vi "RS_SMBV100A.vi"(4 "error in":T15, 7 "Command":T16) -> (0 "error out":T15, 3 "Response":T13)   [LabVIEW 2018]
uses:
  MOKO_LabViewLibrary/MokoLowLevel/MokoLowLovelControl/MLLC_Command.ctl
  MOKO_LabViewLibrary/MokoLowLevel/MokoLowLovelControl/MLLC_Error.ctl
  MOKO_LabViewLibrary/MokoLowLevel/MokoLowLovelControl/MLLC_Mode.ctl
  MOKO_LabViewLibrary/MokoLowLevel/MokoLowLovelControl/MLLC_Response.ctl
  MOKO_LabViewLibrary/MokoLowLevel/MokoLowLovelControl/MLLC_ConnectCluster.ctl
  MOKO_LabViewLibrary/MokoLowLevel/MokoLowLovelControl/MLLC_InterfaceType.ctl
  MOKO_LabViewLibrary/MokoLowLevel/MokoLowLovelControl/MLLC_OpenedSession.ctl
  MOKO_LabViewLibrary/MokoLowLevel/MokoLowLovelControl/MLLC_InterfaceSettings.ctl
  MOKO_LabViewLibrary/MokoLowLevel/MokoLowLovelControl/MLLC_InterfaceKind.ctl
  data/RS_SMBV100A_DynamWaypoints.ctl
  data/RS_SMBV100A_DynamWaypoint.ctl
  MOKO_LabViewLibrary/MokoLowLevel/MokoLowLovelControl/MLLC_DriverName.ctl
  MOKO_LabViewLibrary/MokoLowLevel/MokoLowLovelControl/MLLC_ErrorCode.ctl
  MOKO_LabViewLibrary/MokoLowLevel/MokoLowLovelControl/MLLC_ResponseInit.ctl
  MOKO_LabViewLibrary/MokoLowLevel/MokoLowLovelControl/MLLC_Request.ctl
panel:
  in  "Request":T1="*IDN?"
  in  "ResponseInit":T2="SMBV100A"
  in  "Error Code":T3=5450
  in  "Driver Name":T4="RS_SMBV100A"
  in  "Settings":T12={"Connect"={"InterfaceType"=enum."VISA", "OpenedSession"="COM1", "InterfaceSettings"={"Interface"=enum."RS232", "EOS 4 read"=enum."LF (\\n)", "EOS 4 write"=enum."LF (\\n)", "TMO, ms"=10000, "Sett"=variant(cluster{"Baud Rate":u32, "Data Bits":u16, "Parity":u16, "Stop Bits":u16, "Flow Control":u16, "Eho":bool} {"Baud Rate"=75, "Data Bits"=0, "Parity"=0, "Stop Bits"=0, "Flow Control"=0, "Eho"=FALSE})}}, "GPS SCENARIO"="****************************** MOVEMENT FILE ******************************\nRESOLUTION: 50\nREFERENCE: 11.583333,48.150,500\nSTART: 0, 0, 0, 10\nSTAY: 10000\nLINE: 200, 0, 0\nLINE: 100, 0, 19.6\nLINE: 600, 0, 0\nLINE: 100, 0, -19.6\nARC: 1000, 500, 180\nLINE: -200, 0, 0\nLINE: -100, 0, 19.6\nLINE: -600, 0, 0\nLINE: -100, 0, -19.6\nARC: 0, 500, 180", "GLONASS SCENARIO"="****************************** MOVEMENT FILE ******************************\nRESOLUTION: 50\nREFERENCE: 11.583333,48.150,500\nSTART: 0, 0, 0, 10\nSTAY: 10000\nLINE: 200, 0, 0\nLINE: 100, 0, 19.6\nLINE: 600, 0, 0\nLINE: 100, 0, -19.6\nARC: 1000, 500, 180\nLINE: -200, 0, 0\nLINE: -100, 0, 19.6\nLINE: -600, 0, 0\nLINE: -100, 0, -19.6\nARC: 0, 500, 180", "GPS WAYPOINTS"=[], "GLONASS WAYPOINTS"=[], "GALILOE SCENARIO"="****************************** MOVEMENT FILE ******************************\nRESOLUTION: 50\nREFERENCE: 11.583333,48.150,500\nSTART: 0, 0, 0, 10\nSTAY: 10000\nLINE: 200, 0, 0\nLINE: 100, 0, 19.6\nLINE: 600, 0, 0\nLINE: 100, 0, -19.6\nARC: 1000, 500, 180\nLINE: -200, 0, 0\nLINE: -100, 0, 19.6\nLINE: -600, 0, 0\nLINE: -100, 0, -19.6\nARC: 0, 500, 180", "GALILEO WAYPOINTS"=[], "GPS WAYPOINTS STRING"="", "BASEBAND"="GPS", "BEIDOU SCENARIO"="****************************** MOVEMENT FILE ******************************\nRESOLUTION: 50\nREFERENCE: 11.583333,48.150,500\nSTART: 0, 0, 0, 10\nSTAY: 10000\nLINE: 200, 0, 0\nLINE: 100, 0, 19.6\nLINE: 600, 0, 0\nLINE: 100, 0, -19.6\nARC: 1000, 500, 180\nLINE: -200, 0, 0\nLINE: -100, 0, 19.6\nLINE: -600, 0, 0\nLINE: -100, 0, -19.6\nARC: 0, 500, 180", "QZSS SCENARIO"="****************************** MOVEMENT FILE ******************************\nRESOLUTION: 50\nREFERENCE: 11.583333,48.150,500\nSTART: 0, 0, 0, 10\nSTAY: 10000\nLINE: 200, 0, 0\nLINE: 100, 0, 19.6\nLINE: 600, 0, 0\nLINE: 100, 0, -19.6\nARC: 1000, 500, 180\nLINE: -200, 0, 0\nLINE: -100, 0, 19.6\nLINE: -600, 0, 0\nLINE: -100, 0, -19.6\nARC: 0, 500, 180", "BEIDOU WAYPOINTS"=[], "SSDK WAYPOINTS"=[]} {"SSDK WAYPOINTS"."Time" format="%<%.3X>T"; "SSDK WAYPOINTS"."Speed" format="%#.10g"; "SSDK WAYPOINTS"."Heigth" format="%#.10g"; "SSDK WAYPOINTS"."Longitude" format="%#.10g"; "SSDK WAYPOINTS"."Latitude" format="%#.10g"; "BEIDOU WAYPOINTS"."Time" format="%<%.3X>T"; "BEIDOU WAYPOINTS"."Speed" format="%#.10g"; "BEIDOU WAYPOINTS"."Heigth" format="%#.10g"; "BEIDOU WAYPOINTS"."Longitude" format="%#.10g"; "BEIDOU WAYPOINTS"."Latitude" format="%#.10g"; "GALILEO WAYPOINTS"."Time" format="%<%.3X>T"; "GALILEO WAYPOINTS"."Speed" format="%#.10g"; "GALILEO WAYPOINTS"."Heigth" format="%#.10g"; "GALILEO WAYPOINTS"."Longitude" format="%#.10g"; "GALILEO WAYPOINTS"."Latitude" format="%#.10g"; "GLONASS WAYPOINTS"."Time" format="%<%.3X>T"; "GLONASS WAYPOINTS"."Speed" format="%#.10g"; "GLONASS WAYPOINTS"."Heigth" format="%#.10g"; "GLONASS WAYPOINTS"."Longitude" format="%#.10g"; "GLONASS WAYPOINTS"."Latitude" format="%#.10g"; "GPS WAYPOINTS"."Time" format="%<%.3X>T"; "GPS WAYPOINTS"."Speed" format="%#.10g"; "GPS WAYPOINTS"."Heigth" format="%#.10g"; "GPS WAYPOINTS"."Longitude" format="%#.10g"; "GPS WAYPOINTS"."Latitude" format="%#.10g"}
  in  "Mode":T14=enum."Check"
  # "RS_SMBV100A"
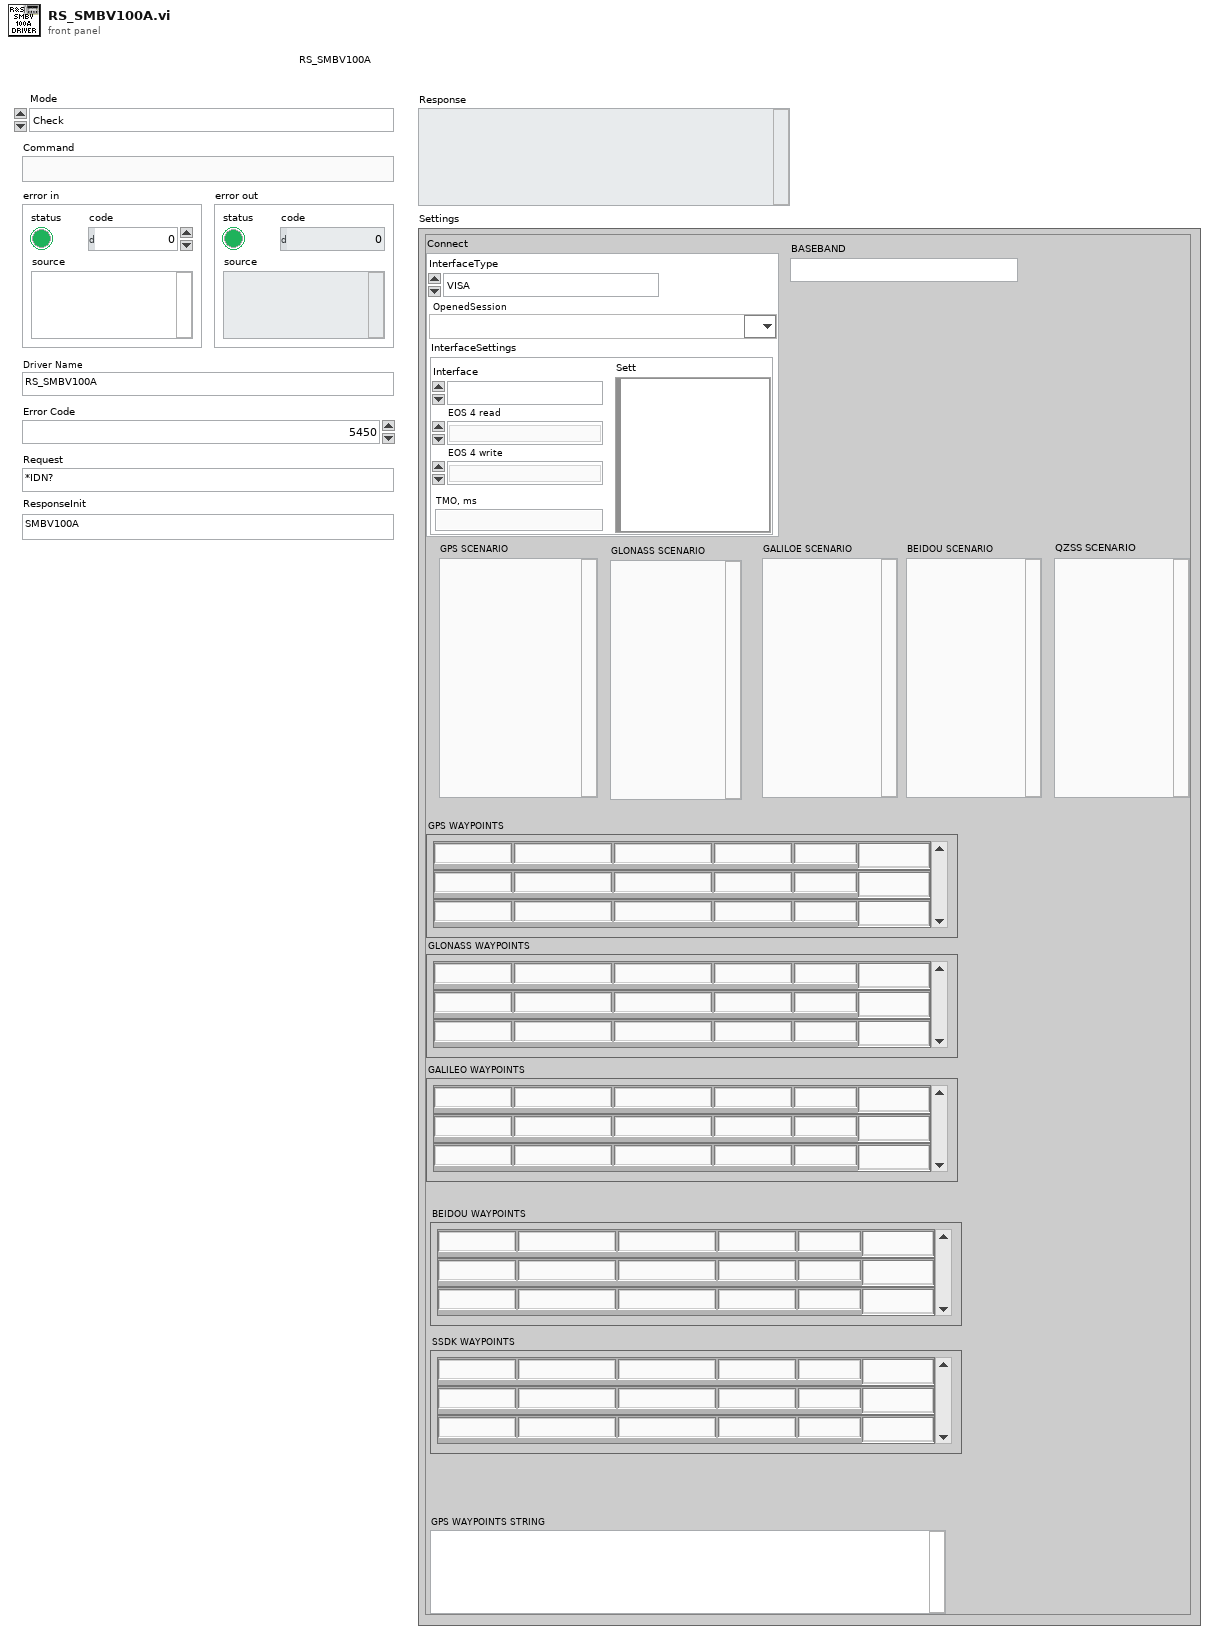
[diagram p1: front panel]
types:
  T1 = typedef "MLLC_Request.ctl" = string
  T2 = typedef "MLLC_ResponseInit.ctl" = string
  T3 = typedef "MLLC_ErrorCode.ctl" = u32
  T4 = typedef "MLLC_DriverName.ctl" = string
  T5 = typedef "MLLC_ConnectCluster.ctl" = cluster{"InterfaceType":T6, "OpenedSession":T7, "InterfaceSettings":T8}
  T6 = typedef "MLLC_InterfaceType.ctl" = enum16{"VISA", "Prologix USB-GPIB"}
  T7 = typedef "MLLC_OpenedSession.ctl" = refnum<visa-resource-name>
  T8 = typedef "MLLC_InterfaceSettings.ctl" = cluster{"Interface":T9, "EOS 4 read":enum16{"Default (=EOS 4 write)", "CR (\\r)", "LF (\\n)", "None"}, "EOS 4 write":enum16{"CR+LF (\\r\\n)", "CR (\\r)", "LF (\\n)", "None"}, "TMO, ms":i32, "Sett":variant}
  T9 = typedef "MLLC_InterfaceKind.ctl" = enum16{"RS232", "GPIB", "USB", "Ethernet", "another"}
  T10 = typedef "RS_SMBV100A_DynamWaypoints.ctl" = T11[]
  T11 = typedef "RS_SMBV100A_DynamWaypoint.ctl" = cluster{"Time":timestamp, "Latitude":ext, "Longitude":ext, "Heigth":dbl, "Speed":dbl, "Scenario":string}
  T12 = cluster{"Connect":T5, "GPS SCENARIO":string, "GLONASS SCENARIO":string, "GPS WAYPOINTS":T10, "GLONASS WAYPOINTS":T10, "GALILOE SCENARIO":string, "GALILEO WAYPOINTS":T10, "GPS WAYPOINTS STRING":string, "BASEBAND":string, "BEIDOU SCENARIO":string, "QZSS SCENARIO":string, "BEIDOU WAYPOINTS":T10, "SSDK WAYPOINTS":T10}
  T13 = typedef "MLLC_Response.ctl" = string
  T14 = typedef "MLLC_Mode.ctl" = enum16{"get", "set", "close", "Init", "Check"}
  T15 = typedef "MLLC_Error.ctl" = errorcluster
  T16 = typedef "MLLC_Command.ctl" = string
  T17 = enum16{"open", "replace", "create", "open or create", "replace or create", "replace or create with confirmation"}
  T18 = typedef "RS_SMBV100A_Parsing Satelite.ctl" = cluster{"Time":dbl[], "Sat":dbl[], "State":dbl[], "NUMBERINSKY":dbl[], "STANDART":string[]}
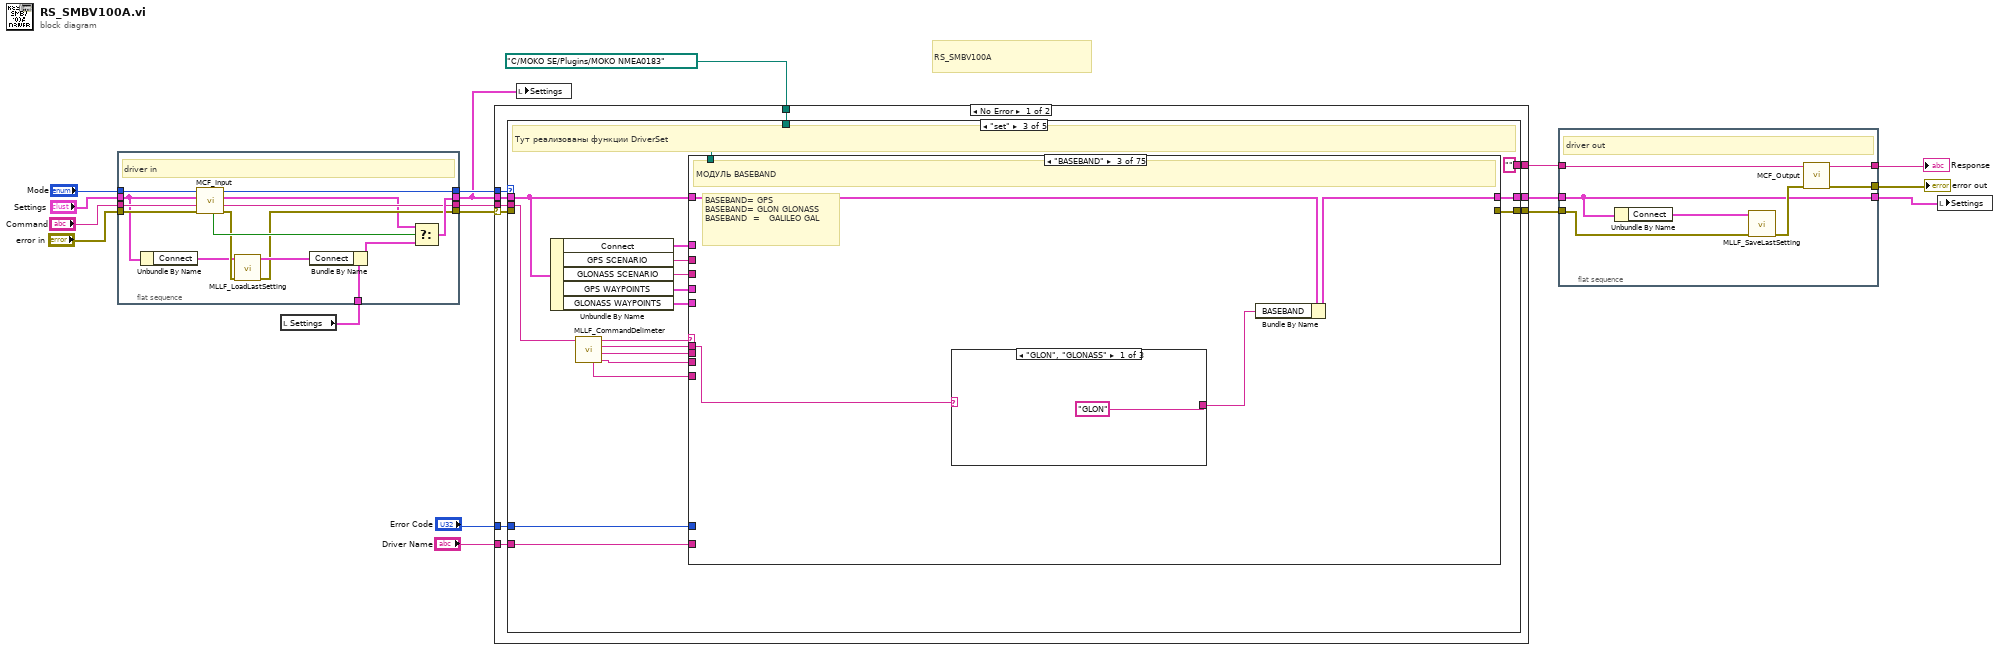
[diagram p0: block diagram]
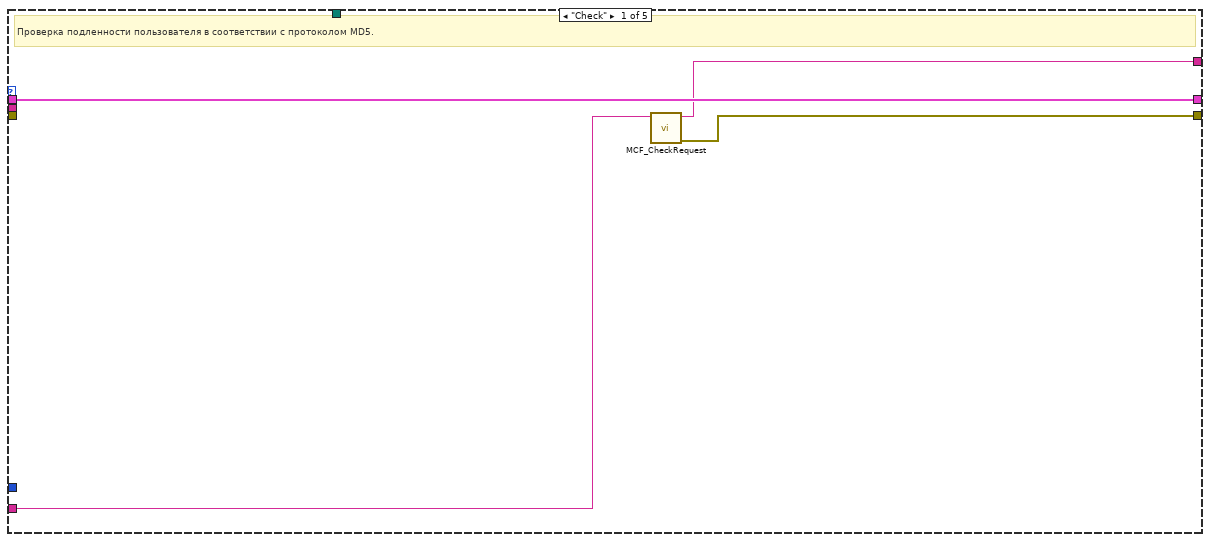
[diagram p2: hidden frame]
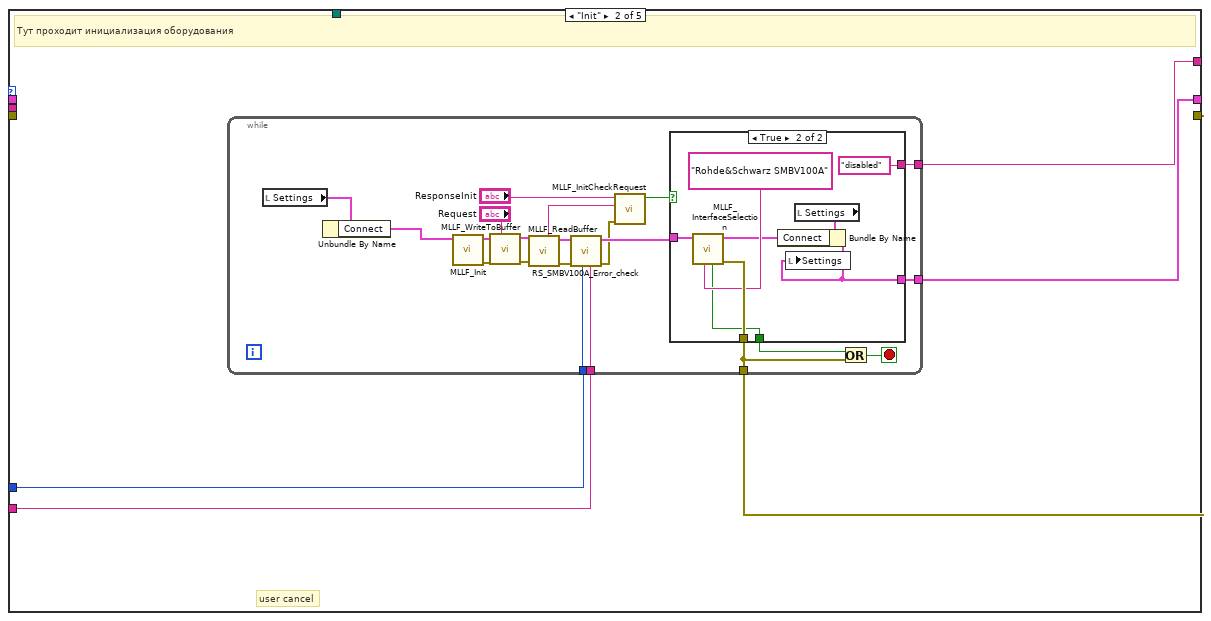
[diagram p3: hidden frame]
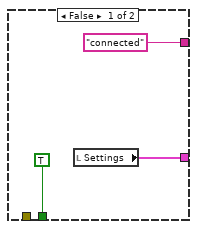
[diagram p4: hidden frame]
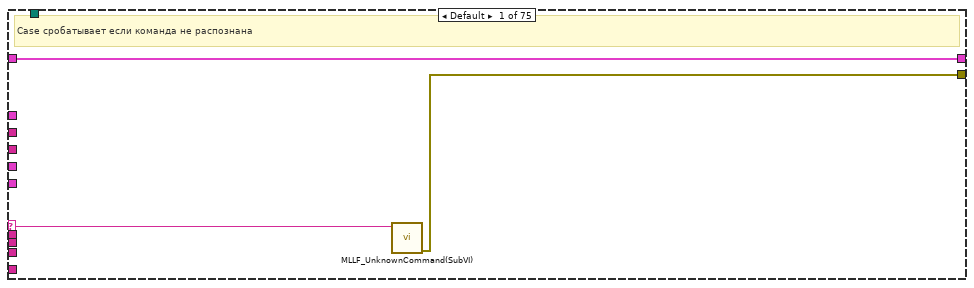
[diagram p5: hidden frame]
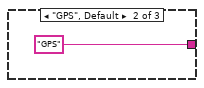
[diagram p7: hidden frame]
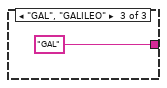
[diagram p8: hidden frame]
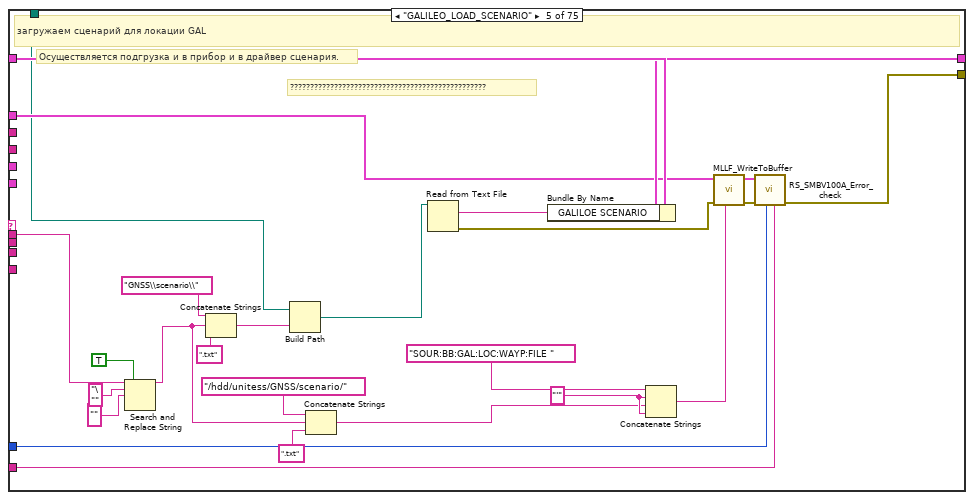
[diagram p10: hidden frame]
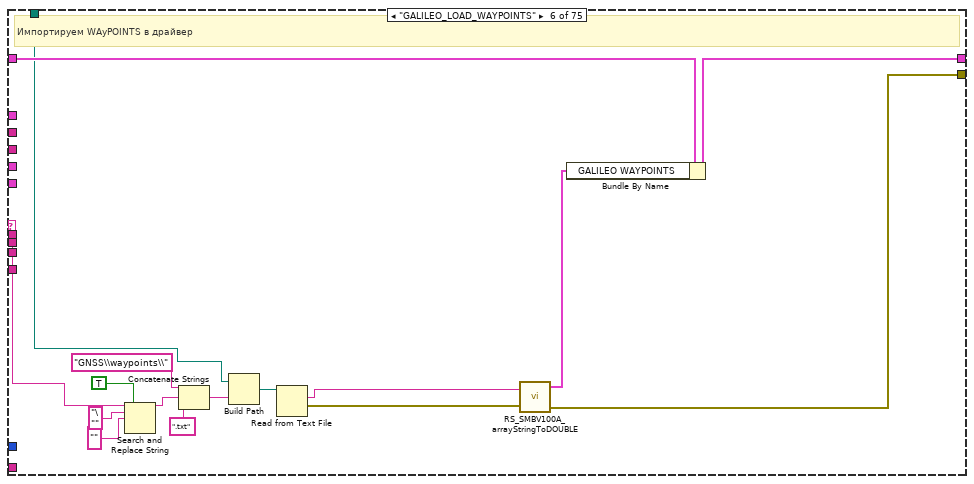
[diagram p11: hidden frame]
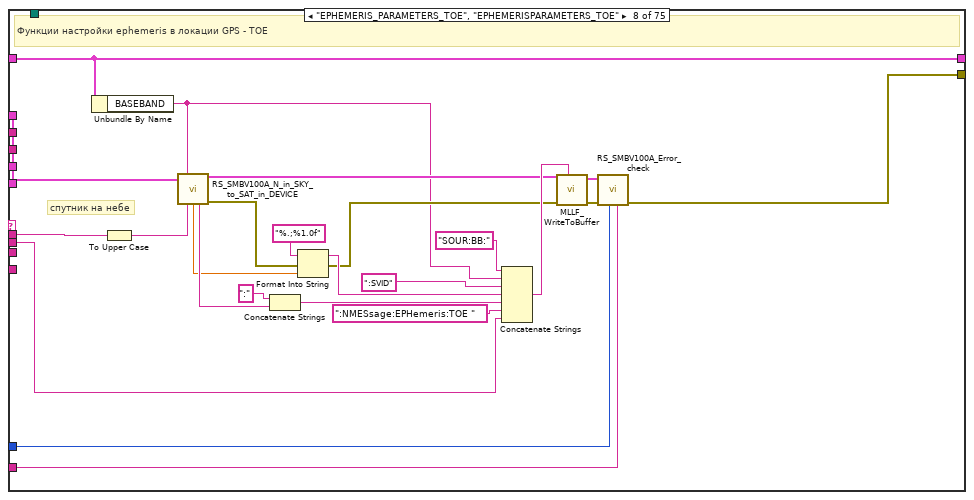
[diagram p13: hidden frame]
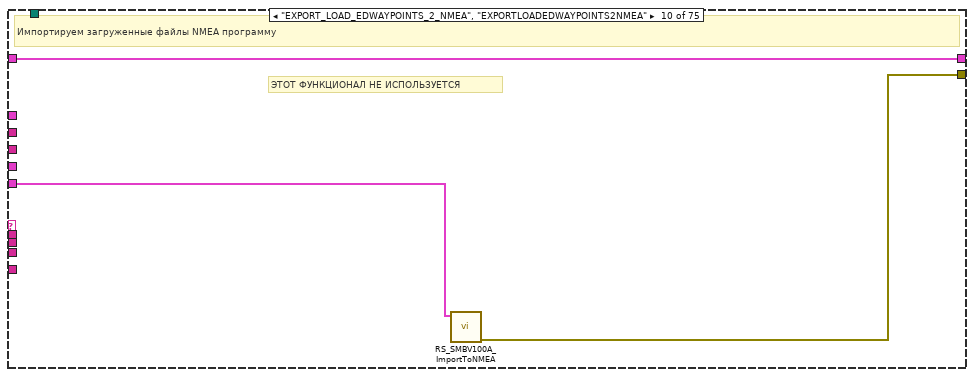
[diagram p15: hidden frame]
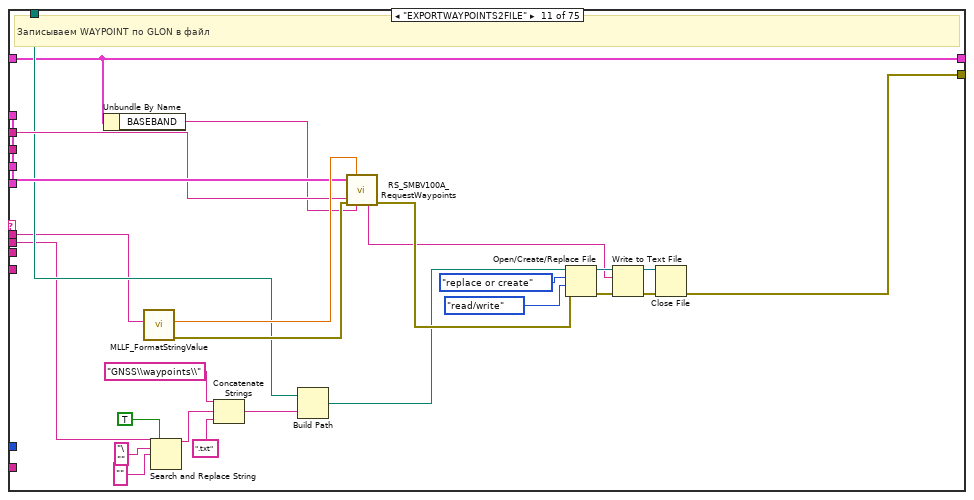
[diagram p16: hidden frame]
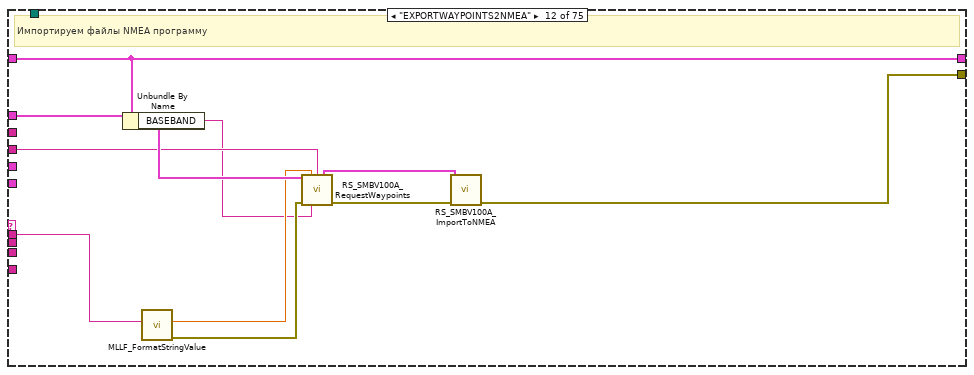
[diagram p17: hidden frame]
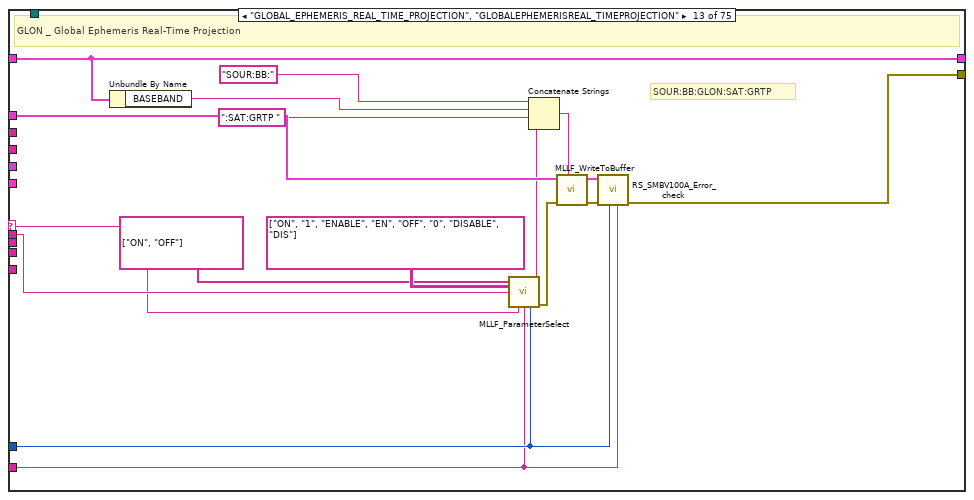
[diagram p18: hidden frame]
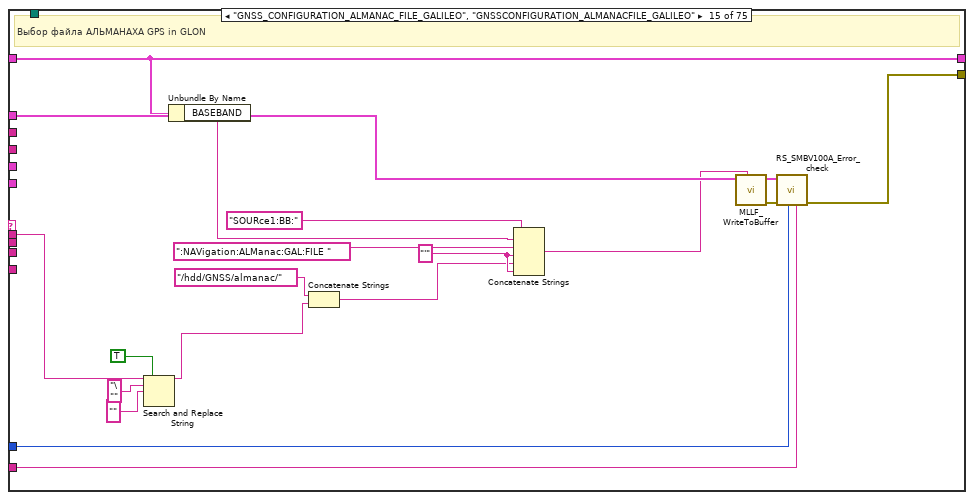
[diagram p20: hidden frame]
diagram:
  # "RS_SMBV100A"
  n1 = flat-sequence {
    tunnel: [w22] -> w3
    tunnel: [w32] -> w5
    tunnel: [w24] -> w2
    tunnel: "Command" -> [w25]
    tunnel: "Mode" -> [w27]
    tunnel: "Settings" -> [w20]
    tunnel: [w29] -> w4
    tunnel: w1 -> [w28]
    tunnel: "error in" -> [w21]
    frame #0 {
      # "driver in"
      n2 = Unbundle By Name(w20) -> ("Connect"=w19:T5)
      n3 = call "MCF_Input.vi"("Error In"=w21, "Command in"=w25, "Mode in"=w27) -> ("Error Out"=w23:errorcluster, "Command out"=w24:string, "Mode out"=w32:T14, "Boolean"=w26:bool)  [unwired: 5 in]
      n4 = call "MLLF_LoadLastSetting.vi"("Error In"=w23, "DriverConnectCluster in"=w19) -> ("Error Out"=w22:errorcluster, "DriverConnectCluster out"=w30:T5)  [unwired: 8 in]
      n5 = Bundle By Name(cluster=w28, "Connect"=w30) -> (w31:T12)
      n6 = Select(t=w20, s=w26, f=w31) -> (s? t:f=w29:T12)
    }
  }
  n7 = local read "Settings"() -> (w1:T12)
  n8 = case shown="No Error" w3 {
    selector: w3 -> [w39 w2026]
    tunnel: [w41 w2026] -> w13
    tunnel: w5 -> [w33 _]
    tunnel: [w42 _] -> w15
    tunnel: w2 -> [w40 _]
    tunnel: w4 -> [w36 w2025]
    tunnel: "Error Code" -> [w38 _]
    tunnel: "Driver Name" -> [w37 _]
    tunnel: [w35 w2025] -> w14
    tunnel: path "C:/MOKO SE/Plugins/MOKO NMEA0183" ("base path") -> [w34 _]
    frame No Error {
      n9 = case shown="\"set\"" w33 {
        tunnel: [w44 w47 "" ("Output String") w1143 "" ("Output String")] -> w42
        tunnel: [w43 w48 w100 w1142 w2023] -> w41
        tunnel: w40 -> [_ _ w101 w1155 _]
        tunnel: w39 -> [_ _ _ _ _]
        tunnel: w38 -> [_ w51 w99 w1152 _]
        tunnel: w37 -> [w45 w50 w96 w1151 _]
        tunnel: w36 -> [w46 _ w98 w1154 w2022]
        tunnel: [w46 w49 w97 w1153 w2022] -> w35
        tunnel: w34 -> [_ _ w95 _ _]
        frame "Check" {
          # "Проверка подленности пользователя в соответствии с протоколом MD5."
          n10 = call "MCF_CheckRequest.vi"("Driver Name"=w45) -> ("Error Out"=w43:errorcluster, "Output String"=w44:string)  [unwired: 9 in]
        }
        frame "Init" {
          # "user cancel"
          # "Тут проходит инициализация оборудования"
          n11 = while {
            tunnel: [w64] -> w48
            tunnel: w51 -> [w61]
            tunnel: w50 -> [w60]
            tunnel: [w57] -> w49
            tunnel: [w56] -> w47
            stop <- w63 stop-if-true
            n12 = local read "Settings"() -> (w67:T12)
            n13 = Unbundle By Name(w67) -> ("Connect"=w68:T5)
            n14 = call "MLLF_Init.vi"("DriverConnect in"=w68) -> ("Error Out"=w70:errorcluster, "DriverConnect out"=w69:T5)  [unwired: 7 in]
            n15 = call "MLLF_WriteToBuffer.vi"("String"="Request", "error in"=w70, "DriverConnect in"=w69) -> ("error out"=w72:T15, "DriverConnect out"=w71:T5)  [unwired: 5 in]
            n16 = call "MLLF_ReadBuffer.vi"("Error In"=w72, "DriverConnect in"=w71) -> ("Error Out"=w58:errorcluster, "DriverConnect out"=w59:T5, "String"=w54:string)  [unwired: 6 in]
            n17 = call "RS_SMBV100A_Error_check.vi"("Driver Name"=w60, "Error Code"=w61, "Error In"=w58, "DriverConnect in"=w59) -> ("Error Out"=w53:errorcluster, "DriverConnect out"=w62:T5)  [unwired: 6 in]
            n18 = call "MLLF_InitCheckRequest.vi"("error in (no error)"=w53, "Answer"=w54, "Response Init"="ResponseInit") -> ("Design"=w52:bool)  [unwired: 5 in, 3 out]
            n19 = case shown="True" w52 {
              tunnel: w62 -> [_ w82]
              tunnel: [TRUE w76] -> w65
              tunnel: [_ w83] -> w64
              tunnel: [w74 w78] -> w57
              tunnel: ["connected" "disabled"] -> w56
              frame False {
                n20 = local read "Settings"() -> (w74:T12)
              }
              frame True {
                n21 = call "MLLF_InterfaceSelection.vi"("Driver Name"="Rohde&Schwarz SMBV100A" ("String"), "DriverConnect in"=w82) -> ("error out"=w83:T15, "DriverConnect out"=w80:T5, "stop init?"=w76:bool)  [unwired: 5 in, 2 out]
                n22 = local read "Settings"() -> (w79:T12)
                n23 = Bundle By Name(cluster=w79, "Connect"=w80) -> (w78:T12)
                n24 = local write "Settings"(w78) -> ()
              }
            }
            n25 = Or(x=w65, y=w64) -> (x .or. y?=w63:bool)
          }
        }
        frame "set" {
          # "Тут реализованы функции DriverSet"
          n26 = Unbundle By Name(w98) -> ("Connect"=w93:T5, "GPS SCENARIO"=w92:string, "GLONASS SCENARIO"=w91:string, "GPS WAYPOINTS"=w90:T10, "GLONASS WAYPOINTS"=w89:T10)
          n27 = call "MLLF_CommandDelimeter.vi"("command with param"=w101) -> ("param 3"=w85:string, "param 2"=w86:string, "param 1"=w87:string, "command"=w88:string, "Spit delimetre"=w84:string)  [unwired: 6 in]
          n28 = case shown="\"BASEBAND\"" w88 {
            selector: w88 -> [w103 _ _ _ _ _ _ _ _ _ _ _ w221 _ _ _ _ _ _ _ w355 w372 w387 _ _ _ w447 _ w486 w503 w522 _ _ w575 _ _ _ w618 _ w655 _ w687 w703 _ _ w738 _ _ w807 _ w825 w842 w859 w876 _ _ w912 _ _ _ _ w975 _ _ _ _ _ _ _ _ _ w1080 _ _ _]
            tunnel: [w102 _ _ _ w129 w147 _ w176 _ w183 w199 w218 w229 _ w252 w271 w290 w309 w328 w347 w369 w386 w403 w419 w437 _ w455 w480 w494 w511 w536 w551 w564 w583 _ w603 w612 w626 w650 w665 w681 w696 w712 w726 _ w752 w773 w804 w815 _ w833 w850 w868 w884 w900 _ w920 w935 w947 _ w969 w991 _ w1006 w1025 _ w1040 w1047 w1056 w1064 w1072 w1082 w1100 w1108 w1118] -> w100
            tunnel: w99 -> [_ _ _ _ w128 _ _ w180 _ _ _ _ w234 _ w257 w276 w295 w314 w333 w352 w353 w370 w388 w418 _ _ w460 w485 w499 w516 w520 w556 w569 w573 _ w599 w617 w631 w654 w670 w686 w701 w717 w731 _ w736 w775 w806 w820 _ w838 w855 w872 w889 w905 _ w910 w934 w949 _ w974 w978 _ w1005 _ _ w1045 w1049 w1058 w1066 w1074 w1087 w1105 w1113 w1119]
            tunnel: w98 -> [w104 w105 w109 w113 w138 w151 w156 w163 w181 w184 w188 w212 w228 w238 w241 w261 w280 w297 w316 w335 w359 w376 w393 w428 w441 w446 w454 w469 w488 w505 w524 w539 w560 w577 w590 w594 w607 w620 w639 w657 w673 w690 w704 w722 w735 w740 w755 w778 w809 w824 w827 w844 w862 w878 w894 w909 w914 w930 w942 w953 w954 w979 w992 w1015 w1028 w1032 w1046 w1055 w1063 w1071 w1079 w1092 w1106 w1114 w1117]
            tunnel: [w104 w105 w108 w113 w137 w150 w156 w163 w181 w184 w188 w212 w228 w238 w241 w261 w280 w297 w316 w335 w359 w376 w393 w427 w440 w446 w454 w469 w488 w505 w524 w539 w560 w577 w590 w594 w607 w620 w639 w657 w673 w690 w704 w722 w735 w740 w755 w778 w809 w824 w827 w844 w862 w878 w894 w909 w914 w930 w942 w953 w954 w979 w992 w1014 w1027 w1032 w1046 w1055 w1063 w1071 w1079 w1092 w1106 w1114 w1116] -> w97
            tunnel: w93 -> [_ _ _ _ w131 _ _ w175 _ _ w208 w220 w232 _ w255 w274 w293 w312 w331 w350 w363 w380 w397 w421 _ _ w458 w483 w497 w514 w530 w554 w567 w584 _ w606 w615 w629 w649 w668 w684 w699 w715 w729 _ w748 w772 w803 w818 _ w836 w853 w871 w887 w903 _ w921 w936 w950 _ w972 w987 _ w1008 _ _ w1043 w1050 w1059 w1067 w1075 w1085 w1103 w1111 _]
            tunnel: w96 -> [_ _ _ _ w127 _ _ w179 _ _ _ _ w233 _ w256 w275 w294 w313 w332 w351 w354 w371 w389 w417 _ _ w459 w484 w498 w515 w521 w555 w568 w574 _ w600 w616 w630 w653 w669 w685 w700 w716 w730 _ w737 w774 w805 w819 _ w837 w854 w860 w888 w904 _ w911 w933 w948 _ w973 w977 _ w1004 _ _ w1044 w1048 w1057 w1065 w1073 w1086 w1104 w1112 w1120]
            tunnel: w87 -> [_ _ w106 _ w116 w141 _ w158 _ _ w186 w217 w222 _ w243 w263 w282 w300 w319 w338 w356 w373 w390 w406 w431 _ w448 w466 w487 w504 w523 w541 w557 w576 _ w591 _ w619 w636 w656 w672 _ _ w719 _ w739 w759 w783 w808 _ w826 w843 w861 w877 w893 _ w913 w927 _ _ w960 w976 _ w994 w1020 _ w1036 _ _ _ _ w1081 w1096 _ w1115]
            tunnel: w92 -> [_ _ _ _ _ _ _ _ _ _ w194 _ _ _ _ _ _ _ _ _ _ _ _ _ _ _ _ _ _ _ _ _ _ _ _ _ _ _ _ _ _ _ _ _ _ _ _ _ _ _ _ _ _ _ _ _ _ _ _ _ _ _ _ _ _ _ _ _ _ _ _ _ _ _ _]
            tunnel: w91 -> [_ _ _ _ _ _ _ _ _ _ _ w214 _ _ _ _ _ _ _ _ _ _ _ _ _ _ _ _ _ _ _ _ _ _ _ _ _ _ _ _ _ _ _ _ _ _ _ _ _ _ _ _ _ _ _ _ _ _ _ _ _ _ _ _ _ _ _ _ _ _ _ _ _ _ _]
            tunnel: w90 -> [_ _ _ _ _ _ _ _ _ _ _ _ _ _ _ _ _ _ _ _ _ _ _ _ _ _ _ _ _ _ _ _ _ _ _ _ _ _ _ _ _ _ _ _ _ _ _ _ _ _ _ _ _ _ _ _ _ _ _ _ _ _ _ _ _ _ _ _ _ _ _ _ _ _ _]
            tunnel: w89 -> [_ _ _ _ _ _ _ _ _ w182 _ _ _ _ _ _ _ _ _ _ _ _ _ _ _ _ _ _ _ _ _ _ _ _ _ _ _ _ _ _ _ _ _ _ _ _ _ _ _ _ _ _ _ _ _ _ _ _ _ _ _ _ _ _ _ _ _ _ _ _ _ _ _ _ _]
            tunnel: w95 -> [_ _ _ _ w114 w140 _ _ _ _ w189 _ _ _ _ _ _ _ _ _ _ _ _ w404 w430 _ _ _ _ _ _ _ _ _ _ _ _ _ _ _ _ _ _ _ _ _ _ _ _ _ _ _ _ _ _ _ _ _ _ _ _ _ _ w993 w1017 _ _ _ _ _ _ _ _ _ _]
            tunnel: w86 -> [_ _ _ _ _ _ _ w157 _ _ w185 _ _ _ _ _ _ _ _ _ _ _ _ _ _ _ _ w465 _ _ _ _ _ _ _ _ _ _ w635 _ _ _ _ _ _ _ _ _ _ _ _ _ _ _ _ _ _ _ _ _ _ _ _ _ _ _ _ _ _ _ _ _ _ _ _]
            tunnel: w85 -> [_ _ _ _ _ _ _ _ _ _ _ _ _ _ _ _ _ _ _ _ _ _ _ _ _ _ _ w464 _ _ _ _ _ _ _ _ _ _ _ _ _ _ _ _ _ _ _ _ _ _ _ _ _ _ _ _ _ _ _ _ _ _ _ _ _ _ _ _ _ _ _ _ _ _ _]
            tunnel: w84 -> [_ _ _ _ _ _ _ _ _ _ _ _ _ _ _ _ _ _ _ _ _ _ _ _ _ _ _ _ _ _ _ _ _ _ _ _ _ _ _ _ _ _ _ _ _ _ _ _ _ _ _ _ _ _ _ _ _ _ _ _ _ _ _ _ _ _ _ _ _ _ _ _ _ w1107 _]
            frame Default {
              # "Case сробатывает если команда не распознана"
              n29 = call "MLLF_UnknownCommand(SubVI).vi"("Unknown command"=w103) -> ("error out"=w102:errorcluster)  [unwired: 10 in]
            }
            frame "----- BASEBAND -----" {
              # "МОДУЛЬ BASEBAND"
            }
            frame "BASEBAND" {
              # "BASEBAND= GPS\nBASEBAND= GLON GLONASS\nBASEBAND  =   GALILEO GAL"
              # "МОДУЛЬ BASEBAND"
              n30 = case shown="\"GLON\", \"GLONASS\"" w106 {
                tunnel: ["GLON" ("regular expression") "GPS" "GAL" ("regular expression")] -> w107
                frame "GLON", "GLONASS" {
                }
                frame "GPS", Default {
                }
                frame "GAL", "GALILEO" {
                }
              }
              n31 = Bundle By Name(cluster=w109, "BASEBAND"=w107) -> (w108:T12)
            }
            frame "----GALILEO BASEBAND----" {
            }
            frame "GALILEO_LOAD_SCENARIO" {
              w135 = "'" ("string")
              # "?????????????????????????????????????????????????"
              # "Осуществляется подгрузка и в прибор и в драйвер сценария."
              # "загружаем сценарий для локации GAL"
              n32 = Search and Replace String(replace all?=TRUE, input string=w116, search string="\"", replace string="") -> (result string=w115:string)  [unwired: 4 in, 3 out]
              n33 = Concatenate Strings("GNSS\\scenario\\", w115, ".txt") -> (w125:string)
              n34 = Build Path(base path=w114, name or relative path=w125) -> (appended path=w120:path)
              n35 = Concatenate Strings("/hdd/unitess/GNSS/scenario/", w115, ".txt") -> (w121:string)
              n36 = Read from Text File(file (use dialog)=w120) -> (text=w139:string, error out=w130:errorcluster)  [unwired: 3 in, 2 out]
              n37 = Bundle By Name(cluster=w138, "GALILOE SCENARIO"=w139) -> (w137:T12)
              n38 = Concatenate Strings("SOUR:BB:GAL:LOC:WAYP:FILE " ("string"), w135, w121, w135) -> (w132:string)
              n39 = call "MLLF_WriteToBuffer.vi"("String"=w132, "error in"=w130, "DriverConnect in"=w131) -> ("error out"=w133:T15, "DriverConnect out"=w134:T5)  [unwired: 5 in]
              n40 = call "RS_SMBV100A_Error_check.vi"("Driver Name"=w127, "Error Code"=w128, "Error In"=w133, "DriverConnect in"=w134) -> ("Error Out"=w129:errorcluster)  [unwired: 6 in, 1 out]
            }
            frame "GALILEO_LOAD_WAYPOINTS" {
              # "Импортируем WAyPOINTS в драйвер"
              n41 = Search and Replace String(replace all?=TRUE, input string=w141, search string="\"", replace string="") -> (result string=w142:string)  [unwired: 4 in, 3 out]
              n42 = Concatenate Strings("GNSS\\waypoints\\", w142, ".txt") -> (w154:string)
              n43 = Build Path(base path=w140, name or relative path=w154) -> (appended path=w152:path)
              n44 = Read from Text File(file (use dialog)=w152) -> (text=w149:string, error out=w148:errorcluster)  [unwired: 3 in, 2 out]
              n45 = call "RS_SMBV100A_arrayStringToDOUBLE.vi"("string"=w149, "error in"=w148) -> ("Dynam waypoints"=w146:T10, "error out"=w147:errorcluster)  [unwired: 1 in]
              n46 = Bundle By Name(cluster=w151, "GALILEO WAYPOINTS"=w146) -> (w150:T12)
            }
            frame "---- GLONASS BASEBAND -----" {
              # "Функции настройки в локации GLONASS"
            }
            frame "EPHEMERIS_PARAMETERS_TOE", "EPHEMERISPARAMETERS_TOE" {
              # "спутник на небе"
              # "Функции настройки ephemeris в локации GPS - TOE"
              n47 = Unbundle By Name(w163) -> ("BASEBAND"=w160:string)
              n48 = To Upper Case(1:w158) -> (0:w159:string)
              n49 = call "RS_SMBV100A_N_in_SKY_to_SAT_in_DEVICE.vi"("DriverConnect in"=w175, "BASEBAND"=w160, "String Value"=w159) -> ("GNSS"=w167:string, "DriverConnect out"=w171:T5, "SATINSKY_for_DEVICE"=w164:dbl, "Error Out"=w170:errorcluster)  [unwired: 8 in, 1 out]
              n50 = Concatenate Strings(":" ("regular expression"), w167) -> (w166:string)
              n51 = Format Into String(format string="%.;%1.0f" ("format"), error in=w170, w164) -> (resulting string=w173:string, error out=w169:errorcluster)  [unwired: 1 in]
              n52 = Concatenate Strings("SOUR:BB:" ("regular expression"), w160, ":SVID" ("regular expression"), w173, w166, ":NMESsage:EPHemeris:TOE " ("regular expression"), w157) -> (w172:string)
              n53 = call "MLLF_WriteToBuffer.vi"("String"=w172, "error in"=w169, "DriverConnect in"=w171) -> ("error out"=w177:T15, "DriverConnect out"=w178:T5)  [unwired: 5 in]
              n54 = call "RS_SMBV100A_Error_check.vi"("Driver Name"=w179, "Error Code"=w180, "Error In"=w177, "DriverConnect in"=w178) -> ("Error Out"=w176:errorcluster)  [unwired: 6 in, 1 out]
            }
            frame "---------------------------- EXPORT ----------------------------------" {
            }
            frame "EXPORT_LOAD_EDWAYPOINTS_2_NMEA", "EXPORTLOADEDWAYPOINTS2NMEA" {
              # "ЭТОТ ФУНКЦИОНАЛ НЕ ИСПОЛЬЗУЕТСЯ"
              # "Импортируем загруженные файлы NMEA программу"
              n55 = call "RS_SMBV100A_ImportToNMEA.vi"("Dynam waypoints"=w182) -> ("error out"=w183:errorcluster)  [unwired: 10 in]
            }
            frame "EXPORTWAYPOINTS2FILE" {
              # "Записываем WAYPOINT по GLON в файл"
              n56 = Unbundle By Name(w188) -> ("BASEBAND"=w187:string)
              n57 = call "MLLF_FormatStringValue.vi"("String Value"=w186) -> ("error out"=w209:T15, "number"=w210:dbl)  [unwired: 8 in, 1 out]
              n58 = Search and Replace String(replace all?=TRUE, input string=w185, search string="\"", replace string="") -> (result string=w190:string)  [unwired: 4 in, 3 out]
              n59 = Concatenate Strings("GNSS\\waypoints\\", w190, ".txt") -> (w197:string)
              n60 = Build Path(base path=w189, name or relative path=w197) -> (appended path=w196:path)
              n61 = call "RS_SMBV100A_RequestWaypoints.vi"("DriverConnect in"=w208, "scenario time, c"=w210, "Error In"=w209, "BASEBAND"=w187, "Scenario in"=w194) -> ("Waypoints, txt"=w200:string, "Error Out"=w201:errorcluster)  [unwired: 7 in, 2 out]
              n62 = Open/Create/Replace File(file path (use dialog)=w196, error in=w201, operation (0:open)=T17."replace or create", access (0:read/write)=enum16{"read/write", "read-only", "write-only"}."read/write") -> (refnum out=w205:refnum<file>, error out=w202:errorcluster)  [unwired: 2 in, 1 out]
              n63 = Write to Text File(file (use dialog)=w205, text=w200, error in=w202) -> (refnum out=w203:refnum<file>, error out=w204:errorcluster)  [unwired: 1 in, 1 out]
              n64 = Close File(refnum=w203, error in=w204) -> (error out=w199:errorcluster)  [unwired: 1 out]
            }
            frame "EXPORTWAYPOINTS2NMEA" {
              # "Импортируем файлы NMEA программу"
              n65 = Unbundle By Name(w212) -> ("BASEBAND"=w211:string)
              n66 = call "MLLF_FormatStringValue.vi"("String Value"=w217) -> ("error out"=w215:T15, "number"=w216:dbl)  [unwired: 8 in, 1 out]
              n67 = call "RS_SMBV100A_RequestWaypoints.vi"("DriverConnect in"=w220, "scenario time, c"=w216, "Error In"=w215, "BASEBAND"=w211, "Scenario in"=w214) -> ("Dynam waypoints"=w213:T10, "Error Out"=w219:errorcluster)  [unwired: 7 in, 2 out]
              n68 = call "RS_SMBV100A_ImportToNMEA.vi"("error in"=w219, "Dynam waypoints"=w213) -> ("error out"=w218:errorcluster)  [unwired: 9 in]
            }
            frame "GLOBAL_EPHEMERIS_REAL_TIME_PROJECTION", "GLOBALEPHEMERISREAL_TIMEPROJECTION" {
              # "SOUR:BB:GLON:SAT:GRTP"
              # "GLON _ Global Ephemeris Real-Time Projection"
              n69 = Unbundle By Name(w228) -> ("BASEBAND"=w226:string)
              n70 = call "MLLF_ParameterSelect.vi"("Command to equipment"=string[] ["ON", "OFF"], "Names"=string[][] [["ON", "1", "ENABLE", "EN"], ["OFF", "0", "DISABLE", "DIS"]], "Input"=w222, "Command"=w221, "Driver Name"=w233, "Error Code"=w234) -> ("Choice"=w224:string, "Error Out"=w235:errorcluster)  [unwired: 8 in]
              n71 = Concatenate Strings("SOUR:BB:", w226, ":SAT:GRTP ", w224) -> (w223:string)
              n72 = call "MLLF_WriteToBuffer.vi"("String"=w223, "error in"=w235, "DriverConnect in"=w232) -> ("error out"=w230:T15, "DriverConnect out"=w231:T5)  [unwired: 5 in]
              n73 = call "RS_SMBV100A_Error_check.vi"("Driver Name"=w233, "Error Code"=w234, "Error In"=w230, "DriverConnect in"=w231) -> ("Error Out"=w229:errorcluster)  [unwired: 6 in, 1 out]
            }
            frame "---------------------- GNSS_CONFIGURATION ---------------------------------" {
            }
            frame "GNSS_CONFIGURATION_ALMANAC_FILE_GALILEO", "GNSSCONFIGURATION_ALMANACFILE_GALILEO" {
              w249 = "'" ("string")
              # "Выбор файла АЛЬМАНАХА GPS in GLON"
              n74 = Search and Replace String(replace all?=TRUE, input string=w243, search string="\"", replace string="") -> (result string=w242:string)  [unwired: 4 in, 3 out]
              n75 = Unbundle By Name(w241) -> ("BASEBAND"=w240:string)
              n76 = Concatenate Strings("/hdd/GNSS/almanac/" ("string"), w242) -> (w247:string)
              n77 = Concatenate Strings("SOURce1:BB:" ("string"), w240, ":NAVigation:ALManac:GAL:FILE " ("string"), w249, w247, w249) -> (w250:string)
              n78 = call "MLLF_WriteToBuffer.vi"("String"=w250, "DriverConnect in"=w255) -> ("error out"=w253:T15, "DriverConnect out"=w254:T5)  [unwired: 6 in]
              n79 = call "RS_SMBV100A_Error_check.vi"("Driver Name"=w256, "Error Code"=w257, "Error In"=w253, "DriverConnect in"=w254) -> ("Error Out"=w252:errorcluster)  [unwired: 6 in, 1 out]
            }
            frame "GNSS_CONFIGURATION_ALMANAC_FILE_GLONASS", "GNSSCONFIGURATION_ALMANACFILE_GLONASS" {
              w269 = "'" ("string")
              # "Выбор файла АЛЬМАНАХА Glonas in GLON"
              n80 = Search and Replace String(replace all?=TRUE, input string=w263, search string="\"", replace string="") -> (result string=w262:string)  [unwired: 4 in, 3 out]
              n81 = Unbundle By Name(w261) -> ("BASEBAND"=w260:string)
              n82 = Concatenate Strings("/hdd/GNSS/almanac/" ("string"), w262) -> (w267:string)
              n83 = Concatenate Strings("SOURce1:BB:" ("string"), w260, ":NAVigation:ALManac:GLON:FILE " ("string"), w269, w267, w269) -> (w270:string)
              n84 = call "MLLF_WriteToBuffer.vi"("String"=w270, "DriverConnect in"=w274) -> ("error out"=w272:T15, "DriverConnect out"=w273:T5)  [unwired: 6 in]
              n85 = call "RS_SMBV100A_Error_check.vi"("Driver Name"=w275, "Error Code"=w276, "Error In"=w272, "DriverConnect in"=w273) -> ("Error Out"=w271:errorcluster)  [unwired: 6 in, 1 out]
            }
            frame "GNSS_CONFIGURATION_ALMANAC_FILE_GPS", "GNSSCONFIGURATION_ALMANACFILE_GPS" {
              w288 = "'" ("string")
              # "Выбор файла АЛЬМАНАХА GPS in GLON"
              n86 = Search and Replace String(replace all?=TRUE, input string=w282, search string="\"", replace string="") -> (result string=w281:string)  [unwired: 4 in, 3 out]
              n87 = Concatenate Strings("/hdd/GNSS/almanac/" ("string"), w281) -> (w286:string)
              n88 = Unbundle By Name(w280) -> ("BASEBAND"=w278:string)
              n89 = Concatenate Strings("SOURce1:BB:" ("string"), w278, ":NAVigation:ALManac:GPS:FILE " ("string"), w288, w286, w288) -> (w289:string)
              n90 = call "MLLF_WriteToBuffer.vi"("String"=w289, "DriverConnect in"=w293) -> ("error out"=w291:T15, "DriverConnect out"=w292:T5)  [unwired: 6 in]
              n91 = call "RS_SMBV100A_Error_check.vi"("Driver Name"=w294, "Error Code"=w295, "Error In"=w291, "DriverConnect in"=w292) -> ("Error Out"=w290:errorcluster)  [unwired: 6 in, 1 out]
            }
            frame "GNSS_CONFIGURATION_RINEX_FILE_GAL", "GNSSCONFIGURATION_RINEXFILE_GAL" {
              w306 = "'" ("string")
              # "Выбор файла GPS RINEX GLON"
              n92 = Search and Replace String(replace all?=TRUE, input string=w300, search string="\"", replace string="") -> (result string=w299:string)  [unwired: 4 in, 3 out]
              n93 = Concatenate Strings("/hdd/GNSS/rinex/" ("string"), w299) -> (w304:string)
              n94 = Unbundle By Name(w297) -> ("BASEBAND"=w298:string)
              n95 = Concatenate Strings("SOURce1:BB:" ("string"), w298, ":RIN:ALM:GAL:FILE " ("string"), w306, w304, w306) -> (w307:string)
              n96 = call "MLLF_WriteToBuffer.vi"("String"=w307, "DriverConnect in"=w312) -> ("error out"=w310:T15, "DriverConnect out"=w311:T5)  [unwired: 6 in]
              n97 = call "RS_SMBV100A_Error_check.vi"("Driver Name"=w313, "Error Code"=w314, "Error In"=w310, "DriverConnect in"=w311) -> ("Error Out"=w309:errorcluster)  [unwired: 6 in, 1 out]
            }
            frame "GNSS_CONFIGURATION_RINEXFILE_GLONASS", "GNSSCONFIGURATION_RINEXFILE_GLONASS" {
              w325 = "'" ("string")
              # "Выбор файла GPS RINEX GLON"
              n98 = Search and Replace String(replace all?=TRUE, input string=w319, search string="\"", replace string="") -> (result string=w318:string)  [unwired: 4 in, 3 out]
              n99 = Concatenate Strings("/hdd/GNSS/rinex/" ("string"), w318) -> (w323:string)
              n100 = Unbundle By Name(w316) -> ("BASEBAND"=w317:string)
              n101 = Concatenate Strings("SOURce1:BB:" ("string"), w317, ":RIN:ALM:GLON:FILE " ("string"), w325, w323, w325) -> (w326:string)
              n102 = call "MLLF_WriteToBuffer.vi"("String"=w326, "DriverConnect in"=w331) -> ("error out"=w329:T15, "DriverConnect out"=w330:T5)  [unwired: 6 in]
              n103 = call "RS_SMBV100A_Error_check.vi"("Driver Name"=w332, "Error Code"=w333, "Error In"=w329, "DriverConnect in"=w330) -> ("Error Out"=w328:errorcluster)  [unwired: 6 in, 1 out]
            }
            frame "GNSS_CONFIGURATION_RINEX_FILE_GPS", "GNSSCONFIGURATION_RINEXFILE_GPS" {
              w344 = "'" ("string")
              # "Выбор файла GPS RINEX GLON"
              n104 = Search and Replace String(replace all?=TRUE, input string=w338, search string="\"", replace string="") -> (result string=w337:string)  [unwired: 4 in, 3 out]
              n105 = Concatenate Strings("/hdd/GNSS/rinex/" ("string"), w337) -> (w342:string)
              n106 = Unbundle By Name(w335) -> ("BASEBAND"=w336:string)
              n107 = Concatenate Strings("SOURce1:BB:" ("string"), w336, ":RIN:ALM:GPS:FILE " ("string"), w344, w342, w344) -> (w345:string)
              n108 = call "MLLF_WriteToBuffer.vi"("String"=w345, "DriverConnect in"=w350) -> ("error out"=w348:T15, "DriverConnect out"=w349:T5)  [unwired: 6 in]
              n109 = call "RS_SMBV100A_Error_check.vi"("Driver Name"=w351, "Error Code"=w352, "Error In"=w348, "DriverConnect in"=w349) -> ("Error Out"=w347:errorcluster)  [unwired: 6 in, 1 out]
            }
            frame "GNSS_CONFIGURATION_RINEX_FILE_GAL_STATE", "GNSSCONFIGURATION_RINEXFILE_GAL_STATE" {
              # "SOUR:BB:GLON:NAV:RIN:GAL:STAT OFF"
              # "Активировать\\Деактивировать GPS файла RINEX GLON"
              n110 = Unbundle By Name(w359) -> ("BASEBAND"=w361:string)
              n111 = call "MLLF_ParameterSelect.vi"("Command to equipment"=string[] ["ON\n", "OFF"], "Names"=string[][] [["ON", "1", "ENABLE", "EN"], ["OFF", "0", "DISABLE", "DIS"]], "Input"=w356, "Command"=w355, "Driver Name"=w354, "Error Code"=w353) -> ("Choice"=w358:string, "Error Out"=w366:errorcluster)  [unwired: 8 in]
              n112 = Concatenate Strings("SOUR:BB:", w361, ":NAV:RIN:GAL:STAT ", w358) -> (w357:string)
              n113 = call "MLLF_WriteToBuffer.vi"("String"=w357, "error in"=w366, "DriverConnect in"=w363) -> ("error out"=w364:T15, "DriverConnect out"=w365:T5)  [unwired: 5 in]
              n114 = call "RS_SMBV100A_Error_check.vi"("Driver Name"=w354, "Error Code"=w353, "Error In"=w364, "DriverConnect in"=w365) -> ("Error Out"=w369:errorcluster)  [unwired: 6 in, 1 out]
            }
            frame "GNSS_CONFIGURATION_RINEX_FILE_GLONASS_STATE", "GNSSCONFIGURATION_RINEXFILE_GLONASS_STATE" {
              # "SOUR:BB:GLON:NAV:RIN:GAL:STAT OFF"
              # "Активировать\\Деактивировать GPS файла RINEX GLON"
              n115 = Unbundle By Name(w376) -> ("BASEBAND"=w378:string)
              n116 = call "MLLF_ParameterSelect.vi"("Command to equipment"=string[] ["ON\n", "OFF"], "Names"=string[][] [["ON", "1", "ENABLE", "EN"], ["OFF", "0", "DISABLE", "DIS"]], "Input"=w373, "Command"=w372, "Driver Name"=w371, "Error Code"=w370) -> ("Choice"=w375:string, "Error Out"=w383:errorcluster)  [unwired: 8 in]
              n117 = Concatenate Strings("SOUR:BB:", w378, ":NAV:RIN:GLON:STAT ", w375) -> (w374:string)
              n118 = call "MLLF_WriteToBuffer.vi"("String"=w374, "error in"=w383, "DriverConnect in"=w380) -> ("error out"=w381:T15, "DriverConnect out"=w382:T5)  [unwired: 5 in]
              n119 = call "RS_SMBV100A_Error_check.vi"("Driver Name"=w371, "Error Code"=w370, "Error In"=w381, "DriverConnect in"=w382) -> ("Error Out"=w386:errorcluster)  [unwired: 6 in, 1 out]
            }
            frame "GNSS_CONFIGURATION_RINEX_FILE_GPS_STATE", "GNSSCONFIGURATION_RINEXFILE_GPS_STATE" {
              # "SOUR:BB:GLON:NAV:RIN:GAL:STAT OFF"
              # "Активировать\\Деактивировать GPS файла RINEX GLON"
              n120 = Unbundle By Name(w393) -> ("BASEBAND"=w395:string)
              n121 = call "MLLF_ParameterSelect.vi"("Command to equipment"=string[] ["ON\n", "OFF"], "Names"=string[][] [["ON", "1", "ENABLE", "EN"], ["OFF", "0", "DISABLE", "DIS"]], "Input"=w390, "Command"=w387, "Driver Name"=w389, "Error Code"=w388) -> ("Choice"=w392:string, "Error Out"=w400:errorcluster)  [unwired: 8 in]
              n122 = Concatenate Strings("SOUR:BB:", w395, ":NAV:RIN:GPS:STAT ", w392) -> (w391:string)
              n123 = call "MLLF_WriteToBuffer.vi"("String"=w391, "error in"=w400, "DriverConnect in"=w397) -> ("error out"=w398:T15, "DriverConnect out"=w399:T5)  [unwired: 5 in]
              n124 = call "RS_SMBV100A_Error_check.vi"("Driver Name"=w389, "Error Code"=w388, "Error In"=w398, "DriverConnect in"=w399) -> ("Error Out"=w403:errorcluster)  [unwired: 6 in, 1 out]
            }
            frame "GLONASS_LOAD_SCENARIO" {
              w425 = "'" ("string")
              # "Осуществляется подгрузка и в прибор и в драйвер сценария."
              # "загружаем сценарий для локации GLON"
              n125 = Search and Replace String(replace all?=TRUE, input string=w406, search string="\"", replace string="") -> (result string=w405:string)  [unwired: 4 in, 3 out]
              n126 = Concatenate Strings("GNSS\\scenario\\", w405, ".txt") -> (w415:string)
              n127 = Build Path(base path=w404, name or relative path=w415) -> (appended path=w410:path)
              n128 = Concatenate Strings("/hdd/GNSS/scenario/", w405, ".txt") -> (w411:string)
              n129 = Read from Text File(file (use dialog)=w410) -> (text=w429:string, error out=w420:errorcluster)  [unwired: 3 in, 2 out]
              n130 = Bundle By Name(cluster=w428, "GLONASS SCENARIO"=w429) -> (w427:T12)
              n131 = Concatenate Strings("SOUR:BB:GLON:LOC:WAYP:FILE " ("string"), w425, w411, w425) -> (w422:string)
              n132 = call "MLLF_WriteToBuffer.vi"("String"=w422, "error in"=w420, "DriverConnect in"=w421) -> ("error out"=w423:T15, "DriverConnect out"=w424:T5)  [unwired: 5 in]
              n133 = call "RS_SMBV100A_Error_check.vi"("Driver Name"=w417, "Error Code"=w418, "Error In"=w423, "DriverConnect in"=w424) -> ("Error Out"=w419:errorcluster)  [unwired: 6 in, 1 out]
            }
            frame "GLONASS_LOAD_WAYPOINTS" {
              # "Импортируем WAyPOINTS в драйвер"
              n134 = Search and Replace String(replace all?=TRUE, input string=w431, search string="\"", replace string="") -> (result string=w432:string)  [unwired: 4 in, 3 out]
              n135 = Concatenate Strings("GNSS\\waypoints\\", w432, ".txt") -> (w444:string)
              n136 = Build Path(base path=w430, name or relative path=w444) -> (appended path=w442:path)
              n137 = Read from Text File(file (use dialog)=w442) -> (text=w439:string, error out=w438:errorcluster)  [unwired: 3 in, 2 out]
              n138 = call "RS_SMBV100A_arrayStringToDOUBLE.vi"("string"=w439, "error in"=w438) -> ("Dynam waypoints"=w436:T10, "error out"=w437:errorcluster)  [unwired: 1 in]
              n139 = Bundle By Name(cluster=w441, "GLONASS WAYPOINTS"=w436) -> (w440:T12)
            }
            frame "------------------------------------ LOCALIZATION_DATA -----------------------------------" {
            }
            frame "LOCALIZATION_DATA_GEOGRAPHYCLOCATION", "LOCALIZATIONDATA_GEOGRAPHYCLOCATION" {
              # "выбираем позицию GLON приемника"
              n140 = Unbundle By Name(w454) -> ("BASEBAND"=w453:string)
              n141 = call "MLLF_ParameterSelect.vi"("Command to equipment"=string[] ["\"Waypoints\"", "\"User Defined\"", "\"New York\"", "\"BEIJING\"", "\"SEOUL\"", "\"SINGAPORE\"", "\"TAIPEI\"", "\"TOKYO\"", "\"SYDNEY\"", "\"LONDON\"", "\"MOSCOW\"", "\"MUNICH\"", "\"PARIS\""], "Names"=string[][] [["WAIPOINTS", "", ""], ["USER_DEFINE", "USER", "USER DEFINE"], ["NEW YORK", "NEW_YORK", ""], ["BEIJING", "", ""], ["SEOUL", "", ""], ["SINGAPORE", "", ""], ["TAIPEI", "", ""], ["TOKYO", "", ""], ["SYDNEY", "", ""], ["LONDON", "", ""], ["MOSCOW", "", ""], ["MUNICH", "", ""], ["PARIS", "", ""]], "Input"=w448, "Command"=w447, "Driver Name"=w459, "Error Code"=w460) -> ("Choice"=w450:string, "Error Out"=w461:errorcluster)  [unwired: 8 in]
              n142 = Concatenate Strings("SOUR:BB:", w453, ":LOC:SEL ", w450) -> (w449:string)
              n143 = call "MLLF_WriteToBuffer.vi"("String"=w449, "error in"=w461, "DriverConnect in"=w458) -> ("error out"=w456:T15, "DriverConnect out"=w457:T5)  [unwired: 5 in]
              n144 = call "RS_SMBV100A_Error_check.vi"("Driver Name"=w459, "Error Code"=w460, "Error In"=w456, "DriverConnect in"=w457) -> ("Error Out"=w455:errorcluster)  [unwired: 6 in, 1 out]
            }
            frame "LOCALIZATION_DATA_POSITION", "LOCALIZATIONDATA_POSITION" {
              w476 = ", " ("string")
              w478 = " %.;%1.7f" ("format")
              # "вот так правильно!"
              # "Позиция GLON приемника при USER DEFINE <Latitude> ,<Longitude>,<Altitude>"
              n145 = call "MLLF_FormatStringValue.vi"("String Value"=w466, "Format"=w478) -> ("error out"=w475:T15, "String Value Formated"=w470:T16)  [unwired: 7 in, 1 out]
              n146 = Unbundle By Name(w469) -> ("BASEBAND"=w467:string)
              n147 = call "MLLF_FormatStringValue.vi"("error in"=w475, "String Value"=w465, "Format"=w478) -> ("error out"=w474:T15, "String Value Formated"=w471:T16)  [unwired: 6 in, 1 out]
              n148 = call "MLLF_FormatStringValue.vi"("error in"=w474, "String Value"=w464, "Format"=w478) -> ("error out"=w473:T15, "String Value Formated"=w477:T16)  [unwired: 6 in, 1 out]
              n149 = Concatenate Strings("SOUR:BB:", w467, ":LOC:COOR:DEC " ("string"), w471, w476, w470, w476, w477) -> (w472:string)
              n150 = call "MLLF_WriteToBuffer.vi"("String"=w472, "error in"=w473, "DriverConnect in"=w483) -> ("error out"=w481:T15, "DriverConnect out"=w482:T5)  [unwired: 5 in]
              n151 = call "RS_SMBV100A_Error_check.vi"("Driver Name"=w484, "Error Code"=w485, "Error In"=w481, "DriverConnect in"=w482) -> ("Error Out"=w480:errorcluster)  [unwired: 6 in, 1 out]
            }
            frame "LOCALIZATION_DATA_READ_OUTMODE", "LOCALIZATIONDATA_READOUTMODE" {
              # "Использование сценария GLON"
              n152 = Unbundle By Name(w488) -> ("BASEBAND"=w489:string)
              n153 = call "MLLF_ParameterSelect.vi"("Command to equipment"=string[] ["CYCL", "OWAY", "RTR"], "Names"=string[][] [["CYCLE", "CYCLIC", ""], ["ONE WAY", "ONE", "OWAY"], ["ROUND TRIP", "ROUND", "RTR"]], "Input"=w487, "Command"=w486, "Driver Name"=w498, "Error Code"=w499) -> ("Choice"=w491:string, "Error Out"=w500:errorcluster)  [unwired: 8 in]
              n154 = Concatenate Strings("SOUR:BB:", w489, ":LOC:WAYP:ROM ", w491) -> (w490:string)
              n155 = call "MLLF_WriteToBuffer.vi"("String"=w490, "error in"=w500, "DriverConnect in"=w497) -> ("error out"=w495:T15, "DriverConnect out"=w496:T5)  [unwired: 5 in]
              n156 = call "RS_SMBV100A_Error_check.vi"("Driver Name"=w498, "Error Code"=w499, "Error In"=w495, "DriverConnect in"=w496) -> ("Error Out"=w494:errorcluster)  [unwired: 6 in, 1 out]
            }
            frame "LOCALIZATION_DATA_REFERENCE_FRAME", "LOCALIZATIONDATA_REFERENCEFRAME" {
              # "Использование сценария GLON"
              n157 = Unbundle By Name(w505) -> ("BASEBAND"=w508:string)
              n158 = call "MLLF_ParameterSelect.vi"("Command to equipment"=string[] ["WGS84", "PZ90"], "Names"=string[][] [["WGS84", "WGS_84", "WGS-84"], ["PZ90", "PZ_90", "PZ-90"]], "Input"=w504, "Command"=w503, "Driver Name"=w515, "Error Code"=w516) -> ("Choice"=w507:string, "Error Out"=w517:errorcluster)  [unwired: 8 in]
              n159 = Concatenate Strings("SOUR:BB:", w508, ":LOC:COOR:RFR ", w507) -> (w506:string)
              n160 = call "MLLF_WriteToBuffer.vi"("String"=w506, "error in"=w517, "DriverConnect in"=w514) -> ("error out"=w512:T15, "DriverConnect out"=w513:T5)  [unwired: 5 in]
              n161 = call "RS_SMBV100A_Error_check.vi"("Driver Name"=w515, "Error Code"=w516, "Error In"=w512, "DriverConnect in"=w513) -> ("Error Out"=w511:errorcluster)  [unwired: 6 in, 1 out]
            }
            frame "LOCALIZATION_DATA_SMOOTH_MOVEMENT", "LOCALIZATIONDATA_SMOOTHMOVEMENT" {
              # "Активировать функцию Smooth Movement"
              n162 = Unbundle By Name(w524) -> ("BASEBAND"=w527:string)
              n163 = call "MLLF_ParameterSelect.vi"("Command to equipment"=string[] ["ON\n", "OFF"], "Names"=string[][] [["ON", "1", "ENABLE", "EN"], ["OFF", "0", "DISABLE", "DIS"]], "Input"=w523, "Command"=w522, "Driver Name"=w521, "Error Code"=w520) -> ("Choice"=w526:string, "Error Out"=w533:errorcluster)  [unwired: 8 in]
              n164 = Concatenate Strings("SOUR:BB:", w527, ":LOC:SMOV ", w526) -> (w525:string)
              n165 = call "MLLF_WriteToBuffer.vi"("String"=w525, "error in"=w533, "DriverConnect in"=w530) -> ("error out"=w531:T15, "DriverConnect out"=w532:T5)  [unwired: 5 in]
              n166 = call "RS_SMBV100A_Error_check.vi"("Driver Name"=w521, "Error Code"=w520, "Error In"=w531, "DriverConnect in"=w532) -> ("Error Out"=w536:errorcluster)  [unwired: 6 in, 1 out]
            }
            frame "LOCALIZATION_DATA_WAIPOINTS", "LOCALIZATIONDATA_WAIPOINTS" {
              w548 = "'" ("string")
              # "Выбор файла сценария GPS приемника"
              n167 = Search and Replace String(replace all?=TRUE, input string=w541, search string="\"", replace string="") -> (result string=w540:string)  [unwired: 4 in, 3 out]
              n168 = Unbundle By Name(w539) -> ("BASEBAND"=w538:string)
              n169 = Concatenate Strings("/hdd/GNSS/scenario/" ("string"), w540, ".txt" ("string")) -> (w545:string)
              n170 = Concatenate Strings("SOUR:BB:", w538, ":LOC:WAYP:FILE " ("string"), w548, w545, w548) -> (w549:string)
              n171 = call "MLLF_WriteToBuffer.vi"("String"=w549, "DriverConnect in"=w554) -> ("error out"=w552:T15, "DriverConnect out"=w553:T5)  [unwired: 6 in]
              n172 = call "RS_SMBV100A_Error_check.vi"("Driver Name"=w555, "Error Code"=w556, "Error In"=w552, "DriverConnect in"=w553) -> ("Error Out"=w551:errorcluster)  [unwired: 6 in, 1 out]
            }
            frame "RFBAND" {
              # "Настройка частоты GLONASS грожданская/военная"
              n173 = Unbundle By Name(w560) -> ("BASEBAND"=w561:string)
              n174 = call "MLLF_ParameterSelect.vi"("Command to equipment"=string[] ["L1", "L2"], "Names"=string[][] [["L1", "L1/E2"], ["L2", ""]], "Input"=w557, "Driver Name"=w568, "Error Code"=w569) -> ("Choice"=w558:string, "Error Out"=w570:errorcluster)  [unwired: 9 in]
              n175 = Concatenate Strings("BB:", w561, ":RFB ", w558) -> (w559:string)
              n176 = call "MLLF_WriteToBuffer.vi"("String"=w559, "error in"=w570, "DriverConnect in"=w567) -> ("error out"=w565:T15, "DriverConnect out"=w566:T5)  [unwired: 5 in]
              n177 = call "RS_SMBV100A_Error_check.vi"("Driver Name"=w568, "Error Code"=w569, "Error In"=w565, "DriverConnect in"=w566) -> ("Error Out"=w564:errorcluster)  [unwired: 6 in, 1 out]
            }
            frame "TimeProjectionOfNavigationData" {
              # "<subsystem>:SVID<ch>:<GNSS>:NMESsage:\nRTPRojection."
              n178 = Unbundle By Name(w577) -> ("BASEBAND"=w580:string)
              n179 = call "MLLF_ParameterSelect.vi"("Command to equipment"=string[] ["ON\n", "OFF"], "Names"=string[][] [["ON", "1", "ENABLE", "EN"], ["OFF", "0", "DISABLE", "DIS"]], "Input"=w576, "Command"=w575, "Driver Name"=w574, "Error Code"=w573) -> ("Choice"=w578:string, "Error Out"=w587:errorcluster)  [unwired: 8 in]
              n180 = Concatenate Strings("SOURce1:BB:", w580, ":SATellite:GRTProjection ", w578) -> (w579:string)
              n181 = call "MLLF_WriteToBuffer.vi"("String"=w579, "error in"=w587, "DriverConnect in"=w584) -> ("error out"=w585:T15, "DriverConnect out"=w586:T5)  [unwired: 5 in]
              n182 = call "RS_SMBV100A_Error_check.vi"("Driver Name"=w574, "Error Code"=w573, "Error In"=w585, "DriverConnect in"=w586) -> ("Error Out"=w583:errorcluster)  [unwired: 6 in, 1 out]
            }
            frame "------------------------ SATELLITE_CONFIGURATIONS ---------------------------" {
            }
            frame "SATELLITE_CONFIGURATIONS_ELEVATION_MASK", "SATELLITECONFIGURATIONS_ELEVATIONMASK" {
              # "Угол отсечки по GLON"
              n183 = Unbundle By Name(w594) -> ("BASEBAND"=w595:string)
              n184 = call "MLLF_ParameterSelect.vi"("Command to equipment"=string[] ["0", "2.5", "5", "7.5", "10"], "Names"=string[][] [["0", ""], ["2.5", "2,5"], ["5", ""], ["7.5", "7,5"], ["10", ""]], "Input"=w591, "Driver Name"=w600, "Error Code"=w599) -> ("Choice"=w593:string, "Error Out"=w598:errorcluster)  [unwired: 9 in]
              n185 = Concatenate Strings("SOUR:BB:", w595, ":SEM ", w593) -> (w592:string)
              n186 = call "MLLF_WriteToBuffer.vi"("String"=w592, "error in"=w598, "DriverConnect in"=w606) -> ("error out"=w604:T15, "DriverConnect out"=w605:T5)  [unwired: 5 in]
              n187 = call "RS_SMBV100A_Error_check.vi"("Driver Name"=w600, "Error Code"=w599, "Error In"=w604, "DriverConnect in"=w605) -> ("Error Out"=w603:errorcluster)  [unwired: 6 in, 1 out]
            }
            frame "SATELLITECONFIGURATIONS_GETOPTIMALCONSTELATION" {
              # "Установить оптимальную конфигурацию спутников"
              n188 = Unbundle By Name(w607) -> ("BASEBAND"=w609:string)
              n189 = Concatenate Strings("SOUR:BB:", w609, ":GOC ") -> (w608:string)
              n190 = call "MLLF_WriteToBuffer.vi"("String"=w608, "DriverConnect in"=w615) -> ("error out"=w613:T15, "DriverConnect out"=w614:T5)  [unwired: 6 in]
              n191 = call "RS_SMBV100A_Error_check.vi"("Driver Name"=w616, "Error Code"=w617, "Error In"=w613, "DriverConnect in"=w614) -> ("Error Out"=w612:errorcluster)  [unwired: 6 in, 1 out]
            }
            frame "SATELLITECONFIGURATIONS_MAXIMUMNUMBEROFSATELLITES" {
              # "Колличество спутников В модуле GLON"
              n192 = Unbundle By Name(w620) -> ("BASEBAND"=w623:string)
              n193 = call "MLLF_ParameterSelect.vi"("Command to equipment"=string[] ["1", "4", "5", "6", "7", "8", "9", "10", "11", "12", "13", "14", "15", "16", "17", "18", "19", "20", "21", "22", "23", "24"], "Names"=string[][] [["1"], ["4"], ["5"], ["6"], ["7"], ["8"], ["9"], ["10"], ["11"], ["12"], ["13"], ["14"], ["15"], ["16"], ["17"], ["18"], ["19"], ["20"], ["21"], ["22"], ["23"], ["24"]], "Input"=w619, "Command"=w618, "Driver Name"=w630, "Error Code"=w631) -> ("Choice"=w621:string, "Error Out"=w632:errorcluster)  [unwired: 8 in]
              n194 = Concatenate Strings("SOUR:BB:", w623, ":SAT:COUNT ", w621) -> (w622:string)
              n195 = call "MLLF_WriteToBuffer.vi"("String"=w622, "error in"=w632, "DriverConnect in"=w629) -> ("error out"=w627:T15, "DriverConnect out"=w628:T5)  [unwired: 5 in]
              n196 = call "RS_SMBV100A_Error_check.vi"("Driver Name"=w630, "Error Code"=w631, "Error In"=w627, "DriverConnect in"=w628) -> ("Error Out"=w626:errorcluster)  [unwired: 6 in, 1 out]
            }
            frame "SATELLITECONFIGURATIONS_PseudorangeBias" {
              # "Функции настройки ephemeris в локации GPS - TOE"
              n197 = Unbundle By Name(w639) -> ("BASEBAND"=w637:string)
              n198 = call "RS_SMBV100A_N_in_SKY_to_SAT_in_DEVICE.vi"("DriverConnect in"=w649, "BASEBAND"=w637, "String Value"=w636) -> ("DriverConnect out"=w645:T5, "SAT"=w640:dbl, "Error Out"=w644:errorcluster)  [unwired: 8 in, 2 out]
              n199 = Format Into String(format string="%.;%1.0f" ("format"), error in=w644, w640) -> (resulting string=w641:string, error out=w643:errorcluster)  [unwired: 1 in]
              n200 = Concatenate Strings("SOUR:BB:", w637, ":SATellite" ("regular expression"), w641, ":PRBias " ("regular expression"), w635) -> (w646:string)
              n201 = call "MLLF_WriteToBuffer.vi"("String"=w646, "error in"=w643, "DriverConnect in"=w645) -> ("error out"=w651:T15, "DriverConnect out"=w652:T5)  [unwired: 5 in]
              n202 = call "RS_SMBV100A_Error_check.vi"("Driver Name"=w653, "Error Code"=w654, "Error In"=w651, "DriverConnect in"=w652) -> ("Error Out"=w650:errorcluster)  [unwired: 6 in, 1 out]
            }
            frame "SATELLITECONFIGURATIONS_POWERMODE" {
              # "Модуль мощности GLON"
              n203 = Unbundle By Name(w657) -> ("BASEBAND"=w660:string)
              n204 = call "MLLF_ParameterSelect.vi"("Command to equipment"=string[] ["USER", "AUTO"], "Names"=string[][] [["USER"], ["AUTO"]], "Input"=w656, "Command"=w655, "Driver Name"=w669, "Error Code"=w670) -> ("Choice"=w659:string, "Error Out"=w671:errorcluster)  [unwired: 8 in]
              n205 = Concatenate Strings("SOUR:BB:", w660, ":POW:MODE ", w659) -> (w658:string)
              n206 = call "MLLF_WriteToBuffer.vi"("String"=w658, "error in"=w671, "DriverConnect in"=w668) -> ("error out"=w666:T15, "DriverConnect out"=w667:T5)  [unwired: 5 in]
              n207 = call "RS_SMBV100A_Error_check.vi"("Driver Name"=w669, "Error Code"=w670, "Error In"=w666, "DriverConnect in"=w667) -> ("Error Out"=w665:errorcluster)  [unwired: 6 in, 1 out]
            }
            frame "SATELLITECONFIGURATIONS_REFPOWER" {
              # "от -145 до 20 dBm"
              # "Опорная Мощность по GLON"
              n208 = call "MLLF_FormatStringValue.vi"("String Value"=w672, "Format"=" %.;%1.2f" ("format")) -> ("error out"=w677:T15, "String Value Formated"=w678:T16)  [unwired: 7 in, 1 out]
              n209 = Unbundle By Name(w673) -> ("BASEBAND"=w674:string)
              n210 = Concatenate Strings("SOUR:BB:", w674, ":POW:REF:POW " ("string"), w678) -> (w676:string)
              n211 = call "MLLF_WriteToBuffer.vi"("String"=w676, "error in"=w677, "DriverConnect in"=w684) -> ("error out"=w682:T15, "DriverConnect out"=w683:T5)  [unwired: 5 in]
              n212 = call "RS_SMBV100A_Error_check.vi"("Driver Name"=w685, "Error Code"=w686, "Error In"=w682, "DriverConnect in"=w683) -> ("Error Out"=w681:errorcluster)  [unwired: 6 in, 1 out]
            }
            frame "SATELLITECONFIGURATIONS_REFSATELLITE" {
              # "!!!!!!!!!!!!!!!! N.A. -  устанавливается по умолчанию при сбросе\nНО не выставляется из CASE!!! так как указано в документации\n!!!!!!!!!!!!!!!!!!!!!!!!!!!!!!!!!!!!!!!!!!!!!!!!!!!!!!!!!!!!!!!!!!!!!!!!!!!!!!!!!\nПроизводители вкурсе ИХ КАСЯК!!!"
              # "Опорный спутник по мощности GLON"
              n213 = Unbundle By Name(w690) -> ("BASEBAND"=w691:string)
              n214 = call "MLLF_ParameterSelect.vi"("Command to equipment"=string[] ["-1", "1", "2", "3", "4", "5", "6", "7", "8", "9", "10", "11", "12", "13", "14", "15", "16", "17", "18", "19", "20", "21", "22", "23", "24"], "Names"=string[][] [["N.A.", "NA"], ["1", ""], ["2", ""], ["3", ""], ["4", ""], ["5", ""], ["6", ""], ["7", ""], ["8", ""], ["9", ""], ["10", ""], ["11", ""], ["12", ""], ["13", ""], ["14", ""], ["15", ""], ["16", ""], ["17", ""], ["18", ""], ["19", ""], ["20", ""], ["21", ""], ["22", ""], ["23", ""], ["24", ""]], "Input"=w687, "Driver Name"=w700, "Error Code"=w701) -> ("Choice"=w688:string, "Error Out"=w702:errorcluster)  [unwired: 9 in]
              n215 = Concatenate Strings("SOUR:BB:", w691, ":POW:REF:SAT ", w688) -> (w689:string)
              n216 = call "MLLF_WriteToBuffer.vi"("String"=w689, "error in"=w702, "DriverConnect in"=w699) -> ("error out"=w697:T15, "DriverConnect out"=w698:T5)  [unwired: 5 in]
              n217 = call "RS_SMBV100A_Error_check.vi"("Driver Name"=w700, "Error Code"=w701, "Error In"=w697, "DriverConnect in"=w698) -> ("Error Out"=w696:errorcluster)  [unwired: 6 in, 1 out]
            }
            frame "SATELLITECONFIGURATIONS_REFSTANDART" {
              # "SOUR:BB:GLON:POW:REF:STAN GAL"
              # "Опорный стандарт по мощности GLON"
              n218 = Unbundle By Name(w704) -> ("BASEBAND"=w707:string)
              n219 = call "MLLF_ParameterSelect.vi"("Command to equipment"=string[] ["GPS", "GLON", "GAL"], "Names"=string[][] [["GPS"], ["GLONASS"], ["GALILEO"]], "Input"=w703, "Driver Name"=w716, "Error Code"=w717) -> ("Choice"=w705:string, "Error Out"=w718:errorcluster)  [unwired: 9 in]
              n220 = Concatenate Strings("SOUR:BB:", w707, ":POW:REF:STAN ", w705) -> (w706:string)
              n221 = call "MLLF_WriteToBuffer.vi"("String"=w706, "error in"=w718, "DriverConnect in"=w715) -> ("error out"=w713:T15, "DriverConnect out"=w714:T5)  [unwired: 5 in]
              n222 = call "RS_SMBV100A_Error_check.vi"("Driver Name"=w716, "Error Code"=w717, "Error In"=w713, "DriverConnect in"=w714) -> ("Error Out"=w712:errorcluster)  [unwired: 6 in, 1 out]
            }
            frame "SIMULATIONMODE", "SMODE" {
              # "SOUR:BB:GLON:SMOD  USER"
              # "Выбор симуляции GLONASS статический\\автоматический\\пользовательский"
              n223 = Unbundle By Name(w722) -> ("BASEBAND"=w723:string)
              n224 = call "MLLF_ParameterSelect.vi"("Command to equipment"=string[] ["STAT", "AUTO", "USER"], "Names"=string[][] [["STATIC"], ["AUTO"], ["USER"]], "Input"=w719, "Driver Name"=w730, "Error Code"=w731) -> ("Choice"=w720:string, "Error Out"=w732:errorcluster)  [unwired: 9 in]
              n225 = Concatenate Strings("SOUR:BB:", w723, ":SMOD ", w720) -> (w721:string)
              n226 = call "MLLF_WriteToBuffer.vi"("String"=w721, "error in"=w732, "DriverConnect in"=w729) -> ("error out"=w727:T15, "DriverConnect out"=w728:T5)  [unwired: 5 in]
              n227 = call "RS_SMBV100A_Error_check.vi"("Driver Name"=w730, "Error Code"=w731, "Error In"=w727, "DriverConnect in"=w728) -> ("Error Out"=w726:errorcluster)  [unwired: 6 in, 1 out]
            }
            frame "----------------------------  SIMULATION_START_TIME ----------------------------------------" {
            }
            frame "SIMULATION_START_TIME", "SIMULATIONSTARTTIME" {
              # "SOUR:BB:GLON:NAV:SIM:TBAS UTC"
              # "Формат времени GLON"
              n228 = Unbundle By Name(w740) -> ("BASEBAND"=w743:string)
              n229 = call "MLLF_ParameterSelect.vi"("Command to equipment"=string[] ["UTC", "GLO", "GPS"], "Names"=string[][] [["UTC", ""], ["GLO", "GLONASS"], ["GPS", ""]], "Input"=w739, "Command"=w738, "Driver Name"=w737, "Error Code"=w736) -> ("Choice"=w741:string, "Error Out"=w749:errorcluster)  [unwired: 8 in]
              n230 = Concatenate Strings("SOUR:BB:", w743, ":NAV:SIM:TBAS ", w741) -> (w742:string)
              n231 = call "MLLF_WriteToBuffer.vi"("String"=w742, "error in"=w749, "DriverConnect in"=w748) -> ("error out"=w746:T15, "DriverConnect out"=w747:T5)  [unwired: 5 in]
              n232 = call "RS_SMBV100A_Error_check.vi"("Driver Name"=w737, "Error Code"=w736, "Error In"=w746, "DriverConnect in"=w747) -> ("Error Out"=w752:errorcluster)  [unwired: 6 in, 1 out]
            }
            frame "SIMULATIONSTARTTIME_DATE" {
              # "SOUR:BB:GLON:NAV:SIM:DATE %,;%<%Y,%m,%d>T"
              # "Вносим дату времени GLON"
              n233 = Search and Replace String(replace all?=TRUE, input string=w759, search string=".", replace string=",") -> (result string=w761:string, error out=w760:errorcluster)  [unwired: 4 in, 2 out]
              n234 = Unbundle By Name(w755) -> ("BASEBAND"=w756:string)
              n235 = Scan From String(format string="%.;%<%d,%m,%Y>T", input string=w761, error in=w760) -> (error out=w765:errorcluster, output 1=w768:timestamp)  [unwired: 2 in, 2 out]
              n236 = Format Into String(format string="%,;%<%Y,%m,%d>T", error in=w765, w768) -> (resulting string=w754:string, error out=w766:errorcluster)  [unwired: 1 in]
              n237 = Concatenate Strings("SOUR:BB:", w756, ":NAV:SIM:DATE ", w754) -> (w753:string)
              n238 = call "MLLF_WriteToBuffer.vi"("String"=w753, "error in"=w766, "DriverConnect in"=w772) -> ("error out"=w770:T15, "DriverConnect out"=w771:T5)  [unwired: 5 in]
              n239 = call "RS_SMBV100A_Error_check.vi"("Driver Name"=w774, "Error Code"=w775, "Error In"=w770, "DriverConnect in"=w771) -> ("Error Out"=w773:errorcluster)  [unwired: 6 in, 1 out]
            }
            frame "SIMULATIONSTARTTIME_TIME" {
              w791 = " %.;%1.3f" ("format")
              # "SOUR:BB:GLON:NAV:SIM:TIME %.;%<%H,%M,%S%5u>T"
              # "string               sec     sec"
              # "GLONASS_SIMULATIONSTARTTIME_TIME= 05,00,00.000 3456 -34551"
              # "Вносим время времени GLON"
              n240 = Unbundle By Name(w778) -> ("BASEBAND"=w779:string)
              n241 = Match Pattern(string=w783, regular expression="[\\s\\t]+") -> (before substring=w787:string, after substring=w792:string)  [unwired: 1 in, 2 out]
              n242 = Match Pattern(string=w792, regular expression="[\\s\\t]+") -> (before substring=w789:string, after substring=w788:string)  [unwired: 1 in, 2 out]
              n243 = call "MLLF_FormatStringValue.vi"("String Value"=w789, "Format"=w791) -> ("error out"=w790:T15, "number"=w785:dbl)  [unwired: 7 in, 1 out]
              n244 = call "MLLF_FormatStringValue.vi"("error in"=w790, "String Value"=w788, "Format"=w791) -> ("error out"=w786:T15, "number"=w784:dbl)  [unwired: 6 in, 1 out]
              n245 = Scan From String(format string="%.;%<%H,%M,%S%5u>T", input string=w787, error in=w786) -> (error out=w797:errorcluster, output 1=w798:timestamp)  [unwired: 2 in, 2 out]
              n246 = Add(x=w798, y=w785) -> (x+y=w795:timestamp)
              n247 = Add(x=w795, y=w784) -> (x+y=w796:timestamp)
              n248 = Format Into String(format string="%.;%<%H,%M,%S%5u>T", error in=w797, w796) -> (resulting string=w777:string, error out=w782:errorcluster)  [unwired: 1 in]
              n249 = Concatenate Strings("SOUR:BB:", w779, ":NAV:SIM:TIME ", w777) -> (w776:string)
              n250 = call "MLLF_WriteToBuffer.vi"("String"=w776, "error in"=w782, "DriverConnect in"=w803) -> ("error out"=w801:T15, "DriverConnect out"=w802:T5)  [unwired: 5 in]
              n251 = call "RS_SMBV100A_Error_check.vi"("Driver Name"=w805, "Error Code"=w806, "Error In"=w801, "DriverConnect in"=w802) -> ("Error Out"=w804:errorcluster)  [unwired: 6 in, 1 out]
            }
            frame "STATE" {
              # "Включение/выключения модуляции"
              n252 = Unbundle By Name(w809) -> ("BASEBAND"=w812:string)
              n253 = call "MLLF_ParameterSelect.vi"("Command to equipment"=string[] ["ON", "OFF"], "Names"=string[][] [["ON", "1", "ENABLE", "EN"], ["OFF", "0", "DISABLE", "DIS"]], "Input"=w808, "Command"=w807, "Driver Name"=w819, "Error Code"=w820) -> ("Choice"=w811:string, "Error Out"=w821:errorcluster)  [unwired: 8 in]
              n254 = Concatenate Strings("SOUR:BB:", w812, ":STAT ", w811) -> (w810:string)
              n255 = call "MLLF_WriteToBuffer.vi"("String"=w810, "error in"=w821, "DriverConnect in"=w818) -> ("error out"=w816:T15, "DriverConnect out"=w817:T5)  [unwired: 5 in]
              n256 = call "RS_SMBV100A_Error_check.vi"("Driver Name"=w819, "Error Code"=w820, "Error In"=w816, "DriverConnect in"=w817) -> ("Error Out"=w815:errorcluster)  [unwired: 6 in, 1 out]
            }
            frame "-------------------- SYSTEM_CONFIGURATION -----------------------------------" {
            }
            frame "SYSTEM_CONFIGURATION_ANTI_SPOOFING", "SYSTEMCONFIGURATION_ANTI_SPOOFING" {
              # "GLON ANTI-SPOOFING"
              n257 = Unbundle By Name(w827) -> ("BASEBAND"=w830:string)
              n258 = call "MLLF_ParameterSelect.vi"("Command to equipment"=string[] ["ON", "OFF"], "Names"=string[][] [["ON", "1", "ENABLE", "EN"], ["OFF", "0", "DISABLE", "DIS"]], "Input"=w826, "Command"=w825, "Driver Name"=w837, "Error Code"=w838) -> ("Choice"=w829:string, "Error Out"=w839:errorcluster)  [unwired: 8 in]
              n259 = Concatenate Strings("SOUR:BB:", w830, ":SAT:ASP ", w829) -> (w828:string)
              n260 = call "MLLF_WriteToBuffer.vi"("String"=w828, "error in"=w839, "DriverConnect in"=w836) -> ("error out"=w834:T15, "DriverConnect out"=w835:T5)  [unwired: 5 in]
              n261 = call "RS_SMBV100A_Error_check.vi"("Driver Name"=w837, "Error Code"=w838, "Error In"=w834, "DriverConnect in"=w835) -> ("Error Out"=w833:errorcluster)  [unwired: 6 in, 1 out]
            }
            frame "SYSTEM_CONFIGURATION_GLONASS", "SYSTEMCONFIGURATION_GLONASS" {
              # "Подмешиваем спутники GLONASS"
              n262 = Unbundle By Name(w844) -> ("BASEBAND"=w847:string)
              n263 = call "MLLF_ParameterSelect.vi"("Command to equipment"=string[] ["ON", "OFF"], "Names"=string[][] [["ON", "1", "ENABLE", "EN"], ["OFF", "0", "DISABLE", "DIS"]], "Input"=w843, "Command"=w842, "Driver Name"=w854, "Error Code"=w855) -> ("Choice"=w846:string, "Error Out"=w856:errorcluster)  [unwired: 8 in]
              n264 = Concatenate Strings("SOUR:BB:", w847, ":HYBR:GLON:STAT  ", w846) -> (w845:string)
              n265 = call "MLLF_WriteToBuffer.vi"("String"=w845, "error in"=w856, "DriverConnect in"=w853) -> ("error out"=w851:T15, "DriverConnect out"=w852:T5)  [unwired: 5 in]
              n266 = call "RS_SMBV100A_Error_check.vi"("Driver Name"=w854, "Error Code"=w855, "Error In"=w851, "DriverConnect in"=w852) -> ("Error Out"=w850:errorcluster)  [unwired: 6 in, 1 out]
            }
            frame "SYSTEM_CONFIGURATION_GALILEO", "SYSTEMCONFIGURATION_GALILEO" {
              # "Подмешиваем спутники GPS"
              n267 = Unbundle By Name(w862) -> ("BASEBAND"=w865:string)
              n268 = call "MLLF_ParameterSelect.vi"("Command to equipment"=string[] ["ON", "OFF"], "Names"=string[][] [["ON", "1", "ENABLE", "EN"], ["OFF", "0", "DISABLE", "DIS"]], "Input"=w861, "Command"=w859, "Driver Name"=w860, "Error Code"=w872) -> ("Choice"=w863:string, "Error Out"=w873:errorcluster)  [unwired: 8 in]
              n269 = Concatenate Strings("SOUR:BB:", w865, ":HYBR:GAL:STAT  ", w863) -> (w864:string)
              n270 = call "MLLF_WriteToBuffer.vi"("String"=w864, "error in"=w873, "DriverConnect in"=w871) -> ("error out"=w869:T15, "DriverConnect out"=w870:T5)  [unwired: 5 in]
              n271 = call "RS_SMBV100A_Error_check.vi"("Driver Name"=w860, "Error Code"=w872, "Error In"=w869, "DriverConnect in"=w870) -> ("Error Out"=w868:errorcluster)  [unwired: 6 in, 1 out]
            }
            frame "SYSTEM_CONFIGURATION_GPS", "SYSTEMCONFIGURATION_GPS" {
              # "Подмешиваем спутники GPS"
              n272 = Unbundle By Name(w878) -> ("BASEBAND"=w881:string)
              n273 = call "MLLF_ParameterSelect.vi"("Command to equipment"=string[] ["ON", "OFF"], "Names"=string[][] [["ON", "1", "ENABLE", "EN"], ["OFF", "0", "DISABLE", "DIS"]], "Input"=w877, "Command"=w876, "Driver Name"=w888, "Error Code"=w889) -> ("Choice"=w880:string, "Error Out"=w890:errorcluster)  [unwired: 8 in]
              n274 = Concatenate Strings("SOUR:BB:", w881, ":HYBR:GPS:STAT  ", w880) -> (w879:string)
              n275 = call "MLLF_WriteToBuffer.vi"("String"=w879, "error in"=w890, "DriverConnect in"=w887) -> ("error out"=w885:T15, "DriverConnect out"=w886:T5)  [unwired: 5 in]
              n276 = call "RS_SMBV100A_Error_check.vi"("Driver Name"=w888, "Error Code"=w889, "Error In"=w885, "DriverConnect in"=w886) -> ("Error Out"=w884:errorcluster)  [unwired: 6 in, 1 out]
            }
            frame "SYSTEM_CONFIGURATION_USE_COMMON_RF_FREQUENCY", "SYSTEMCONFIGURATION_USECOMMONRFFREQUENCY" {
              # "Используем опорную частоту GLON"
              n277 = Unbundle By Name(w894) -> ("BASEBAND"=w897:string)
              n278 = call "MLLF_ParameterSelect.vi"("Command to equipment"=string[] ["ON", "OFF"], "Names"=string[][] [["ON", "1", "ENABLE", "EN"], ["OFF", "0", "DISABLE", "DIS"]], "Input"=w893, "Driver Name"=w904, "Error Code"=w905) -> ("Choice"=w895:string, "Error Out"=w906:errorcluster)  [unwired: 9 in]
              n279 = Concatenate Strings("SOUR:BB:", w897, ":UCRF ", w895) -> (w896:string)
              n280 = call "MLLF_WriteToBuffer.vi"("String"=w896, "error in"=w906, "DriverConnect in"=w903) -> ("error out"=w901:T15, "DriverConnect out"=w902:T5)  [unwired: 5 in]
              n281 = call "RS_SMBV100A_Error_check.vi"("Driver Name"=w904, "Error Code"=w905, "Error In"=w901, "DriverConnect in"=w902) -> ("Error Out"=w900:errorcluster)  [unwired: 6 in, 1 out]
            }
            frame "---------------------------- TIME_CONVERSION_CONFIGURATION  ----------------------------" {
            }
            frame "TIME_CONVERSION_CONFIGURATION_SIMULATE_LEAP_SECOND_TRANSITION", "TIMECONVERSIONCONFIGURATION_SIMULATELEAPSECONDTRANSITION" {
              # "SOUR:BB:GLON:NAVigation:TCONversion:LEAP:SLST ON"
              n282 = Unbundle By Name(w914) -> ("BASEBAND"=w917:string)
              n283 = call "MLLF_ParameterSelect.vi"("Command to equipment"=string[] ["ON\n", "OFF"], "Names"=string[][] [["ON", "1", "ENABLE", "EN"], ["OFF", "0", "DISABLE", "DIS"]], "Input"=w913, "Command"=w912, "Driver Name"=w911, "Error Code"=w910) -> ("Choice"=w915:string, "Error Out"=w924:errorcluster)  [unwired: 8 in]
              n284 = Concatenate Strings("SOUR:BB:", w917, ":NAVigation:TCONversion:LEAP:SLST ", w915) -> (w916:string)
              n285 = call "MLLF_WriteToBuffer.vi"("String"=w916, "error in"=w924, "DriverConnect in"=w921) -> ("error out"=w922:T15, "DriverConnect out"=w923:T5)  [unwired: 5 in]
              n286 = call "RS_SMBV100A_Error_check.vi"("Driver Name"=w911, "Error Code"=w910, "Error In"=w922, "DriverConnect in"=w923) -> ("Error Out"=w920:errorcluster)  [unwired: 6 in, 1 out]
            }
            frame "TIME_CONVERSION_CONFIGURATION_CURRENT_LEAP_SECONDS", "TIMECONVERSIONCONFIGURATION_CURRENTLEAPSECONDS" {
              n287 = call "MLLF_FormatStringValue.vi"("String Value"=w927, "Format"=" %.;%1.7f" ("format")) -> ("error out"=w937:T15, "String Value Formated"=w938:T16)  [unwired: 7 in, 1 out]
              n288 = Unbundle By Name(w930) -> ("BASEBAND"=w929:string)
              n289 = Concatenate Strings("SOUR:BB:", w929, ":NAVigation:TCONversion:LEAP:SEC " ("string"), w938) -> (w932:string)
              n290 = call "MLLF_WriteToBuffer.vi"("String"=w932, "error in"=w937, "DriverConnect in"=w936) -> ("error out"=w940:T15, "DriverConnect out"=w941:T5)  [unwired: 5 in]
              n291 = call "RS_SMBV100A_Error_check.vi"("Driver Name"=w933, "Error Code"=w934, "Error In"=w940, "DriverConnect in"=w941) -> ("Error Out"=w935:errorcluster)  [unwired: 6 in, 1 out]
            }
            frame "TIME_CONVERSION_CONFIGURATION_SYNCHRONIZE", "TIMECONVERSIONCONFIGURATION_SYNCHRONIZE" {
              n292 = Unbundle By Name(w942) -> ("BASEBAND"=w945:string)
              n293 = Concatenate Strings("SOUR:BB:", w945, ":NAVigation:TCONversion:LEAP:SYNC" ("string")) -> (w943:string)
              n294 = call "MLLF_WriteToBuffer.vi"("String"=w943, "DriverConnect in"=w950) -> ("error out"=w951:T15, "DriverConnect out"=w952:T5)  [unwired: 6 in]
              n295 = call "RS_SMBV100A_Error_check.vi"("Driver Name"=w948, "Error Code"=w949, "Error In"=w951, "DriverConnect in"=w952) -> ("Error Out"=w947:errorcluster)  [unwired: 6 in, 1 out]
            }
            frame "---------------------------------------  VEHICLE ------------------------------------------" {
            }
            frame "VEHICLE_DESCRIPTION_FILE", "VEHICLEDESCRIPTIONFILE" {
              w967 = "\"" ("string")
              # "Выбор СВОЙСТВА средства передвижения GLON приемника"
              n296 = Search and Replace String(replace all?=TRUE, input string=w960, search string="\"", replace string="") -> (result string=w959:string)  [unwired: 4 in, 3 out]
              n297 = Unbundle By Name(w954) -> ("BASEBAND"=w957:string)
              n298 = Concatenate Strings("/hdd/GNSS/vehicle/" ("string"), w959, ".xvd" ("string")) -> (w965:string)
              n299 = Concatenate Strings(":VEHicle:FILE " ("string"), w967, w965, w967) -> (w955:string)
              n300 = Concatenate Strings("SOURce1:BB:", w957, w955) -> (w956:string)
              n301 = call "MLLF_WriteToBuffer.vi"("String"=w956, "DriverConnect in"=w972) -> ("error out"=w970:T15, "DriverConnect out"=w971:T5)  [unwired: 6 in]
              n302 = call "RS_SMBV100A_Error_check.vi"("Driver Name"=w973, "Error Code"=w974, "Error In"=w970, "DriverConnect in"=w971) -> ("Error Out"=w969:errorcluster)  [unwired: 6 in, 1 out]
            }
            frame "VEHICLE_TYPE", "VEHICLETYPE" {
              # "Выбор средства передвижения GLON приемника"
              n303 = Unbundle By Name(w979) -> ("BASEBAND"=w982:string)
              n304 = call "MLLF_ParameterSelect.vi"("Command to equipment"=string[] ["PEDESTRIAN", "LAND VEHICLE", "SHIP", "AIRCRAFT", "SPACECRAFT", "HIL"], "Names"=string[][] [["PEDESTRIAN"], ["LAND VEHICLE"], ["SHIP"], ["AIRCRAFT"], ["SPACECRAFT"], ["HIL"]], "Input"=w976, "Command"=w975, "Driver Name"=w977, "Error Code"=w978) -> ("Choice"=w980:string, "Error Out"=w988:errorcluster)  [unwired: 8 in]
              n305 = Concatenate Strings("SOUR:BB:", w982, ":VEH:TYPE ", w980) -> (w981:string)
              n306 = call "MLLF_WriteToBuffer.vi"("String"=w981, "error in"=w988, "DriverConnect in"=w987) -> ("error out"=w985:T15, "DriverConnect out"=w986:T5)  [unwired: 5 in]
              n307 = call "RS_SMBV100A_Error_check.vi"("Driver Name"=w977, "Error Code"=w978, "Error In"=w985, "DriverConnect in"=w986) -> ("Error Out"=w991:errorcluster)  [unwired: 6 in, 1 out]
            }
            frame "----- LOAD SCENARIO -----" {
              # "Функции настройки в локации GPS"
            }
            frame "GPS_LOAD_SCENARIO" {
              w1012 = "'" ("string")
              # "Осуществляется подгрузка и в прибор и в драйвер сценария."
              # "загружаем сценарий для локации GPS"
              n308 = Search and Replace String(replace all?=TRUE, input string=w994, search string="\"", replace string="") -> (result string=w995:string)  [unwired: 4 in, 3 out]
              n309 = Concatenate Strings("GNSS\\scenario\\", w995) -> (w1003:string)
              n310 = Build Path(base path=w993, name or relative path=w1003) -> (appended path=w999:path)
              n311 = Concatenate Strings("/hdd/GNSS/scenario/", w995) -> (w1000:string)
              n312 = Read from Text File(file (use dialog)=w999) -> (text=w1016:string, error out=w1007:errorcluster)  [unwired: 3 in, 2 out]
              n313 = Bundle By Name(cluster=w1015, "GPS SCENARIO"=w1016) -> (w1014:T12)
              n314 = Concatenate Strings("SOUR:BB:GPS:LOC:WAYP:FILE " ("string"), w1012, w1000, w1012) -> (w1009:string)
              n315 = call "MLLF_WriteToBuffer.vi"("String"=w1009, "error in"=w1007, "DriverConnect in"=w1008) -> ("error out"=w1010:T15, "DriverConnect out"=w1011:T5)  [unwired: 5 in]
              n316 = call "RS_SMBV100A_Error_check.vi"("Driver Name"=w1004, "Error Code"=w1005, "Error In"=w1010, "DriverConnect in"=w1011) -> ("Error Out"=w1006:errorcluster)  [unwired: 6 in, 1 out]
            }
            frame "GPS_LOAD_WAYPOINTS" {
              # "Импортируем WAYPOINTS в драйвер"
              n317 = Search and Replace String(replace all?=TRUE, input string=w1020, search string="\"", replace string="") -> (result string=w1019:string)  [unwired: 4 in, 3 out]
              n318 = Concatenate Strings("GNSS\\waypoints\\", w1019) -> (w1031:string)
              n319 = Build Path(base path=w1017, name or relative path=w1031) -> (appended path=w1029:path)
              n320 = Read from Text File(file (use dialog)=w1029) -> (text=w1018:string, error out=w1026:errorcluster)  [unwired: 3 in, 2 out]
              n321 = call "RS_SMBV100A_arrayStringToDOUBLE.vi"("string"=w1018, "error in"=w1026) -> ("Dynam waypoints"=w1024:T10, "error out"=w1025:errorcluster)  [unwired: 1 in]
              n322 = Bundle By Name(cluster=w1028, "GPS WAYPOINTS"=w1024, "GPS WAYPOINTS STRING"=w1018) -> (w1027:T12)
            }
            frame "----- Standart Function -----" {
              # "Стандартные функции"
            }
            frame "LEVEL", "RF_LEVEL_AMPLITUDE" {
              # "Уровень выходного сигнала в dBm"
              n323 = call "MLLF_FormatStringValue.vi"("String Value"=w1036, "Format"=" %.;%1.2f" ("format")) -> ("error out"=w1035:T15, "String Value Formated"=w1037:T16)  [unwired: 7 in, 1 out]
              n324 = Concatenate Strings("SOUR:POW:LEV:IMM:AMPL " ("string"), w1037, " dBm" ("string")) -> (w1034:string)
              n325 = call "MLLF_WriteToBuffer.vi"("String"=w1034, "error in"=w1035, "DriverConnect in"=w1043) -> ("error out"=w1041:T15, "DriverConnect out"=w1042:T5)  [unwired: 5 in]
              n326 = call "RS_SMBV100A_Error_check.vi"("Driver Name"=w1044, "Error Code"=w1045, "Error In"=w1041, "DriverConnect in"=w1042) -> ("Error Out"=w1040:errorcluster)  [unwired: 6 in, 1 out]
            }
            frame "PRESET", "RESET" {
              # "Сбрасывает прибор в состояние с начальными установками. Синтаксис: PRESET"
              n327 = call "MLLF_WriteToBufferWithDelay.vi"("Delay Time ( 0,05 s)"=3.0, "Command"="*RST" ("String"), "DriverConnect in"=w1050) -> ("Error Out"=w1053:errorcluster, "DriverConnect out"=w1054:T5)  [unwired: 7 in]
              n328 = call "RS_SMBV100A_Error_check.vi"("Driver Name"=w1048, "Error Code"=w1049, "Error In"=w1053, "DriverConnect in"=w1054) -> ("Error Out"=w1047:errorcluster)  [unwired: 6 in, 1 out]
            }
            frame "SHUTDOWN" {
              # "Сбрасывает прибор в состояние с начальными установками. Синтаксис: PRESET"
              n329 = call "MLLF_WriteToBufferWithDelay.vi"("Command"="SYST:SHUT" ("String"), "DriverConnect in"=w1059) -> ("Error Out"=w1061:errorcluster, "DriverConnect out"=w1062:T5)  [unwired: 8 in]
              n330 = call "RS_SMBV100A_Error_check.vi"("Driver Name"=w1057, "Error Code"=w1058, "Error In"=w1061, "DriverConnect in"=w1062) -> ("Error Out"=w1056:errorcluster)  [unwired: 6 in, 1 out]
            }
            frame "REBOOT" {
              # "Сбрасывает прибор в состояние с начальными установками. Синтаксис: PRESET"
              n331 = call "MLLF_WriteToBufferWithDelay.vi"("Command"="SYST:REB" ("String"), "DriverConnect in"=w1067) -> ("Error Out"=w1069:errorcluster, "DriverConnect out"=w1070:T5)  [unwired: 8 in]
              n332 = call "RS_SMBV100A_Error_check.vi"("Driver Name"=w1065, "Error Code"=w1066, "Error In"=w1069, "DriverConnect in"=w1070) -> ("Error Out"=w1064:errorcluster)  [unwired: 6 in, 1 out]
            }
            frame "RESTART" {
              # "Сбрасывает прибор в состояние с начальными установками. Синтаксис: PRESET"
              n333 = call "MLLF_WriteToBufferWithDelay.vi"("Command"="SYST:REST" ("String"), "DriverConnect in"=w1075) -> ("Error Out"=w1077:errorcluster, "DriverConnect out"=w1078:T5)  [unwired: 8 in]
              n334 = call "RS_SMBV100A_Error_check.vi"("Driver Name"=w1073, "Error Code"=w1074, "Error In"=w1077, "DriverConnect in"=w1078) -> ("Error Out"=w1072:errorcluster)  [unwired: 6 in, 1 out]
            }
            frame "RF" {
              # "ка = щт щаа"
              # "Включение\\Выключение блока RF\\A Mod"
              n335 = call "MLLF_ParameterSelect.vi"("Command to equipment"=string[] ["OUTP:STAT ON", "OUTP:STAT OFF"], "Names"=string[][] [["ON"], ["OFF"]], "Input"=w1081, "Command"=w1080, "Driver Name"=w1086, "Error Code"=w1087) -> ("Choice"=w1088:string, "Error Out"=w1089:errorcluster)  [unwired: 8 in]
              n336 = call "MLLF_WriteToBuffer.vi"("String"=w1088, "error in"=w1089, "DriverConnect in"=w1085) -> ("error out"=w1083:T15, "DriverConnect out"=w1084:T5)  [unwired: 5 in]
              n337 = call "RS_SMBV100A_Error_check.vi"("Driver Name"=w1086, "Error Code"=w1087, "Error In"=w1083, "DriverConnect in"=w1084) -> ("Error Out"=w1082:errorcluster)  [unwired: 6 in, 1 out]
            }
            frame "RF_LEVEL_LIMIT" {
              # "Уровень LIMITA PEP выходного сигнала в dBm"
              n338 = call "MLLF_FormatStringValue.vi"("String Value"=w1096, "Format"=" %.;%1.2f" ("format")) -> ("error out"=w1095:T15, "String Value Formated"=w1097:T16)  [unwired: 7 in, 1 out]
              n339 = Concatenate Strings("SOUR:POW:LIM:AMPL " ("string"), w1097, " dBm" ("string")) -> (w1094:string)
              n340 = call "MLLF_WriteToBuffer.vi"("String"=w1094, "error in"=w1095, "DriverConnect in"=w1103) -> ("error out"=w1101:T15, "DriverConnect out"=w1102:T5)  [unwired: 5 in]
              n341 = call "RS_SMBV100A_Error_check.vi"("Driver Name"=w1104, "Error Code"=w1105, "Error In"=w1101, "DriverConnect in"=w1102) -> ("Error Out"=w1100:errorcluster)  [unwired: 6 in, 1 out]
            }
            frame "SCPI" {
              # "Уровень LIMITA PEP выходного сигнала в dBm"
              n342 = call "MLLF_WriteToBuffer.vi"("String"=w1107, "DriverConnect in"=w1111) -> ("error out"=w1109:T15, "DriverConnect out"=w1110:T5)  [unwired: 6 in]
              n343 = call "RS_SMBV100A_Error_check.vi"("Driver Name"=w1112, "Error Code"=w1113, "Error In"=w1109, "DriverConnect in"=w1110) -> ("Error Out"=w1108:errorcluster)  [unwired: 6 in, 1 out]
            }
            frame "TIMEOUT" {
              # "Время ожидания ответа от прибора."
              n344 = call "MLLF_FormatStringValue.vi"("String Value"=w1115) -> ("error out"=w1122:T15, "number"=w1121:dbl)  [unwired: 8 in, 1 out]
              n345 = In Range and Coerce(upper limit=60000, x=w1121, lower limit=50) -> (coerced(x)=w1125:dbl, In Range?=w1123:bool)
              n346 = case shown="False" w1123 {
                tunnel: [w1134 _] -> w1124
                tunnel: w1119 -> [w1133 _]
                tunnel: w1120 -> [w1132 _]
                frame False {
                  n347 = Format Into String(format string="Ошибка команды: %s.\nTimeOut должен быть в пределах 50 - 60000", w1132) -> (resulting string=w1136:string)  [unwired: 2 in, 1 out]
                  n348 = Add(x=w1133, y=0) -> (x+y=w1137:T3)
                  n349 = Bundle By Name(cluster=errorcluster {"status"=TRUE, "code"=0, "source"=""} ("error out"), "code"=w1137, "source"=w1136) -> (w1134:errorcluster)
                }
                frame True {
                }
              }
              n350 = case shown="No Error" w1122 {
                tunnel: [w1130 w1131] -> w1116
                tunnel: w1117 -> [w1129 w1131]
                tunnel: w1125 -> [w1128 _]
                frame No Error {
                  n351 = Bundle By Name(cluster=w1129, "Connect.InterfaceSettings.TMO, ms"=w1128) -> (w1130:T12)
                }
                frame Error {
                }
              }
              n352 = Merge Errors(w1122, w1124) -> (w1118:errorcluster)
            }
          }
        }
        frame "get" {
          # "Тут реализованы функции DriverGet"
          n353 = Unbundle By Name(w1154) -> ("Connect"=w1148:T5)
          n354 = call "MLLF_CommandDelimeter.vi"("command with param"=w1155) -> ("param 1"=w1140:string, "command"=w1141:string)  [unwired: 6 in, 3 out]
          n355 = case shown="\"GNSS_N_SKY_SORTED_MAXTOMIN\"" w1141 {
            selector: w1141 -> [w1157 _ _ _ _ _ _ _ _ _ _ _ _ _ _ _ _ _ _ _ _ _ _ _ _ _ _ _ _ _ _ _ _ _ _ _ _ _ _ _ _ _ _ _ _ _ _ _ _ _ _ _ _ _ _ _ _ _ _ _ _ _ _]
            tunnel: [w1156 _ _ w1175 w1189 w1203 _ _ _ w1224 w1240 w1256 w1271 w1287 w1303 w1319 w1335 w1351 w1367 w1383 w1399 w1415 w1431 w1447 w1463 w1479 w1495 w1511 w1527 w1543 _ w1575 w1593 w1617 w1629 w1642 w1682 w1718 w1742 w1754 w1785 _ w1797 w1808 w1819 w1830 w1841 w1852 w1863 w1874 w1885 w1896 w1907 w1918 w1929 w1940 w1951 w1962 w1973 w1984 w1990 w2007 w2018] -> w1147
            tunnel: w1152 -> [_ _ _ _ _ _ _ _ _ w1226 w1242 w1258 w1273 w1289 w1305 w1321 w1337 w1353 w1369 w1385 w1401 w1417 w1433 w1449 w1465 w1481 w1497 w1513 w1529 w1545 _ w1577 w1595 w1619 w1631 w1641 w1681 w1717 w1741 w1753 w1787 _ w1799 w1810 w1821 w1832 w1843 w1854 w1865 w1876 w1887 w1898 w1909 w1920 w1931 w1942 w1953 w1964 w1975 w1986 w1998 w2009 w2020]
            tunnel: [w1160 w1163 w1164 w1174 w1188 w1202 w1211 w1212 w1213 w1215 w1231 w1247 w1264 w1279 w1295 w1311 w1327 w1344 w1359 w1375 w1392 w1408 w1424 w1440 w1456 w1471 w1487 w1503 w1519 w1535 w1550 w1551 w1578 w1613 w1621 w1634 w1665 w1705 w1722 w1746 w1777 w1788 w1790 w1802 w1813 w1824 w1834 w1845 w1856 w1867 w1878 w1889 w1900 w1911 w1922 w1933 w1944 w1955 w1966 w1977 w1988 w2000 w2011] -> w1153
            tunnel: w1154 -> [w1160 w1163 w1164 w1174 w1188 w1202 w1211 w1212 w1213 w1215 w1231 w1247 w1264 w1279 w1295 w1311 w1327 w1344 w1359 w1375 w1392 w1408 w1424 w1440 w1456 w1471 w1487 w1503 w1519 w1535 w1550 w1551 w1578 w1613 w1621 w1634 w1665 w1705 w1722 w1746 w1777 w1788 w1790 w1802 w1813 w1824 w1834 w1845 w1856 w1867 w1878 w1889 w1900 w1911 w1922 w1933 w1944 w1955 w1966 w1977 w1988 w2000 w2011]
            tunnel: [w1158 w1161 _ _ _ _ _ _ _ w1223 w1239 w1255 w1265 w1282 w1297 w1313 w1329 w1346 w1362 w1379 w1393 w1410 w1426 w1442 w1458 w1473 w1489 w1506 w1521 w1537 _ w1574 _ _ _ _ _ w1713 w1737 _ w1784 _ w1796 w1807 w1818 w1826 w1837 w1848 w1858 w1870 w1881 w1892 w1903 w1914 w1924 w1936 w1947 w1958 w1969 w1980 _ w2003 w2014] -> w1149
            tunnel: w1148 -> [_ _ _ w1176 w1190 w1204 _ _ _ w1222 w1238 w1254 w1270 w1286 w1302 w1318 w1334 w1350 w1366 w1382 w1398 w1414 w1430 w1446 w1462 w1478 w1494 w1510 w1526 w1542 _ w1573 w1591 w1603 w1625 w1638 w1673 w1710 w1732 w1750 w1783 _ w1795 w1806 w1817 w1829 w1840 w1851 w1862 w1873 w1884 w1895 w1906 w1917 w1928 w1939 w1950 w1961 w1972 w1983 w1996 w2006 w2017]
            tunnel: w1151 -> [_ _ _ _ _ _ _ _ _ w1225 w1241 w1257 w1272 w1288 w1304 w1320 w1336 w1352 w1368 w1384 w1400 w1416 w1432 w1448 w1464 w1480 w1496 w1512 w1528 w1544 _ w1576 w1594 w1618 w1630 w1640 w1680 w1716 w1740 w1752 w1786 _ w1798 w1809 w1820 w1831 w1842 w1853 w1864 w1875 w1886 w1897 w1908 w1919 w1930 w1941 w1952 w1963 w1974 w1985 w1997 w2008 w2019]
            tunnel: [_ _ _ w1167 w1184 w1199 _ _ _ _ _ _ _ _ _ _ _ _ _ _ _ _ _ _ _ _ _ _ _ _ _ _ w1587 w1606 w1626 w1660 w1700 _ _ w1772 _ _ _ _ _ _ _ _ _ _ _ _ _ _ _ _ _ _ _ _ w1994 _ _] -> w1144
            tunnel: w1140 -> [_ _ _ _ _ _ _ _ _ w1219 w1235 w1251 w1267 w1283 w1299 w1315 w1331 w1347 w1363 w1378 w1395 w1411 w1427 w1443 w1459 w1475 w1491 w1507 w1523 w1539 _ w1572 _ _ _ w1637 w1669 w1709 w1734 w1749 w1782 _ _ _ _ _ _ _ _ _ _ _ _ _ _ _ _ _ _ _ _ _ _]
            frame "False", Default {
              # "DEFAULT"
              n356 = call "MLLF_UnknownCommand(SubVI).vi"("Unknown command"=w1157) -> ("error out"=w1156:errorcluster)  [unwired: 10 in]
              n357 = Build Array(0 ("TimeOut")) -> (w1158:i32[])
            }
            frame "TIMEOUT" {
              # "Время ожидания ответа от прибора."
              n358 = Unbundle By Name(w1163) -> ("Connect.InterfaceSettings.TMO, ms"=w1162:i32)
              n359 = Build Array(w1162) -> (w1161:i32[])
            }
            frame "------ID-------" {
            }
            frame "model" {
              n360 = call "RS_SMBV100A_FASTQUERY.vi"("input"="*IDN?", "DriverConnect in"=w1176) -> ("Error Out"=w1175:errorcluster, "output"=w1173:string)  [unwired: 7 in, 1 out]
              n361 = for {
                N: 4 -> [_]
                shift-right: [w1178] -> _
                shift-left: w1173 -> [w1181]
                tunnel: [w1180] -> w1172 mode=indexing
                stop <- w1179 stop-if-true
                n362 = Match Pattern(string=w1181, regular expression=",") -> (before substring=w1180:string, after substring=w1178:string)  [unwired: 1 in, 2 out]
                n363 = Empty String/Path?(string/path=w1178) -> (empty?=w1179:bool)
              }
              n364 = Index Array(array=w1172, index #1=0 ("index"), index #2=1 ("index")) -> (element #1=w1170:string, element #2=w1168:string)
              n365 = Concatenate Strings(w1170, " " ("string"), w1168) -> (w1167:string)
            }
            frame "FW", "ver", "version" {
              n366 = call "RS_SMBV100A_FASTQUERY.vi"("input"="*IDN?", "DriverConnect in"=w1190) -> ("Error Out"=w1189:errorcluster, "output"=w1185:string)  [unwired: 7 in, 1 out]
              n367 = for {
                N: 4 -> [_]
                shift-right: [w1192] -> _
                shift-left: w1185 -> [w1195]
                tunnel: [w1194] -> w1187 mode=indexing
                stop <- w1193 stop-if-true
                n368 = Match Pattern(string=w1195, regular expression=",") -> (before substring=w1194:string, after substring=w1192:string)  [unwired: 1 in, 2 out]
                n369 = Empty String/Path?(string/path=w1192) -> (empty?=w1193:bool)
              }
              n370 = Index Array(array=w1187, index=3) -> (element=w1184:string)
            }
            frame "serial", "serialNum", "SN" {
              n371 = call "RS_SMBV100A_FASTQUERY.vi"("input"="*IDN?", "DriverConnect in"=w1204) -> ("Error Out"=w1203:errorcluster, "output"=w1198:string)  [unwired: 7 in, 1 out]
              n372 = for {
                N: 4 -> [_]
                shift-right: [w1206] -> _
                shift-left: w1198 -> [w1209]
                tunnel: [w1208] -> w1201 mode=indexing
                stop <- w1207 stop-if-true
                n373 = Match Pattern(string=w1209, regular expression=",") -> (before substring=w1208:string, after substring=w1206:string)  [unwired: 1 in, 2 out]
                n374 = Empty String/Path?(string/path=w1206) -> (empty?=w1207:bool)
              }
              n375 = Index Array(array=w1201, index=2) -> (element=w1199:string)
            }
            frame "----- BASEBAND -----" {
            }
            frame "----- GPS BASEBAND -----" {
            }
            frame "----- GPS BASEBAND MASS WITH SARTIROVKA-----" {
            }
            frame "GNNS_N_NUMBER_ACTIVE_SAT" {
              # "колличество активных спутников на Созвездии."
              n376 = Unbundle By Name(w1215) -> ("BASEBAND"=w1216:string)
              n377 = call "RS_SMBV100A_N_ASKCONFIGURATION.vi"("DriverConnect in"=w1222, "BASEBAND"=w1216, "mass"=w1219) -> ("wrong sat"=w1217:bool, "DriverConnect out"=w1221:T5, "Parsing Satelite"=w1214:T18, "Error Out"=w1220:errorcluster)  [unwired: 9 in]
              n378 = case shown="False" w1217 {
                tunnel: [0.0 ("OUT GNSS NUMBERACTIVESAT") w1229] -> w1218
                tunnel: w1214 -> [_ w1228]
                frame True {
                  # "Если Тру вернуть Ноль\nтогда в скрипте проверку делать"
                }
                frame False {
                  n379 = call "RS_SMBV100A_PARS_SAT_TIME_AND_NUMBER.vi"("Parsing Satelite"=w1228) -> ("OUT GNSS NUMBERACTIVESAT"=w1229:dbl)  [unwired: 13 in, 5 out]
                }
              }
              n380 = Build Array(w1218) -> (w1223:dbl[])
              n381 = call "RS_SMBV100A_Error_check.vi"("Driver Name"=w1225, "Error Code"=w1226, "Error In"=w1220, "DriverConnect in"=w1221) -> ("Error Out"=w1224:errorcluster)  [unwired: 6 in, 1 out]
            }
            frame "GPS_N_NUMBER_ACTIVE_SAT" {
              # "колличество активных спутников GPS на Созвездии."
              n382 = Unbundle By Name(w1231) -> ("BASEBAND"=w1232:string)
              n383 = call "RS_SMBV100A_N_ASKCONFIGURATION.vi"("DriverConnect in"=w1238, "BASEBAND"=w1232, "mass"=w1235) -> ("wrong sat"=w1233:bool, "DriverConnect out"=w1237:T5, "Parsing Satelite"=w1230:T18, "Error Out"=w1236:errorcluster)  [unwired: 9 in]
              n384 = case shown="False" w1233 {
                tunnel: [0.0 ("OUT GNSS NUMBERACTIVESAT") w1245] -> w1234
                tunnel: w1230 -> [_ w1244]
                frame True {
                  # "Если Тру вернуть Ноль\nтогда в скрипте проверку делать"
                }
                frame False {
                  n385 = call "RS_SMBV100A_PARS_SAT_TIME_AND_NUMBER.vi"("Parsing Satelite"=w1244) -> ("OUT GPS NUMBERACTIVESAT"=w1245:dbl)  [unwired: 13 in, 5 out]
                }
              }
              n386 = Build Array(w1234) -> (w1239:dbl[])
              n387 = call "RS_SMBV100A_Error_check.vi"("Driver Name"=w1241, "Error Code"=w1242, "Error In"=w1236, "DriverConnect in"=w1237) -> ("Error Out"=w1240:errorcluster)  [unwired: 6 in, 1 out]
            }
            frame "GLONASS_N_NUMBER_ACTIVE_SAT" {
              # "колличество активных спутников GLONASS на Созвездии."
              n388 = Unbundle By Name(w1247) -> ("BASEBAND"=w1248:string)
              n389 = call "RS_SMBV100A_N_ASKCONFIGURATION.vi"("DriverConnect in"=w1254, "BASEBAND"=w1248, "mass"=w1251) -> ("wrong sat"=w1250:bool, "DriverConnect out"=w1253:T5, "Parsing Satelite"=w1246:T18, "Error Out"=w1252:errorcluster)  [unwired: 9 in]
              n390 = case shown="False" w1250 {
                tunnel: [0.0 ("OUT GNSS NUMBERACTIVESAT") w1261] -> w1249
                tunnel: w1246 -> [_ w1260]
                frame True {
                  # "Если Тру вернуть Ноль\nтогда в скрипте проверку делать"
                }
                frame False {
                  n391 = call "RS_SMBV100A_PARS_SAT_TIME_AND_NUMBER.vi"("Parsing Satelite"=w1260) -> ("OUT GLONASS NUMBERACTIVESAT"=w1261:dbl)  [unwired: 13 in, 5 out]
                }
              }
              n392 = Build Array(w1249) -> (w1255:dbl[])
              n393 = call "RS_SMBV100A_Error_check.vi"("Driver Name"=w1257, "Error Code"=w1258, "Error In"=w1252, "DriverConnect in"=w1253) -> ("Error Out"=w1256:errorcluster)  [unwired: 6 in, 1 out]
            }
            frame "GNSS_N_SAT_SORTED_MINTOMAX" {
              # "Массив порядка спутников(не номеров собственных) по времени от наименьшего времени"
              n394 = Unbundle By Name(w1264) -> ("BASEBAND"=w1263:string)
              n395 = call "RS_SMBV100A_N_ASKCONFIGURATION.vi"("DriverConnect in"=w1270, "BASEBAND"=w1263, "mass"=w1267) -> ("wrong sat"=w1266:bool, "DriverConnect out"=w1269:T5, "Parsing Satelite"=w1262:T18, "Error Out"=w1268:errorcluster)  [unwired: 9 in]
              n396 = case shown="False" w1266 {
                tunnel: [dbl[] [0.0] ("GNSS_SatSkySortedMinToMax") w1277] -> w1265
                tunnel: w1262 -> [_ w1275]
                frame True {
                  # "Если Тру вернуть Ноль\nтогда в скрипте проверку делать"
                }
                frame False {
                  n397 = call "RS_SMBV100A_PARS_SAT_TIME_AND_NUMBER.vi"("Parsing Satelite"=w1275) -> ("GNSS 2D SAT"=w1276:dbl[][])  [unwired: 13 in, 5 out]
                  n398 = call "RS_SMBV100A_CONVERT_DATASAT_2D_to_N1D.vi"("2D DATA SAT"=w1276) -> ("GNSS_SatSortedMinToMax"=w1277:dbl[])  [unwired: 2 in, 5 out]
                }
              }
              n399 = call "RS_SMBV100A_Error_check.vi"("Driver Name"=w1272, "Error Code"=w1273, "Error In"=w1268, "DriverConnect in"=w1269) -> ("Error Out"=w1271:errorcluster)  [unwired: 6 in, 1 out]
            }
            frame "GPS_N_SAT_SORTED_MINTOMAX" {
              # "Массив порядка GPS спутников(не номеров собственных) по времени от наименьшего времени"
              n400 = Unbundle By Name(w1279) -> ("BASEBAND"=w1280:string)
              n401 = call "RS_SMBV100A_N_ASKCONFIGURATION.vi"("DriverConnect in"=w1286, "BASEBAND"=w1280, "mass"=w1283) -> ("wrong sat"=w1281:bool, "DriverConnect out"=w1285:T5, "Parsing Satelite"=w1278:T18, "Error Out"=w1284:errorcluster)  [unwired: 9 in]
              n402 = case shown="False" w1281 {
                tunnel: [dbl[] [0.0] ("GNSS_SatSkySortedMinToMax") w1292] -> w1282
                tunnel: w1278 -> [_ w1291]
                frame True {
                  # "Если Тру вернуть Ноль\nтогда в скрипте проверку делать"
                }
                frame False {
                  n403 = call "RS_SMBV100A_PARS_SAT_TIME_AND_NUMBER.vi"("Parsing Satelite"=w1291) -> ("GPS 2D SAT"=w1293:dbl[][])  [unwired: 13 in, 5 out]
                  n404 = call "RS_SMBV100A_CONVERT_DATASAT_2D_to_N1D.vi"("2D DATA SAT"=w1293) -> ("GNSS_SatSortedMinToMax"=w1292:dbl[])  [unwired: 2 in, 5 out]
                }
              }
              n405 = call "RS_SMBV100A_Error_check.vi"("Driver Name"=w1288, "Error Code"=w1289, "Error In"=w1284, "DriverConnect in"=w1285) -> ("Error Out"=w1287:errorcluster)  [unwired: 6 in, 1 out]
            }
            frame "GLONASS_N_SAT_SORTED_MINTOMAX" {
              # "Массив порядка GLONASS спутников(не номеров собственных) по времени от наименьшего времени"
              n406 = Unbundle By Name(w1295) -> ("BASEBAND"=w1296:string)
              n407 = call "RS_SMBV100A_N_ASKCONFIGURATION.vi"("DriverConnect in"=w1302, "BASEBAND"=w1296, "mass"=w1299) -> ("wrong sat"=w1298:bool, "DriverConnect out"=w1301:T5, "Parsing Satelite"=w1294:T18, "Error Out"=w1300:errorcluster)  [unwired: 9 in]
              n408 = case shown="False" w1298 {
                tunnel: [dbl[] [0.0] ("GNSS_SatSkySortedMinToMax") w1309] -> w1297
                tunnel: w1294 -> [_ w1307]
                frame True {
                  # "Если Тру вернуть Ноль\nтогда в скрипте проверку делать"
                }
                frame False {
                  n409 = call "RS_SMBV100A_PARS_SAT_TIME_AND_NUMBER.vi"("Parsing Satelite"=w1307) -> ("GLONASS 2D SAT"=w1308:dbl[][])  [unwired: 13 in, 5 out]
                  n410 = call "RS_SMBV100A_CONVERT_DATASAT_2D_to_N1D.vi"("2D DATA SAT"=w1308) -> ("GNSS_SatSortedMinToMax"=w1309:dbl[])  [unwired: 2 in, 5 out]
                }
              }
              n411 = call "RS_SMBV100A_Error_check.vi"("Driver Name"=w1304, "Error Code"=w1305, "Error In"=w1300, "DriverConnect in"=w1301) -> ("Error Out"=w1303:errorcluster)  [unwired: 6 in, 1 out]
            }
            frame "GNSS_N_TIME_SORTED_MINTOMAX" {
              # "Массив времен в секундах GNSS спутников - от наименьшего времени"
              n412 = Unbundle By Name(w1311) -> ("BASEBAND"=w1312:string)
              n413 = call "RS_SMBV100A_N_ASKCONFIGURATION.vi"("DriverConnect in"=w1318, "BASEBAND"=w1312, "mass"=w1315) -> ("wrong sat"=w1314:bool, "DriverConnect out"=w1317:T5, "Parsing Satelite"=w1310:T18, "Error Out"=w1316:errorcluster)  [unwired: 9 in]
              n414 = case shown="False" w1314 {
                tunnel: [dbl[] [0.0] ("GNSS_SatSkySortedMinToMax") w1324] -> w1313
                tunnel: w1310 -> [_ w1323]
                frame True {
                  # "Если Тру вернуть Ноль\nтогда в скрипте проверку делать"
                }
                frame False {
                  n415 = call "RS_SMBV100A_PARS_SAT_TIME_AND_NUMBER.vi"("Parsing Satelite"=w1323) -> ("GNSS 2D SAT"=w1325:dbl[][])  [unwired: 13 in, 5 out]
                  n416 = call "RS_SMBV100A_CONVERT_DATASAT_2D_to_N1D.vi"("2D DATA SAT"=w1325) -> ("GNSS_TimeSortedMinToMax"=w1324:dbl[])  [unwired: 2 in, 5 out]
                }
              }
              n417 = call "RS_SMBV100A_Error_check.vi"("Driver Name"=w1320, "Error Code"=w1321, "Error In"=w1316, "DriverConnect in"=w1317) -> ("Error Out"=w1319:errorcluster)  [unwired: 6 in, 1 out]
            }
            frame "GPS_N_TIME_SORTED_MINTOMAX" {
              # "Массив времен в секундах GPS спутников - от наименьшего времени"
              n418 = Unbundle By Name(w1327) -> ("BASEBAND"=w1328:string)
              n419 = call "RS_SMBV100A_N_ASKCONFIGURATION.vi"("DriverConnect in"=w1334, "BASEBAND"=w1328, "mass"=w1331) -> ("wrong sat"=w1330:bool, "DriverConnect out"=w1333:T5, "Parsing Satelite"=w1326:T18, "Error Out"=w1332:errorcluster)  [unwired: 9 in]
              n420 = case shown="False" w1330 {
                tunnel: [dbl[] [0.0] ("GNSS_SatSkySortedMinToMax") w1340] -> w1329
                tunnel: w1326 -> [_ w1339]
                frame True {
                  # "Если Тру вернуть Ноль\nтогда в скрипте проверку делать"
                }
                frame False {
                  n421 = call "RS_SMBV100A_PARS_SAT_TIME_AND_NUMBER.vi"("Parsing Satelite"=w1339) -> ("GPS 2D SAT"=w1341:dbl[][])  [unwired: 13 in, 5 out]
                  n422 = call "RS_SMBV100A_CONVERT_DATASAT_2D_to_N1D.vi"("2D DATA SAT"=w1341) -> ("GNSS_TimeSortedMinToMax"=w1340:dbl[])  [unwired: 2 in, 5 out]
                }
              }
              n423 = call "RS_SMBV100A_Error_check.vi"("Driver Name"=w1336, "Error Code"=w1337, "Error In"=w1332, "DriverConnect in"=w1333) -> ("Error Out"=w1335:errorcluster)  [unwired: 6 in, 1 out]
            }
            frame "GLONASS_N_TIME_SORTED_MINTOMAX" {
              # "Массив времен в секундах GLONASS спутников - от наименьшего времени"
              n424 = Unbundle By Name(w1344) -> ("BASEBAND"=w1343:string)
              n425 = call "RS_SMBV100A_N_ASKCONFIGURATION.vi"("DriverConnect in"=w1350, "BASEBAND"=w1343, "mass"=w1347) -> ("wrong sat"=w1345:bool, "DriverConnect out"=w1349:T5, "Parsing Satelite"=w1342:T18, "Error Out"=w1348:errorcluster)  [unwired: 9 in]
              n426 = case shown="False" w1345 {
                tunnel: [dbl[] [0.0] ("GNSS_SatSkySortedMinToMax") w1356] -> w1346
                tunnel: w1342 -> [_ w1355]
                frame True {
                  # "Если Тру вернуть Ноль\nтогда в скрипте проверку делать"
                }
                frame False {
                  n427 = call "RS_SMBV100A_PARS_SAT_TIME_AND_NUMBER.vi"("Parsing Satelite"=w1355) -> ("GLONASS 2D SAT"=w1357:dbl[][])  [unwired: 13 in, 5 out]
                  n428 = call "RS_SMBV100A_CONVERT_DATASAT_2D_to_N1D.vi"("2D DATA SAT"=w1357) -> ("GNSS_TimeSortedMinToMax"=w1356:dbl[])  [unwired: 2 in, 5 out]
                }
              }
              n429 = call "RS_SMBV100A_Error_check.vi"("Driver Name"=w1352, "Error Code"=w1353, "Error In"=w1348, "DriverConnect in"=w1349) -> ("Error Out"=w1351:errorcluster)  [unwired: 6 in, 1 out]
            }
            frame "GNSS_N_SKY_SORTED_MINTOMAX" {
              # "Массив номеров GNSS спутников на небе - от наименьшего времени"
              n430 = Unbundle By Name(w1359) -> ("BASEBAND"=w1360:string)
              n431 = call "RS_SMBV100A_N_ASKCONFIGURATION.vi"("DriverConnect in"=w1366, "BASEBAND"=w1360, "mass"=w1363) -> ("wrong sat"=w1361:bool, "DriverConnect out"=w1365:T5, "Parsing Satelite"=w1358:T18, "Error Out"=w1364:errorcluster)  [unwired: 9 in]
              n432 = case shown="False" w1361 {
                tunnel: [dbl[] [0.0] ("GNSS_SatSkySortedMinToMax") w1373] -> w1362
                tunnel: w1358 -> [_ w1371]
                frame True {
                  # "Если Тру вернуть Ноль\nтогда в скрипте проверку делать"
                }
                frame False {
                  n433 = call "RS_SMBV100A_PARS_SAT_TIME_AND_NUMBER.vi"("Parsing Satelite"=w1371) -> ("GNSS 2D SAT"=w1372:dbl[][])  [unwired: 13 in, 5 out]
                  n434 = call "RS_SMBV100A_CONVERT_DATASAT_2D_to_N1D.vi"("2D DATA SAT"=w1372) -> ("GNSS_SatSkySortedMinToMax"=w1373:dbl[])  [unwired: 2 in, 5 out]
                }
              }
              n435 = call "RS_SMBV100A_Error_check.vi"("Driver Name"=w1368, "Error Code"=w1369, "Error In"=w1364, "DriverConnect in"=w1365) -> ("Error Out"=w1367:errorcluster)  [unwired: 6 in, 1 out]
            }
            frame "GPS_N_SKY_SORTED_MINTOMAX" {
              # "Массив номеров GPS спутников на небе - от наименьшего времени"
              n436 = Unbundle By Name(w1375) -> ("BASEBAND"=w1376:string)
              n437 = call "RS_SMBV100A_N_ASKCONFIGURATION.vi"("DriverConnect in"=w1382, "BASEBAND"=w1376, "mass"=w1378) -> ("wrong sat"=w1377:bool, "DriverConnect out"=w1381:T5, "Parsing Satelite"=w1374:T18, "Error Out"=w1380:errorcluster)  [unwired: 9 in]
              n438 = case shown="False" w1377 {
                tunnel: [dbl[] [0.0] ("GNSS_SatSkySortedMinToMax") w1389] -> w1379
                tunnel: w1374 -> [_ w1387]
                frame True {
                  # "Если Тру вернуть Ноль\nтогда в скрипте проверку делать"
                }
                frame False {
                  n439 = call "RS_SMBV100A_PARS_SAT_TIME_AND_NUMBER.vi"("Parsing Satelite"=w1387) -> ("GPS 2D SAT"=w1388:dbl[][])  [unwired: 13 in, 5 out]
                  n440 = call "RS_SMBV100A_CONVERT_DATASAT_2D_to_N1D.vi"("2D DATA SAT"=w1388) -> ("GNSS_SatSkySortedMinToMax"=w1389:dbl[])  [unwired: 2 in, 5 out]
                }
              }
              n441 = call "RS_SMBV100A_Error_check.vi"("Driver Name"=w1384, "Error Code"=w1385, "Error In"=w1380, "DriverConnect in"=w1381) -> ("Error Out"=w1383:errorcluster)  [unwired: 6 in, 1 out]
            }
            frame "GLONASS_N_SKY_SORTED_MINTOMAX" {
              # "Массив номеров GLONASS спутников на небе - от наименьшего времени"
              n442 = Unbundle By Name(w1392) -> ("BASEBAND"=w1391:string)
              n443 = call "RS_SMBV100A_N_ASKCONFIGURATION.vi"("DriverConnect in"=w1398, "BASEBAND"=w1391, "mass"=w1395) -> ("wrong sat"=w1394:bool, "DriverConnect out"=w1397:T5, "Parsing Satelite"=w1390:T18, "Error Out"=w1396:errorcluster)  [unwired: 9 in]
              n444 = case shown="False" w1394 {
                tunnel: [dbl[] [0.0] ("GNSS_SatSkySortedMinToMax") w1404] -> w1393
                tunnel: w1390 -> [_ w1403]
                frame True {
                  # "Если Тру вернуть Ноль\nтогда в скрипте проверку делать"
                }
                frame False {
                  n445 = call "RS_SMBV100A_PARS_SAT_TIME_AND_NUMBER.vi"("Parsing Satelite"=w1403) -> ("GLONASS 2D SAT"=w1405:dbl[][])  [unwired: 13 in, 5 out]
                  n446 = call "RS_SMBV100A_CONVERT_DATASAT_2D_to_N1D.vi"("2D DATA SAT"=w1405) -> ("GNSS_SatSkySortedMinToMax"=w1404:dbl[])  [unwired: 2 in, 5 out]
                }
              }
              n447 = call "RS_SMBV100A_Error_check.vi"("Driver Name"=w1400, "Error Code"=w1401, "Error In"=w1396, "DriverConnect in"=w1397) -> ("Error Out"=w1399:errorcluster)  [unwired: 6 in, 1 out]
            }
            frame "GNSS_N_SAT_SORTED_MAXTOMIN" {
              # "Массив порядка спутников(не номеров собственных) по времени от наибольшего времени"
              n448 = Unbundle By Name(w1408) -> ("BASEBAND"=w1407:string)
              n449 = call "RS_SMBV100A_N_ASKCONFIGURATION.vi"("DriverConnect in"=w1414, "BASEBAND"=w1407, "mass"=w1411) -> ("wrong sat"=w1409:bool, "DriverConnect out"=w1413:T5, "Parsing Satelite"=w1406:T18, "Error Out"=w1412:errorcluster)  [unwired: 9 in]
              n450 = case shown="False" w1409 {
                tunnel: [dbl[] [0.0] ("GNSS_SatSkySortedMinToMax") w1421] -> w1410
                tunnel: w1406 -> [_ w1419]
                frame True {
                  # "Если Тру вернуть Ноль\nтогда в скрипте проверку делать"
                }
                frame False {
                  n451 = call "RS_SMBV100A_PARS_SAT_TIME_AND_NUMBER.vi"("Parsing Satelite"=w1419) -> ("GNSS 2D SAT"=w1420:dbl[][])  [unwired: 13 in, 5 out]
                  n452 = call "RS_SMBV100A_CONVERT_DATASAT_2D_to_N1D.vi"("2D DATA SAT"=w1420) -> ("GNSS_SatSortedMaxToMin"=w1421:dbl[])  [unwired: 2 in, 5 out]
                }
              }
              n453 = call "RS_SMBV100A_Error_check.vi"("Driver Name"=w1416, "Error Code"=w1417, "Error In"=w1412, "DriverConnect in"=w1413) -> ("Error Out"=w1415:errorcluster)  [unwired: 6 in, 1 out]
            }
            frame "GPS_N_SAT_SORTED_MAXTOMIN" {
              # "Массив порядка GPS спутников(не номеров собственных) по времени от наибольшего времени"
              n454 = Unbundle By Name(w1424) -> ("BASEBAND"=w1423:string)
              n455 = call "RS_SMBV100A_N_ASKCONFIGURATION.vi"("DriverConnect in"=w1430, "BASEBAND"=w1423, "mass"=w1427) -> ("wrong sat"=w1425:bool, "DriverConnect out"=w1429:T5, "Parsing Satelite"=w1422:T18, "Error Out"=w1428:errorcluster)  [unwired: 9 in]
              n456 = case shown="False" w1425 {
                tunnel: [dbl[] [0.0] ("GNSS_SatSkySortedMinToMax") w1436] -> w1426
                tunnel: w1422 -> [_ w1435]
                frame True {
                  # "Если Тру вернуть Ноль\nтогда в скрипте проверку делать"
                }
                frame False {
                  n457 = call "RS_SMBV100A_PARS_SAT_TIME_AND_NUMBER.vi"("Parsing Satelite"=w1435) -> ("GPS 2D SAT"=w1437:dbl[][])  [unwired: 13 in, 5 out]
                  n458 = call "RS_SMBV100A_CONVERT_DATASAT_2D_to_N1D.vi"("2D DATA SAT"=w1437) -> ("GNSS_SatSortedMaxToMin"=w1436:dbl[])  [unwired: 2 in, 5 out]
                }
              }
              n459 = call "RS_SMBV100A_Error_check.vi"("Driver Name"=w1432, "Error Code"=w1433, "Error In"=w1428, "DriverConnect in"=w1429) -> ("Error Out"=w1431:errorcluster)  [unwired: 6 in, 1 out]
            }
            frame "GLONASS_N_SAT_SORTED_MAXTOMIN" {
              # "Массив порядка GLONASS спутников(не номеров собственных) по времени от наибольшего времени"
              n460 = Unbundle By Name(w1440) -> ("BASEBAND"=w1439:string)
              n461 = call "RS_SMBV100A_N_ASKCONFIGURATION.vi"("DriverConnect in"=w1446, "BASEBAND"=w1439, "mass"=w1443) -> ("wrong sat"=w1441:bool, "DriverConnect out"=w1445:T5, "Parsing Satelite"=w1438:T18, "Error Out"=w1444:errorcluster)  [unwired: 9 in]
              n462 = case shown="False" w1441 {
                tunnel: [dbl[] [0.0] ("GNSS_SatSkySortedMinToMax") w1453] -> w1442
                tunnel: w1438 -> [_ w1451]
                frame True {
                  # "Если Тру вернуть Ноль\nтогда в скрипте проверку делать"
                }
                frame False {
                  n463 = call "RS_SMBV100A_PARS_SAT_TIME_AND_NUMBER.vi"("Parsing Satelite"=w1451) -> ("GLONASS 2D SAT"=w1452:dbl[][])  [unwired: 13 in, 5 out]
                  n464 = call "RS_SMBV100A_CONVERT_DATASAT_2D_to_N1D.vi"("2D DATA SAT"=w1452) -> ("GNSS_SatSortedMaxToMin"=w1453:dbl[])  [unwired: 2 in, 5 out]
                }
              }
              n465 = call "RS_SMBV100A_Error_check.vi"("Driver Name"=w1448, "Error Code"=w1449, "Error In"=w1444, "DriverConnect in"=w1445) -> ("Error Out"=w1447:errorcluster)  [unwired: 6 in, 1 out]
            }
            frame "GPS_N_TIME_SORTED_MAXTOMIN" {
              # "Массив времен в секундах GPS спутников- по времени от наибольшего времени"
              n466 = Unbundle By Name(w1456) -> ("BASEBAND"=w1455:string)
              n467 = call "RS_SMBV100A_N_ASKCONFIGURATION.vi"("DriverConnect in"=w1462, "BASEBAND"=w1455, "mass"=w1459) -> ("wrong sat"=w1457:bool, "DriverConnect out"=w1461:T5, "Parsing Satelite"=w1454:T18, "Error Out"=w1460:errorcluster)  [unwired: 9 in]
              n468 = case shown="False" w1457 {
                tunnel: [dbl[] [0.0] ("GNSS_SatSkySortedMinToMax") w1468] -> w1458
                tunnel: w1454 -> [_ w1467]
                frame True {
                  # "Если Тру вернуть Ноль\nтогда в скрипте проверку делать"
                }
                frame False {
                  n469 = call "RS_SMBV100A_PARS_SAT_TIME_AND_NUMBER.vi"("Parsing Satelite"=w1467) -> ("GPS 2D SAT"=w1469:dbl[][])  [unwired: 13 in, 5 out]
                  n470 = call "RS_SMBV100A_CONVERT_DATASAT_2D_to_N1D.vi"("2D DATA SAT"=w1469) -> ("GNSS_TimeSortedMaxToMin"=w1468:dbl[])  [unwired: 2 in, 5 out]
                }
              }
              n471 = call "RS_SMBV100A_Error_check.vi"("Driver Name"=w1464, "Error Code"=w1465, "Error In"=w1460, "DriverConnect in"=w1461) -> ("Error Out"=w1463:errorcluster)  [unwired: 6 in, 1 out]
            }
            frame "GNSS_N_TIME_SORTED_MAXTOMIN" {
              # "Массив времен в секундах GNSS спутников- по времени от наибольшего времени"
              n472 = Unbundle By Name(w1471) -> ("BASEBAND"=w1472:string)
              n473 = call "RS_SMBV100A_N_ASKCONFIGURATION.vi"("DriverConnect in"=w1478, "BASEBAND"=w1472, "mass"=w1475) -> ("wrong sat"=w1474:bool, "DriverConnect out"=w1477:T5, "Parsing Satelite"=w1470:T18, "Error Out"=w1476:errorcluster)  [unwired: 9 in]
              n474 = case shown="False" w1474 {
                tunnel: [dbl[] [0.0] ("GNSS_SatSkySortedMinToMax") w1484] -> w1473
                tunnel: w1470 -> [_ w1483]
                frame True {
                  # "Если Тру вернуть Ноль\nтогда в скрипте проверку делать"
                }
                frame False {
                  n475 = call "RS_SMBV100A_PARS_SAT_TIME_AND_NUMBER.vi"("Parsing Satelite"=w1483) -> ("GNSS 2D SAT"=w1485:dbl[][])  [unwired: 13 in, 5 out]
                  n476 = call "RS_SMBV100A_CONVERT_DATASAT_2D_to_N1D.vi"("2D DATA SAT"=w1485) -> ("GNSS_TimeSortedMaxToMin"=w1484:dbl[])  [unwired: 2 in, 5 out]
                }
              }
              n477 = call "RS_SMBV100A_Error_check.vi"("Driver Name"=w1480, "Error Code"=w1481, "Error In"=w1476, "DriverConnect in"=w1477) -> ("Error Out"=w1479:errorcluster)  [unwired: 6 in, 1 out]
            }
            frame "GLONASS_N_TIME_SORTED_MAXTOMIN" {
              # "Массив времен в секундах GLONASS спутников- по времени от наибольшего времени"
              n478 = Unbundle By Name(w1487) -> ("BASEBAND"=w1488:string)
              n479 = call "RS_SMBV100A_N_ASKCONFIGURATION.vi"("DriverConnect in"=w1494, "BASEBAND"=w1488, "mass"=w1491) -> ("wrong sat"=w1490:bool, "DriverConnect out"=w1493:T5, "Parsing Satelite"=w1486:T18, "Error Out"=w1492:errorcluster)  [unwired: 9 in]
              n480 = case shown="False" w1490 {
                tunnel: [dbl[] [0.0] ("GNSS_SatSkySortedMinToMax") w1501] -> w1489
                tunnel: w1486 -> [_ w1499]
                frame True {
                  # "Если Тру вернуть Ноль\nтогда в скрипте проверку делать"
                }
                frame False {
                  n481 = call "RS_SMBV100A_PARS_SAT_TIME_AND_NUMBER.vi"("Parsing Satelite"=w1499) -> ("GLONASS 2D SAT"=w1500:dbl[][])  [unwired: 13 in, 5 out]
                  n482 = call "RS_SMBV100A_CONVERT_DATASAT_2D_to_N1D.vi"("2D DATA SAT"=w1500) -> ("GNSS_TimeSortedMaxToMin"=w1501:dbl[])  [unwired: 2 in, 5 out]
                }
              }
              n483 = call "RS_SMBV100A_Error_check.vi"("Driver Name"=w1496, "Error Code"=w1497, "Error In"=w1492, "DriverConnect in"=w1493) -> ("Error Out"=w1495:errorcluster)  [unwired: 6 in, 1 out]
            }
            frame "GNSS_N_SKY_SORTED_MAXTOMIN" {
              # "Массив номеров GNSS спутников на небе - по времени от наибольшего времени"
              n484 = Unbundle By Name(w1503) -> ("BASEBAND"=w1504:string)
              n485 = call "RS_SMBV100A_N_ASKCONFIGURATION.vi"("DriverConnect in"=w1510, "BASEBAND"=w1504, "mass"=w1507) -> ("wrong sat"=w1505:bool, "DriverConnect out"=w1509:T5, "Parsing Satelite"=w1502:T18, "Error Out"=w1508:errorcluster)  [unwired: 9 in]
              n486 = case shown="False" w1505 {
                tunnel: [dbl[] [0.0] ("GNSS_SatSkySortedMinToMax") w1516] -> w1506
                tunnel: w1502 -> [_ w1515]
                frame True {
                  # "Если Тру вернуть Ноль\nтогда в скрипте проверку делать"
                }
                frame False {
                  n487 = call "RS_SMBV100A_PARS_SAT_TIME_AND_NUMBER.vi"("Parsing Satelite"=w1515) -> ("GNSS 2D SAT"=w1517:dbl[][])  [unwired: 13 in, 5 out]
                  n488 = call "RS_SMBV100A_CONVERT_DATASAT_2D_to_N1D.vi"("2D DATA SAT"=w1517) -> ("GNSS_SatSkySortedMaxToMin"=w1516:dbl[])  [unwired: 2 in, 5 out]
                }
              }
              n489 = call "RS_SMBV100A_Error_check.vi"("Driver Name"=w1512, "Error Code"=w1513, "Error In"=w1508, "DriverConnect in"=w1509) -> ("Error Out"=w1511:errorcluster)  [unwired: 6 in, 1 out]
            }
            frame "GPS_N_SKY_SORTED_MAXTOMIN" {
              # "Массив номеров GPS спутников на небе - по времени от наибольшего времени"
              n490 = Unbundle By Name(w1519) -> ("BASEBAND"=w1520:string)
              n491 = call "RS_SMBV100A_N_ASKCONFIGURATION.vi"("DriverConnect in"=w1526, "BASEBAND"=w1520, "mass"=w1523) -> ("wrong sat"=w1522:bool, "DriverConnect out"=w1525:T5, "Parsing Satelite"=w1518:T18, "Error Out"=w1524:errorcluster)  [unwired: 9 in]
              n492 = case shown="False" w1522 {
                tunnel: [dbl[] [0.0] ("GNSS_SatSkySortedMinToMax") w1533] -> w1521
                tunnel: w1518 -> [_ w1531]
                frame True {
                  # "Если Тру вернуть Ноль\nтогда в скрипте проверку делать"
                }
                frame False {
                  n493 = call "RS_SMBV100A_PARS_SAT_TIME_AND_NUMBER.vi"("Parsing Satelite"=w1531) -> ("GPS 2D SAT"=w1532:dbl[][])  [unwired: 13 in, 5 out]
                  n494 = call "RS_SMBV100A_CONVERT_DATASAT_2D_to_N1D.vi"("2D DATA SAT"=w1532) -> ("GNSS_SatSkySortedMaxToMin"=w1533:dbl[])  [unwired: 2 in, 5 out]
                }
              }
              n495 = call "RS_SMBV100A_Error_check.vi"("Driver Name"=w1528, "Error Code"=w1529, "Error In"=w1524, "DriverConnect in"=w1525) -> ("Error Out"=w1527:errorcluster)  [unwired: 6 in, 1 out]
            }
            frame "GLONASS_N_SKY_SORTED_MAXTOMIN" {
              # "Массив номеров GLONASS спутников на небе - по времени от наибольшего времени"
              n496 = Unbundle By Name(w1535) -> ("BASEBAND"=w1536:string)
              n497 = call "RS_SMBV100A_N_ASKCONFIGURATION.vi"("DriverConnect in"=w1542, "BASEBAND"=w1536, "mass"=w1539) -> ("wrong sat"=w1538:bool, "DriverConnect out"=w1541:T5, "Parsing Satelite"=w1534:T18, "Error Out"=w1540:errorcluster)  [unwired: 9 in]
              n498 = case shown="False" w1538 {
                tunnel: [dbl[] [0.0] ("GNSS_SatSkySortedMinToMax") w1548] -> w1537
                tunnel: w1534 -> [_ w1547]
                frame True {
                  # "Если Тру вернуть Ноль\nтогда в скрипте проверку делать"
                }
                frame False {
                  n499 = call "RS_SMBV100A_PARS_SAT_TIME_AND_NUMBER.vi"("Parsing Satelite"=w1547) -> ("GLONASS 2D SAT"=w1549:dbl[][])  [unwired: 13 in, 5 out]
                  n500 = call "RS_SMBV100A_CONVERT_DATASAT_2D_to_N1D.vi"("2D DATA SAT"=w1549) -> ("GNSS_SatSkySortedMaxToMin"=w1548:dbl[])  [unwired: 2 in, 5 out]
                }
              }
              n501 = call "RS_SMBV100A_Error_check.vi"("Driver Name"=w1544, "Error Code"=w1545, "Error In"=w1540, "DriverConnect in"=w1541) -> ("Error Out"=w1543:errorcluster)  [unwired: 6 in, 1 out]
            }
            frame "----- GLONASS BASEBAND -----" {
            }
            frame "EPHEMERISPARAMETERS_TOE" {
              # "спутник на небе"
              # "Возвращает время TOE от номера на небе спутника"
              n502 = Unbundle By Name(w1551) -> ("BASEBAND"=w1554:string)
              n503 = call "RS_SMBV100A_N_in_SKY_to_SAT_in_DEVICE.vi"("DriverConnect in"=w1573, "BASEBAND"=w1554, "String Value"=w1572) -> ("GNSS"=w1565:string, "DriverConnect out"=w1562:T5, "SATINSKY_for_DEVICE"=w1555:dbl, "Error Out"=w1564:errorcluster)  [unwired: 8 in, 1 out]
              n504 = Concatenate Strings(":" ("regular expression"), w1565) -> (w1567:string)
              n505 = Format Into String(format string="%.;%1.0f" ("format"), error in=w1564, w1555) -> (resulting string=w1569:string, error out=w1561:errorcluster)  [unwired: 1 in]
              n506 = Unbundle By Name(w1551) -> ("BASEBAND"=w1553:string)
              n507 = Concatenate Strings("SOUR:BB:" ("regular expression"), w1553, ":SVID" ("regular expression"), w1569, w1567, ":NMESsage:EPHemeris:TOE?" ("regular expression")) -> (w1563:string)
              n508 = call "RS_SMBV100A_FASTQUERY.vi"("input"=w1563, "Error In"=w1561, "DriverConnect in"=w1562) -> ("Error Out"=w1557:errorcluster, "DriverConnect out"=w1560:T5, "output"=w1559:string)  [unwired: 6 in]
              n509 = call "MLLF_FormatStringValue.vi"("error in"=w1557, "String Value"=w1559) -> ("error out"=w1556:T15, "number"=w1558:dbl)  [unwired: 7 in, 1 out]
              n510 = Build Array(w1558) -> (w1574:dbl[])
              n511 = call "RS_SMBV100A_Error_check.vi"("Driver Name"=w1576, "Error Code"=w1577, "Error In"=w1556, "DriverConnect in"=w1560) -> ("Error Out"=w1575:errorcluster)  [unwired: 6 in, 1 out]
            }
            frame "SIMULATIONDATE" {
              n512 = Unbundle By Name(w1578) -> ("BASEBAND"=w1581:string)
              n513 = Concatenate Strings("SOUR:BB:", w1581, ":NAV:SIM:DATE? " ("regular expression")) -> (w1579:string)
              n514 = call "RS_SMBV100A_FASTQUERY.vi"("input"=w1579, "DriverConnect in"=w1591) -> ("Error Out"=w1586:errorcluster, "DriverConnect out"=w1592:T5, "output"=w1588:string)  [unwired: 7 in]
              n515 = Scan From String(format string="%.;%<%d,%m,%Y>T", input string=w1588, error in=w1586) -> (error out=w1589:errorcluster, output 1=w1590:timestamp)  [unwired: 2 in, 2 out]
              n516 = Format Into String(format string="%,;%<%Y,%m,%d>T", error in=w1589, w1590) -> (resulting string=w1587:string, error out=w1585:errorcluster)  [unwired: 1 in]
              n517 = call "RS_SMBV100A_Error_check.vi"("Driver Name"=w1594, "Error Code"=w1595, "Error In"=w1585, "DriverConnect in"=w1592) -> ("Error Out"=w1593:errorcluster)  [unwired: 6 in, 1 out]
            }
            frame "CURRENTTIME" {
              w1600 = "SOUR:BB:"
              # "возвращает время в UTC"
              n518 = Unbundle By Name(w1613) -> ("BASEBAND"=w1599:string)
              n519 = Concatenate Strings(w1600, w1599, ":NAV:SIM:TIME? " ("regular expression")) -> (w1598:string)
              n520 = call "RS_SMBV100A_FASTQUERY.vi"("input"=w1598, "DriverConnect in"=w1603) -> ("DriverConnect out"=w1602:T5, "output"=w1597:string)  [unwired: 7 in, 1 out]
              n521 = Concatenate Strings(w1600, w1599, ":SPOT:NHOT? " ("regular expression")) -> (w1614:string)
              n522 = call "RS_SMBV100A_FASTQUERY.vi"("input"=w1614, "DriverConnect in"=w1602) -> ("Error Out"=w1604:errorcluster, "DriverConnect out"=w1616:T5, "output"=w1596:string)  [unwired: 7 in]
              n523 = call "MLLF_FormatStringValue.vi"("String Value"=w1596) -> ("number"=w1608:dbl)  [unwired: 8 in, 2 out]
              n524 = Scan From String(format string="%.;%<%H,%M,%S>T", input string=w1597, error in=w1604) -> (error out=w1611:errorcluster, output 1=w1609:timestamp)  [unwired: 2 in, 2 out]
              n525 = Add(x=w1609, y=w1608) -> (x+y=w1607:timestamp)
              n526 = Format Into String(format string="%.;%<%H,%M,%S%3u>T", error in=w1611, w1607) -> (resulting string=w1606:string, error out=w1605:errorcluster)  [unwired: 1 in]
              n527 = call "RS_SMBV100A_Error_check.vi"("Driver Name"=w1618, "Error Code"=w1619, "Error In"=w1605, "DriverConnect in"=w1616) -> ("Error Out"=w1617:errorcluster)  [unwired: 6 in, 1 out]
            }
            frame "SIMULATIONTIME" {
              n528 = Unbundle By Name(w1621) -> ("BASEBAND"=w1623:string)
              n529 = Concatenate Strings("SOUR:BB:", w1623, ":NAV:SIM:TIME? " ("regular expression")) -> (w1620:string)
              n530 = call "RS_SMBV100A_FASTQUERY.vi"("input"=w1620, "DriverConnect in"=w1625) -> ("Error Out"=w1628:errorcluster, "DriverConnect out"=w1627:T5, "output"=w1626:string)  [unwired: 7 in]
              n531 = call "RS_SMBV100A_Error_check.vi"("Driver Name"=w1630, "Error Code"=w1631, "Error In"=w1628, "DriverConnect in"=w1627) -> ("Error Out"=w1629:errorcluster)  [unwired: 6 in, 1 out]
            }
            frame "SATELLITECONFIGURATIONS_DURATION_UTC" {
              w1649 = " ," ("format")
              w1653 = "%1.0f" ("format")
              w1658 = 60.0 ("y")
              # "Определяет время в UTC спутника N(приборе)"
              n532 = Unbundle By Name(w1634) -> ("BASEBAND"=w1632:string)
              n533 = Concatenate Strings("SOUR:BB:", w1632, ":SAT" ("regular expression"), w1637, ":DUR? " ("regular expression")) -> (w1647:string)
              n534 = call "RS_SMBV100A_FASTQUERY.vi"("input"=w1647, "DriverConnect in"=w1638) -> ("Error Out"=w1636:errorcluster, "DriverConnect out"=w1639:T5, "output"=w1644:string)  [unwired: 7 in]
              n535 = call "MLLF_FormatStringValue.vi"("error in"=w1636, "String Value"=w1644) -> ("error out"=w1635:T15, "number"=w1659:dbl)  [unwired: 7 in, 1 out]
              n536 = Quotient & Remainder(x=w1659, y=w1658) -> (x-y*floor(x/y)=w1656:dbl, floor(x/y)=w1657:dbl)
              n537 = Quotient & Remainder(x=w1657, y=w1658) -> (x-y*floor(x/y)=w1655:dbl, floor(x/y)=w1654:dbl)
              n538 = Format Into String(format string=w1653, w1656) -> (resulting string=w1650:string)  [unwired: 2 in, 1 out]
              n539 = Format Into String(format string=w1653, w1655) -> (resulting string=w1651:string)  [unwired: 2 in, 1 out]
              n540 = Format Into String(format string=w1653, w1654) -> (resulting string=w1652:string)  [unwired: 2 in, 1 out]
              n541 = Concatenate Strings(w1652, w1649, w1651, w1649, w1650) -> (w1648:string)
              n542 = Scan From String(format string="%.;%<%H,%M,%S>T", input string=w1648, error in=w1635) -> (error out=w1661:errorcluster, output 1=w1663:timestamp)  [unwired: 2 in, 2 out]
              n543 = Format Into String(format string="%.;%<%H,%M,%S%3u>T", error in=w1661, w1663) -> (resulting string=w1660:string, error out=w1643:errorcluster)  [unwired: 1 in]
              n544 = call "RS_SMBV100A_Error_check.vi"("Driver Name"=w1640, "Error Code"=w1641, "Error In"=w1643, "DriverConnect in"=w1639) -> ("Error Out"=w1642:errorcluster)  [unwired: 6 in, 1 out]
            }
            frame "SATELLITECONFIGURATIONS_REAL_SAT_DURATION_UTC" {
              w1689 = " ," ("format")
              w1693 = "%1.0f" ("format")
              w1698 = 60.0 ("y")
              # "Определяет время в UTC спутника на небе"
              n545 = Unbundle By Name(w1665) -> ("BASEBAND"=w1666:string)
              n546 = call "RS_SMBV100A_N_in_SKY_to_SAT_in_DEVICE.vi"("DriverConnect in"=w1673, "BASEBAND"=w1666, "String Value"=w1669) -> ("DriverConnect out"=w1672:T5, "SAT"=w1675:dbl, "Error Out"=w1674:errorcluster)  [unwired: 8 in, 2 out]
              n547 = Unbundle By Name(w1665) -> ("BASEBAND"=w1667:string)
              n548 = Format Into String(format string="%.;%1.0f" ("format"), error in=w1674, w1675) -> (resulting string=w1670:string, error out=w1671:errorcluster)  [unwired: 1 in]
              n549 = Concatenate Strings("SOUR:BB:", w1667, ":SAT" ("regular expression"), w1670, ":DUR? " ("regular expression")) -> (w1687:string)
              n550 = call "RS_SMBV100A_FASTQUERY.vi"("input"=w1687, "Error In"=w1671, "DriverConnect in"=w1672) -> ("Error Out"=w1678:errorcluster, "DriverConnect out"=w1679:T5, "output"=w1684:string)  [unwired: 6 in]
              n551 = call "MLLF_FormatStringValue.vi"("error in"=w1678, "String Value"=w1684) -> ("error out"=w1677:T15, "number"=w1699:dbl)  [unwired: 7 in, 1 out]
              n552 = Quotient & Remainder(x=w1699, y=w1698) -> (x-y*floor(x/y)=w1696:dbl, floor(x/y)=w1697:dbl)
              n553 = Quotient & Remainder(x=w1697, y=w1698) -> (x-y*floor(x/y)=w1695:dbl, floor(x/y)=w1694:dbl)
              n554 = Format Into String(format string=w1693, w1696) -> (resulting string=w1690:string)  [unwired: 2 in, 1 out]
              n555 = Format Into String(format string=w1693, w1695) -> (resulting string=w1691:string)  [unwired: 2 in, 1 out]
              n556 = Format Into String(format string=w1693, w1694) -> (resulting string=w1692:string)  [unwired: 2 in, 1 out]
              n557 = Concatenate Strings(w1692, w1689, w1691, w1689, w1690) -> (w1688:string)
              n558 = Scan From String(format string="%.;%<%H,%M,%S>T", input string=w1688, error in=w1677) -> (error out=w1701:errorcluster, output 1=w1703:timestamp)  [unwired: 2 in, 2 out]
              n559 = Format Into String(format string="%.;%<%H,%M,%S%3u>T", error in=w1701, w1703) -> (resulting string=w1700:string, error out=w1683:errorcluster)  [unwired: 1 in]
              n560 = call "RS_SMBV100A_Error_check.vi"("Driver Name"=w1680, "Error Code"=w1681, "Error In"=w1683, "DriverConnect in"=w1679) -> ("Error Out"=w1682:errorcluster)  [unwired: 6 in, 1 out]
            }
            frame "SATELLITECONFIGURATIONS_DURATION_SEC" {
              # "Определяет время в UTC спутника N(в приборе)"
              n561 = Unbundle By Name(w1705) -> ("BASEBAND"=w1707:string)
              n562 = Concatenate Strings("SOUR:BB:", w1707, ":SAT" ("regular expression"), w1709, ":DUR? " ("regular expression")) -> (w1721:string)
              n563 = call "RS_SMBV100A_FASTQUERY.vi"("input"=w1721, "DriverConnect in"=w1710) -> ("Error Out"=w1711:errorcluster, "DriverConnect out"=w1715:T5, "output"=w1719:string)  [unwired: 7 in]
              n564 = call "MLLF_FormatStringValue.vi"("error in"=w1711, "String Value"=w1719) -> ("error out"=w1712:T15, "number"=w1714:dbl)  [unwired: 7 in, 1 out]
              n565 = call "RS_SMBV100A_Error_check.vi"("Driver Name"=w1716, "Error Code"=w1717, "Error In"=w1712, "DriverConnect in"=w1715) -> ("Error Out"=w1718:errorcluster)  [unwired: 6 in, 1 out]
              n566 = Build Array(w1714) -> (w1713:dbl[])
            }
            frame "SATELLITECONFIGURATIONS_REAL_SAT_DURATION_SEC" {
              # "Определяет время в UTC спутника на небе"
              n567 = Unbundle By Name(w1722) -> ("BASEBAND"=w1723:string)
              n568 = call "RS_SMBV100A_N_in_SKY_to_SAT_in_DEVICE.vi"("DriverConnect in"=w1732, "BASEBAND"=w1723, "String Value"=w1734) -> ("DriverConnect out"=w1733:T5, "SAT"=w1730:dbl, "Error Out"=w1729:errorcluster)  [unwired: 8 in, 2 out]
              n569 = Format Into String(format string="%.;%1.0f" ("format"), error in=w1729, w1730) -> (resulting string=w1727:string, error out=w1728:errorcluster)  [unwired: 1 in]
              n570 = Unbundle By Name(w1722) -> ("BASEBAND"=w1725:string)
              n571 = Concatenate Strings("SOUR:BB:", w1725, ":SAT" ("regular expression"), w1727, ":DUR? " ("regular expression")) -> (w1745:string)
              n572 = call "RS_SMBV100A_FASTQUERY.vi"("input"=w1745, "Error In"=w1728, "DriverConnect in"=w1733) -> ("Error Out"=w1735:errorcluster, "DriverConnect out"=w1739:T5, "output"=w1743:string)  [unwired: 6 in]
              n573 = call "MLLF_FormatStringValue.vi"("error in"=w1735, "String Value"=w1743) -> ("error out"=w1736:T15, "number"=w1738:dbl)  [unwired: 7 in, 1 out]
              n574 = call "RS_SMBV100A_Error_check.vi"("Driver Name"=w1740, "Error Code"=w1741, "Error In"=w1736, "DriverConnect in"=w1739) -> ("Error Out"=w1742:errorcluster)  [unwired: 6 in, 1 out]
              n575 = Build Array(w1738) -> (w1737:dbl[])
            }
            frame "SATELLITECONFIGURATIONS_DURATION" {
              w1761 = " ," ("format")
              w1765 = "%1.0f" ("format")
              w1770 = 60.0 ("y")
              # "Определяет время в UTC спутника N(приборе)"
              n576 = Unbundle By Name(w1746) -> ("BASEBAND"=w1747:string)
              n577 = Concatenate Strings("SOUR:BB:", w1747, ":SAT" ("regular expression"), w1749, ":DUR? " ("regular expression")) -> (w1759:string)
              n578 = call "RS_SMBV100A_FASTQUERY.vi"("input"=w1759, "DriverConnect in"=w1750) -> ("DriverConnect out"=w1751:T5, "output"=w1756:string)  [unwired: 7 in, 1 out]
              n579 = call "MLLF_FormatStringValue.vi"("String Value"=w1756) -> ("number"=w1771:dbl)  [unwired: 8 in, 2 out]
              n580 = Quotient & Remainder(x=w1771, y=w1770) -> (x-y*floor(x/y)=w1768:dbl, floor(x/y)=w1769:dbl)
              n581 = Quotient & Remainder(x=w1769, y=w1770) -> (x-y*floor(x/y)=w1767:dbl, floor(x/y)=w1766:dbl)
              n582 = Format Into String(format string=w1765, w1768) -> (resulting string=w1762:string)  [unwired: 2 in, 1 out]
              n583 = Format Into String(format string=w1765, w1767) -> (resulting string=w1763:string)  [unwired: 2 in, 1 out]
              n584 = Format Into String(format string=w1765, w1766) -> (resulting string=w1764:string)  [unwired: 2 in, 1 out]
              n585 = Concatenate Strings(w1764, w1761, w1763, w1761, w1762) -> (w1760:string)
              n586 = Scan From String(format string="%.;%<%H,%M,%S>T", input string=w1760) -> (error out=w1773:errorcluster, output 1=w1775:timestamp)  [unwired: 3 in, 2 out]
              n587 = Format Into String(format string="%.;%<%H,%M,%S%3u>T", error in=w1773, w1775) -> (resulting string=w1772:string, error out=w1755:errorcluster)  [unwired: 1 in]
              n588 = call "RS_SMBV100A_Error_check.vi"("Driver Name"=w1752, "Error Code"=w1753, "Error In"=w1755, "DriverConnect in"=w1751) -> ("Error Out"=w1754:errorcluster)  [unwired: 6 in, 1 out]
            }
            frame "GNNS_NUMBER_SAT_IN_SATELLITECONFIGURATIONS" {
              # "Отдает порядковый номер спутника в устройстве по номеру на Небе"
              n589 = Unbundle By Name(w1777) -> ("BASEBAND"=w1778:string)
              n590 = call "RS_SMBV100A_N_in_SKY_to_SAT_in_DEVICE.vi"("DriverConnect in"=w1783, "BASEBAND"=w1778, "String Value"=w1782) -> ("DriverConnect out"=w1780:T5, "SAT"=w1781:dbl, "Error Out"=w1779:errorcluster)  [unwired: 8 in, 2 out]
              n591 = Build Array(w1781) -> (w1784:dbl[])
              n592 = call "RS_SMBV100A_Error_check.vi"("Driver Name"=w1786, "Error Code"=w1787, "Error In"=w1779, "DriverConnect in"=w1780) -> ("Error Out"=w1785:errorcluster)  [unwired: 6 in, 1 out]
            }
            frame "----- GLONASS BASEBAND MASS -----" {
            }
            frame "GNNS_NUMBER_ACTIVE_SAT" {
              # "колличество активных спутников на Созвездии."
              n593 = Unbundle By Name(w1790) -> ("BASEBAND"=w1791:string)
              n594 = call "RS_SMBV100A_ASKCONFIGURATION.vi"("DriverConnect in"=w1795, "BASEBAND"=w1791) -> ("DriverConnect out"=w1794:T5, "Parsing Satelite"=w1789:T18, "Error Out"=w1793:errorcluster)  [unwired: 11 in]
              n595 = call "RS_SMBV100A_PARS_SAT_TIME_AND_NUMBER.vi"("Parsing Satelite"=w1789) -> ("OUT GNSS NUMBERACTIVESAT"=w1792:dbl)  [unwired: 13 in, 5 out]
              n596 = Build Array(w1792) -> (w1796:dbl[])
              n597 = call "RS_SMBV100A_Error_check.vi"("Driver Name"=w1798, "Error Code"=w1799, "Error In"=w1793, "DriverConnect in"=w1794) -> ("Error Out"=w1797:errorcluster)  [unwired: 6 in, 1 out]
            }
            frame "GPS_NUMBER_ACTIVE_SAT" {
              # "колличество активных спутников GPS на Созвездии."
              n598 = Unbundle By Name(w1802) -> ("BASEBAND"=w1801:string)
              n599 = call "RS_SMBV100A_ASKCONFIGURATION.vi"("DriverConnect in"=w1806, "BASEBAND"=w1801) -> ("DriverConnect out"=w1805:T5, "Parsing Satelite"=w1800:T18, "Error Out"=w1804:errorcluster)  [unwired: 11 in]
              n600 = call "RS_SMBV100A_PARS_SAT_TIME_AND_NUMBER.vi"("Parsing Satelite"=w1800) -> ("OUT GPS NUMBERACTIVESAT"=w1803:dbl)  [unwired: 13 in, 5 out]
              n601 = Build Array(w1803) -> (w1807:dbl[])
              n602 = call "RS_SMBV100A_Error_check.vi"("Driver Name"=w1809, "Error Code"=w1810, "Error In"=w1804, "DriverConnect in"=w1805) -> ("Error Out"=w1808:errorcluster)  [unwired: 6 in, 1 out]
            }
            frame "GLONASS_NUMBER_ACTIVE_SAT" {
              # "колличество активных спутников GLONASS на Созвездии."
              n603 = Unbundle By Name(w1813) -> ("BASEBAND"=w1812:string)
              n604 = call "RS_SMBV100A_ASKCONFIGURATION.vi"("DriverConnect in"=w1817, "BASEBAND"=w1812) -> ("DriverConnect out"=w1816:T5, "Parsing Satelite"=w1811:T18, "Error Out"=w1815:errorcluster)  [unwired: 11 in]
              n605 = call "RS_SMBV100A_PARS_SAT_TIME_AND_NUMBER.vi"("Parsing Satelite"=w1811) -> ("OUT GLONASS NUMBERACTIVESAT"=w1814:dbl)  [unwired: 13 in, 5 out]
              n606 = Build Array(w1814) -> (w1818:dbl[])
              n607 = call "RS_SMBV100A_Error_check.vi"("Driver Name"=w1820, "Error Code"=w1821, "Error In"=w1815, "DriverConnect in"=w1816) -> ("Error Out"=w1819:errorcluster)  [unwired: 6 in, 1 out]
            }
            frame "GNSS_SAT_SORTED_MINTOMAX" {
              # "Массив порядка спутников(не номеров собственных) по времени от наименьшего времени"
              n608 = Unbundle By Name(w1824) -> ("BASEBAND"=w1823:string)
              n609 = call "RS_SMBV100A_ASKCONFIGURATION.vi"("DriverConnect in"=w1829, "BASEBAND"=w1823) -> ("DriverConnect out"=w1828:T5, "Parsing Satelite"=w1822:T18, "Error Out"=w1827:errorcluster)  [unwired: 11 in]
              n610 = call "RS_SMBV100A_PARS_SAT_TIME_AND_NUMBER.vi"("Parsing Satelite"=w1822) -> ("GNSS 2D SAT"=w1825:dbl[][])  [unwired: 13 in, 5 out]
              n611 = call "RS_SMBV100A_CONVERT_DATASAT_2D_to_N1D.vi"("2D DATA SAT"=w1825) -> ("GNSS_SatSortedMinToMax"=w1826:dbl[])  [unwired: 2 in, 5 out]
              n612 = call "RS_SMBV100A_Error_check.vi"("Driver Name"=w1831, "Error Code"=w1832, "Error In"=w1827, "DriverConnect in"=w1828) -> ("Error Out"=w1830:errorcluster)  [unwired: 6 in, 1 out]
            }
            frame "GPS_SAT_SORTED_MINTOMAX" {
              # "Массив порядка GPS спутников(не номеров собственных) по времени от наименьшего времени"
              n613 = Unbundle By Name(w1834) -> ("BASEBAND"=w1835:string)
              n614 = call "RS_SMBV100A_ASKCONFIGURATION.vi"("DriverConnect in"=w1840, "BASEBAND"=w1835) -> ("DriverConnect out"=w1839:T5, "Parsing Satelite"=w1833:T18, "Error Out"=w1838:errorcluster)  [unwired: 11 in]
              n615 = call "RS_SMBV100A_PARS_SAT_TIME_AND_NUMBER.vi"("Parsing Satelite"=w1833) -> ("GPS 2D SAT"=w1836:dbl[][])  [unwired: 13 in, 5 out]
              n616 = call "RS_SMBV100A_CONVERT_DATASAT_2D_to_N1D.vi"("2D DATA SAT"=w1836) -> ("GNSS_SatSortedMinToMax"=w1837:dbl[])  [unwired: 2 in, 5 out]
              n617 = call "RS_SMBV100A_Error_check.vi"("Driver Name"=w1842, "Error Code"=w1843, "Error In"=w1838, "DriverConnect in"=w1839) -> ("Error Out"=w1841:errorcluster)  [unwired: 6 in, 1 out]
            }
            frame "GLONASS_SAT_SORTED_MINTOMAX" {
              # "Массив порядка GLONASS спутников(не номеров собственных) по времени от наименьшего времени"
              n618 = Unbundle By Name(w1845) -> ("BASEBAND"=w1846:string)
              n619 = call "RS_SMBV100A_ASKCONFIGURATION.vi"("DriverConnect in"=w1851, "BASEBAND"=w1846) -> ("DriverConnect out"=w1850:T5, "Parsing Satelite"=w1844:T18, "Error Out"=w1849:errorcluster)  [unwired: 11 in]
              n620 = call "RS_SMBV100A_PARS_SAT_TIME_AND_NUMBER.vi"("Parsing Satelite"=w1844) -> ("GLONASS 2D SAT"=w1847:dbl[][])  [unwired: 13 in, 5 out]
              n621 = call "RS_SMBV100A_CONVERT_DATASAT_2D_to_N1D.vi"("2D DATA SAT"=w1847) -> ("GNSS_SatSortedMinToMax"=w1848:dbl[])  [unwired: 2 in, 5 out]
              n622 = call "RS_SMBV100A_Error_check.vi"("Driver Name"=w1853, "Error Code"=w1854, "Error In"=w1849, "DriverConnect in"=w1850) -> ("Error Out"=w1852:errorcluster)  [unwired: 6 in, 1 out]
            }
            frame "GNSS_TIME_SORTED_MINTOMAX" {
              # "Массив времен в секундах GNSS спутников - от наименьшего времени"
              n623 = Unbundle By Name(w1856) -> ("BASEBAND"=w1857:string)
              n624 = call "RS_SMBV100A_ASKCONFIGURATION.vi"("DriverConnect in"=w1862, "BASEBAND"=w1857) -> ("DriverConnect out"=w1861:T5, "Parsing Satelite"=w1855:T18, "Error Out"=w1860:errorcluster)  [unwired: 11 in]
              n625 = call "RS_SMBV100A_PARS_SAT_TIME_AND_NUMBER.vi"("Parsing Satelite"=w1855) -> ("GNSS 2D SAT"=w1859:dbl[][])  [unwired: 13 in, 5 out]
              n626 = call "RS_SMBV100A_CONVERT_DATASAT_2D_to_N1D.vi"("2D DATA SAT"=w1859) -> ("GNSS_TimeSortedMinToMax"=w1858:dbl[])  [unwired: 2 in, 5 out]
              n627 = call "RS_SMBV100A_Error_check.vi"("Driver Name"=w1864, "Error Code"=w1865, "Error In"=w1860, "DriverConnect in"=w1861) -> ("Error Out"=w1863:errorcluster)  [unwired: 6 in, 1 out]
            }
            frame "GPS_TIME_SORTED_MINTOMAX" {
              # "Массив времен в секундах GPS спутников - от наименьшего времени"
              n628 = Unbundle By Name(w1867) -> ("BASEBAND"=w1868:string)
              n629 = call "RS_SMBV100A_ASKCONFIGURATION.vi"("DriverConnect in"=w1873, "BASEBAND"=w1868) -> ("DriverConnect out"=w1872:T5, "Parsing Satelite"=w1866:T18, "Error Out"=w1871:errorcluster)  [unwired: 11 in]
              n630 = call "RS_SMBV100A_PARS_SAT_TIME_AND_NUMBER.vi"("Parsing Satelite"=w1866) -> ("GPS 2D SAT"=w1869:dbl[][])  [unwired: 13 in, 5 out]
              n631 = call "RS_SMBV100A_CONVERT_DATASAT_2D_to_N1D.vi"("2D DATA SAT"=w1869) -> ("GNSS_TimeSortedMinToMax"=w1870:dbl[])  [unwired: 2 in, 5 out]
              n632 = call "RS_SMBV100A_Error_check.vi"("Driver Name"=w1875, "Error Code"=w1876, "Error In"=w1871, "DriverConnect in"=w1872) -> ("Error Out"=w1874:errorcluster)  [unwired: 6 in, 1 out]
            }
            frame "GLONASS_TIME_SORTED_MINTOMAX" {
              # "Массив времен в секундах GLONASS спутников - от наименьшего времени"
              n633 = Unbundle By Name(w1878) -> ("BASEBAND"=w1879:string)
              n634 = call "RS_SMBV100A_ASKCONFIGURATION.vi"("DriverConnect in"=w1884, "BASEBAND"=w1879) -> ("DriverConnect out"=w1883:T5, "Parsing Satelite"=w1877:T18, "Error Out"=w1882:errorcluster)  [unwired: 11 in]
              n635 = call "RS_SMBV100A_PARS_SAT_TIME_AND_NUMBER.vi"("Parsing Satelite"=w1877) -> ("GLONASS 2D SAT"=w1880:dbl[][])  [unwired: 13 in, 5 out]
              n636 = call "RS_SMBV100A_CONVERT_DATASAT_2D_to_N1D.vi"("2D DATA SAT"=w1880) -> ("GNSS_TimeSortedMinToMax"=w1881:dbl[])  [unwired: 2 in, 5 out]
              n637 = call "RS_SMBV100A_Error_check.vi"("Driver Name"=w1886, "Error Code"=w1887, "Error In"=w1882, "DriverConnect in"=w1883) -> ("Error Out"=w1885:errorcluster)  [unwired: 6 in, 1 out]
            }
            frame "GNSS_SKY_SORTED_MINTOMAX" {
              # "Массив номеров GNSS спутников на небе - от наименьшего времени"
              n638 = Unbundle By Name(w1889) -> ("BASEBAND"=w1890:string)
              n639 = call "RS_SMBV100A_ASKCONFIGURATION.vi"("DriverConnect in"=w1895, "BASEBAND"=w1890) -> ("DriverConnect out"=w1894:T5, "Parsing Satelite"=w1888:T18, "Error Out"=w1893:errorcluster)  [unwired: 11 in]
              n640 = call "RS_SMBV100A_PARS_SAT_TIME_AND_NUMBER.vi"("Parsing Satelite"=w1888) -> ("GNSS 2D SAT"=w1891:dbl[][])  [unwired: 13 in, 5 out]
              n641 = call "RS_SMBV100A_CONVERT_DATASAT_2D_to_N1D.vi"("2D DATA SAT"=w1891) -> ("GNSS_SatSkySortedMinToMax"=w1892:dbl[])  [unwired: 2 in, 5 out]
              n642 = call "RS_SMBV100A_Error_check.vi"("Driver Name"=w1897, "Error Code"=w1898, "Error In"=w1893, "DriverConnect in"=w1894) -> ("Error Out"=w1896:errorcluster)  [unwired: 6 in, 1 out]
            }
            frame "GPS_SKY_SORTED_MINTOMAX" {
              # "Массив номеров GPS спутников на небе - от наименьшего времени"
              n643 = Unbundle By Name(w1900) -> ("BASEBAND"=w1901:string)
              n644 = call "RS_SMBV100A_ASKCONFIGURATION.vi"("DriverConnect in"=w1906, "BASEBAND"=w1901) -> ("DriverConnect out"=w1905:T5, "Parsing Satelite"=w1899:T18, "Error Out"=w1904:errorcluster)  [unwired: 11 in]
              n645 = call "RS_SMBV100A_PARS_SAT_TIME_AND_NUMBER.vi"("Parsing Satelite"=w1899) -> ("GPS 2D SAT"=w1902:dbl[][])  [unwired: 13 in, 5 out]
              n646 = call "RS_SMBV100A_CONVERT_DATASAT_2D_to_N1D.vi"("2D DATA SAT"=w1902) -> ("GNSS_SatSkySortedMinToMax"=w1903:dbl[])  [unwired: 2 in, 5 out]
              n647 = call "RS_SMBV100A_Error_check.vi"("Driver Name"=w1908, "Error Code"=w1909, "Error In"=w1904, "DriverConnect in"=w1905) -> ("Error Out"=w1907:errorcluster)  [unwired: 6 in, 1 out]
            }
            frame "GLONASS_SKY_SORTED_MINTOMAX" {
              # "Массив номеров GLONASS спутников на небе - от наименьшего времени"
              n648 = Unbundle By Name(w1911) -> ("BASEBAND"=w1912:string)
              n649 = call "RS_SMBV100A_ASKCONFIGURATION.vi"("DriverConnect in"=w1917, "BASEBAND"=w1912) -> ("DriverConnect out"=w1916:T5, "Parsing Satelite"=w1910:T18, "Error Out"=w1915:errorcluster)  [unwired: 11 in]
              n650 = call "RS_SMBV100A_PARS_SAT_TIME_AND_NUMBER.vi"("Parsing Satelite"=w1910) -> ("GLONASS 2D SAT"=w1913:dbl[][])  [unwired: 13 in, 5 out]
              n651 = call "RS_SMBV100A_CONVERT_DATASAT_2D_to_N1D.vi"("2D DATA SAT"=w1913) -> ("GNSS_SatSkySortedMinToMax"=w1914:dbl[])  [unwired: 2 in, 5 out]
              n652 = call "RS_SMBV100A_Error_check.vi"("Driver Name"=w1919, "Error Code"=w1920, "Error In"=w1915, "DriverConnect in"=w1916) -> ("Error Out"=w1918:errorcluster)  [unwired: 6 in, 1 out]
            }
            frame "GNSS_SAT_SORTED_MAXTOMIN" {
              # "Массив порядка спутников(не номеров собственных) по времени от наибольшего времени"
              n653 = Unbundle By Name(w1922) -> ("BASEBAND"=w1923:string)
              n654 = call "RS_SMBV100A_ASKCONFIGURATION.vi"("DriverConnect in"=w1928, "BASEBAND"=w1923) -> ("DriverConnect out"=w1927:T5, "Parsing Satelite"=w1921:T18, "Error Out"=w1926:errorcluster)  [unwired: 11 in]
              n655 = call "RS_SMBV100A_PARS_SAT_TIME_AND_NUMBER.vi"("Parsing Satelite"=w1921) -> ("GNSS 2D SAT"=w1925:dbl[][])  [unwired: 13 in, 5 out]
              n656 = call "RS_SMBV100A_CONVERT_DATASAT_2D_to_N1D.vi"("2D DATA SAT"=w1925) -> ("GNSS_SatSortedMaxToMin"=w1924:dbl[])  [unwired: 2 in, 5 out]
              n657 = call "RS_SMBV100A_Error_check.vi"("Driver Name"=w1930, "Error Code"=w1931, "Error In"=w1926, "DriverConnect in"=w1927) -> ("Error Out"=w1929:errorcluster)  [unwired: 6 in, 1 out]
            }
            frame "GPS_SAT_SORTED_MAXTOMIN" {
              # "Массив порядка GPS спутников(не номеров собственных) по времени от наибольшего времени"
              n658 = Unbundle By Name(w1933) -> ("BASEBAND"=w1934:string)
              n659 = call "RS_SMBV100A_ASKCONFIGURATION.vi"("DriverConnect in"=w1939, "BASEBAND"=w1934) -> ("DriverConnect out"=w1938:T5, "Parsing Satelite"=w1932:T18, "Error Out"=w1937:errorcluster)  [unwired: 11 in]
              n660 = call "RS_SMBV100A_PARS_SAT_TIME_AND_NUMBER.vi"("Parsing Satelite"=w1932) -> ("GPS 2D SAT"=w1935:dbl[][])  [unwired: 13 in, 5 out]
              n661 = call "RS_SMBV100A_CONVERT_DATASAT_2D_to_N1D.vi"("2D DATA SAT"=w1935) -> ("GNSS_SatSortedMaxToMin"=w1936:dbl[])  [unwired: 2 in, 5 out]
              n662 = call "RS_SMBV100A_Error_check.vi"("Driver Name"=w1941, "Error Code"=w1942, "Error In"=w1937, "DriverConnect in"=w1938) -> ("Error Out"=w1940:errorcluster)  [unwired: 6 in, 1 out]
            }
            frame "GLONASS_SAT_SORTED_MAXTOMIN" {
              # "Массив порядка GLONASS спутников(не номеров собственных) по времени от наибольшего времени"
              n663 = Unbundle By Name(w1944) -> ("BASEBAND"=w1945:string)
              n664 = call "RS_SMBV100A_ASKCONFIGURATION.vi"("DriverConnect in"=w1950, "BASEBAND"=w1945) -> ("DriverConnect out"=w1949:T5, "Parsing Satelite"=w1943:T18, "Error Out"=w1948:errorcluster)  [unwired: 11 in]
              n665 = call "RS_SMBV100A_PARS_SAT_TIME_AND_NUMBER.vi"("Parsing Satelite"=w1943) -> ("GLONASS 2D SAT"=w1946:dbl[][])  [unwired: 13 in, 5 out]
              n666 = call "RS_SMBV100A_CONVERT_DATASAT_2D_to_N1D.vi"("2D DATA SAT"=w1946) -> ("GNSS_SatSortedMaxToMin"=w1947:dbl[])  [unwired: 2 in, 5 out]
              n667 = call "RS_SMBV100A_Error_check.vi"("Driver Name"=w1952, "Error Code"=w1953, "Error In"=w1948, "DriverConnect in"=w1949) -> ("Error Out"=w1951:errorcluster)  [unwired: 6 in, 1 out]
            }
            frame "GNSS_TIME_SORTED_MAXTOMIN" {
              # "Массив времен в секундах GNSS спутников- по времени от наибольшего времени"
              n668 = Unbundle By Name(w1955) -> ("BASEBAND"=w1956:string)
              n669 = call "RS_SMBV100A_ASKCONFIGURATION.vi"("DriverConnect in"=w1961, "BASEBAND"=w1956) -> ("DriverConnect out"=w1960:T5, "Parsing Satelite"=w1954:T18, "Error Out"=w1959:errorcluster)  [unwired: 11 in]
              n670 = call "RS_SMBV100A_PARS_SAT_TIME_AND_NUMBER.vi"("Parsing Satelite"=w1954) -> ("GNSS 2D SAT"=w1957:dbl[][])  [unwired: 13 in, 5 out]
              n671 = call "RS_SMBV100A_CONVERT_DATASAT_2D_to_N1D.vi"("2D DATA SAT"=w1957) -> ("GNSS_TimeSortedMaxToMin"=w1958:dbl[])  [unwired: 2 in, 5 out]
              n672 = call "RS_SMBV100A_Error_check.vi"("Driver Name"=w1963, "Error Code"=w1964, "Error In"=w1959, "DriverConnect in"=w1960) -> ("Error Out"=w1962:errorcluster)  [unwired: 6 in, 1 out]
            }
            frame "GPS_TIME_SORTED_MAXTOMIN" {
              # "Массив времен в секундах GPS спутников- по времени от наибольшего времени"
              n673 = Unbundle By Name(w1966) -> ("BASEBAND"=w1967:string)
              n674 = call "RS_SMBV100A_ASKCONFIGURATION.vi"("DriverConnect in"=w1972, "BASEBAND"=w1967) -> ("DriverConnect out"=w1971:T5, "Parsing Satelite"=w1965:T18, "Error Out"=w1970:errorcluster)  [unwired: 11 in]
              n675 = call "RS_SMBV100A_PARS_SAT_TIME_AND_NUMBER.vi"("Parsing Satelite"=w1965) -> ("GPS 2D SAT"=w1968:dbl[][])  [unwired: 13 in, 5 out]
              n676 = call "RS_SMBV100A_CONVERT_DATASAT_2D_to_N1D.vi"("2D DATA SAT"=w1968) -> ("GNSS_TimeSortedMaxToMin"=w1969:dbl[])  [unwired: 2 in, 5 out]
              n677 = call "RS_SMBV100A_Error_check.vi"("Driver Name"=w1974, "Error Code"=w1975, "Error In"=w1970, "DriverConnect in"=w1971) -> ("Error Out"=w1973:errorcluster)  [unwired: 6 in, 1 out]
            }
            frame "GLONASS_TIME_SORTED_MAXTOMIN" {
              # "Массив времен в секундах GLONASS спутников- по времени от наибольшего времени"
              n678 = Unbundle By Name(w1977) -> ("BASEBAND"=w1978:string)
              n679 = call "RS_SMBV100A_ASKCONFIGURATION.vi"("DriverConnect in"=w1983, "BASEBAND"=w1978) -> ("DriverConnect out"=w1982:T5, "Parsing Satelite"=w1976:T18, "Error Out"=w1981:errorcluster)  [unwired: 11 in]
              n680 = call "RS_SMBV100A_PARS_SAT_TIME_AND_NUMBER.vi"("Parsing Satelite"=w1976) -> ("GLONASS 2D SAT"=w1979:dbl[][])  [unwired: 13 in, 5 out]
              n681 = call "RS_SMBV100A_CONVERT_DATASAT_2D_to_N1D.vi"("2D DATA SAT"=w1979) -> ("GNSS_TimeSortedMaxToMin"=w1980:dbl[])  [unwired: 2 in, 5 out]
              n682 = call "RS_SMBV100A_Error_check.vi"("Driver Name"=w1985, "Error Code"=w1986, "Error In"=w1981, "DriverConnect in"=w1982) -> ("Error Out"=w1984:errorcluster)  [unwired: 6 in, 1 out]
            }
            frame "GNSS_SKY_SORTED_MAXTOMIN" {
              # "Массив номеров GNSS спутников на небе - по времени от наибольшего времени"
              n683 = Unbundle By Name(w1988) -> ("BASEBAND"=w1989:string)
              n684 = call "RS_SMBV100A_ASKCONFIGURATION.vi"("DriverConnect in"=w1996, "BASEBAND"=w1989) -> ("DriverConnect out"=w1993:T5, "Parsing Satelite"=w1987:T18, "Error Out"=w1992:errorcluster)  [unwired: 11 in]
              n685 = call "RS_SMBV100A_PARS_SAT_TIME_AND_NUMBER.vi"("Parsing Satelite"=w1987) -> ("GNSS 2D SAT"=w1991:dbl[][])  [unwired: 13 in, 5 out]
              n686 = call "RS_SMBV100A_CONVERT_DATASAT_2D_to_N1D.vi"("2D DATA SAT"=w1991) -> ("GNSS_SatSkySortedMaxToMin"=w1995:dbl[])  [unwired: 2 in, 5 out]
              n687 = call "RS_SMBV100A_Error_check.vi"("Driver Name"=w1997, "Error Code"=w1998, "Error In"=w1992, "DriverConnect in"=w1993) -> ("Error Out"=w1990:errorcluster)  [unwired: 6 in, 1 out]
              n688 = call "MLLF_ParsingIntArrayToString (SubVI).vi"("Value"=w1995) -> ("String"=w1994:string)  [unwired: 10 in]
            }
            frame "GPS_SKY_SORTED_MAXTOMIN" {
              # "Массив номеров GPS спутников на небе - по времени от наибольшего времени"
              n689 = Unbundle By Name(w2000) -> ("BASEBAND"=w2001:string)
              n690 = call "RS_SMBV100A_ASKCONFIGURATION.vi"("DriverConnect in"=w2006, "BASEBAND"=w2001) -> ("DriverConnect out"=w2005:T5, "Parsing Satelite"=w1999:T18, "Error Out"=w2004:errorcluster)  [unwired: 11 in]
              n691 = call "RS_SMBV100A_PARS_SAT_TIME_AND_NUMBER.vi"("Parsing Satelite"=w1999) -> ("GPS 2D SAT"=w2002:dbl[][])  [unwired: 13 in, 5 out]
              n692 = call "RS_SMBV100A_CONVERT_DATASAT_2D_to_N1D.vi"("2D DATA SAT"=w2002) -> ("GNSS_SatSkySortedMaxToMin"=w2003:dbl[])  [unwired: 2 in, 5 out]
              n693 = call "RS_SMBV100A_Error_check.vi"("Driver Name"=w2008, "Error Code"=w2009, "Error In"=w2004, "DriverConnect in"=w2005) -> ("Error Out"=w2007:errorcluster)  [unwired: 6 in, 1 out]
            }
            frame "GLONASS_SKY_SORTED_MAXTOMIN" {
              # "Массив номеров GLONASS спутников на небе - по времени от наибольшего времени"
              n694 = Unbundle By Name(w2011) -> ("BASEBAND"=w2012:string)
              n695 = call "RS_SMBV100A_ASKCONFIGURATION.vi"("DriverConnect in"=w2017, "BASEBAND"=w2012) -> ("DriverConnect out"=w2016:T5, "Parsing Satelite"=w2010:T18, "Error Out"=w2015:errorcluster)  [unwired: 11 in]
              n696 = call "RS_SMBV100A_PARS_SAT_TIME_AND_NUMBER.vi"("Parsing Satelite"=w2010) -> ("GLONASS 2D SAT"=w2013:dbl[][])  [unwired: 13 in, 5 out]
              n697 = call "RS_SMBV100A_CONVERT_DATASAT_2D_to_N1D.vi"("2D DATA SAT"=w2013) -> ("GNSS_SatSkySortedMaxToMin"=w2014:dbl[])  [unwired: 2 in, 5 out]
              n698 = call "RS_SMBV100A_Error_check.vi"("Driver Name"=w2019, "Error Code"=w2020, "Error In"=w2015, "DriverConnect in"=w2016) -> ("Error Out"=w2018:errorcluster)  [unwired: 6 in, 1 out]
            }
          }
          n699 = call "MLLF_FormatOutputValueWithUnits.vi"("Lower limit"=-1e+32, "Upper limit"=1e+32, "error in"=w1147, "ValuesIn"=w1149) -> ("error out"=w1142:T15, "Result string"=w1150:T16)  [unwired: 6 in]
          n700 = Concatenate Strings(w1150, w1144) -> (w1143:string)
        }
        frame "close" {
          # "Завершение сессии"
          n701 = Unbundle By Name(w2022) -> ("Connect.OpenedSession"=w2024:T7)
          n702 = VISA Close(VISA resource name=w2024) -> (error out=w2023:errorcluster)  [unwired: 1 in]
        }
      }
    }
    frame Error {
    }
  }
  n703 = local write "Settings"(w4) -> ()
  n704 = flat-sequence {
    tunnel: [w2033] -> w12
    tunnel: w15 -> [w2032]
    tunnel: w13 -> [w2027]
    tunnel: w14 -> [w2028]
    tunnel: [w2028] -> w10
    tunnel: [w2029] -> w11
    frame #0 {
      # "driver out"
      n705 = Unbundle By Name(w2028) -> ("Connect"=w2031:T5)
      n706 = call "MLLF_SaveLastSetting.vi"("error in"=w2027, "DriverConnectCluster in"=w2031) -> ("error out"=w2030:T15)  [unwired: 8 in, 1 out]
      n707 = call "MCF_Output.vi"("Error In"=w2030, "Input"=w2032) -> ("Error Out"=w2029:errorcluster, "Output"=w2033:string)  [unwired: 8 in]
    }
  }
  n708 = local write "Settings"(w10) -> ()
  "error out" <- w11
  "Response" <- w12
